vi "Autonomous Independent.vi"   [LabVIEW 2017]
doc: "This VI is called when autonomous begins, and will automatically be terminated when autonomous ends. You can carry out timed or sensor driven robot movement independently without needing to return to the caller."
uses:
  <vilib>/Rock Robotics/WPI/ThirdParty/Phoenix-LabVIEW/Motor Controller/Controls/CTRE_Phoenix_MotorControl_RemoteSourceType.ctl
  <vilib>/Rock Robotics/WPI/ThirdParty/Phoenix-LabVIEW/Motor Controller/Controls/CTRE_Phoenix_MotorControl_ControlMode.ctl
  <vilib>/Rock Robotics/WPI/Utilities/WPI_GetSetVariantRefNum.vi
  <vilib>/Rock Robotics/Network Tables/NT Read String.vi
  Robot Global Data.vi
  <vilib>/Rock Robotics/WPI/RobotDrive/WPI_RobotDriveArcadeDrive_Standard(NoSaturation).vi
  <vilib>/Rock Robotics/WPI/ThirdParty/Phoenix-LabVIEW/Motor Controller/Get/CTRE_Phoenix_MotorController_GetPulseWidthAll.vi
panel:
  # "Be sure to right-click and choose Data Operations>>Make Current Value default if you want to save the array values with the VI"
types:
  T1 = typedef "CTRE_Phoenix_MotorControl_RemoteSourceType.ctl" = enum16{"Off", "Talon SRX Selected Sensor", "Pigeon IMU Yaw", "Pigeon IMU Pitch", "Pigeon IMU Roll", "CANifier Quadrature", "CANifier PWM Input 0", "CANifier PWM Input 1", "CANifier PWM Input 2", "CANifier PWM Input 3", "Gadgeteer Pigeon Yaw", "Gadgeteer Pigeon Pitch", "Gadgeteer Pigeon Roll"}
  T2 = typedef "WPI_MotorControlDeviceRef.ctl" = cluster{"DeviceStatus":errorcluster, "Type":T3, "PWM":cluster{"PWM Channel":T4, "DeadBand":T5}, "CAN":cluster{"Device Number":u8, "SetOutput VI Ref":variant, "GetOutput VI Ref":variant, "Enable VI Ref":variant, "Disable VI Ref":variant, "Data":variant}, "Invert":bool, "DIO PWM":cluster{"PWM \"Enable\" Channel":T4, "DIOChannel":T6, "PWM Rate":dbl}}
  T3 = typedef "WPI_MotorControlType.ctl" = enum16{"PWM", "CAN", "DIO PWM"}
  T4 = typedef "FPGA_DIOPWMChannel.ctl" = enum8{"PWM 0", "PWM 1", "PWM 2", "PWM 3", "PWM 4", "PWM 5", "PWM 6", "PWM 7", "PWM 8", "PWM 9", "PWM MXP 0", "PWM MXP 1", "PWM MXP 2", "PWM MXP 3", "PWM MXP 4", "PWM MXP 5", "PWM MXP 6", "PWM MXP 7", "PWM MXP 8", "PWM MXP 9", "Invalid"}
  T5 = typedef "WPI_PWMDeadband.ctl" = cluster{"Name":string, "maxPositivePwm":i32, "minPositivePwm":i32, "centerPwm":i32, "maxNegativePwm":i32, "minNegativePwm":i32, "angularRange":u16}
  T6 = typedef "FPGA_DIOChannel.ctl" = enum8{"DIO 0", "DIO 1", "DIO 2", "DIO 3", "DIO 4", "DIO 5", "DIO 6", "DIO 7", "DIO 8", "DIO 9", "DIO MXP 0", "DIO MXP 1", "DIO MXP 2", "DIO MXP 3", "DIO MXP 4", "DIO MXP 5", "DIO MXP 6", "DIO MXP 7", "DIO MXP 8", "DIO MXP 9", "DIO MXP 10", "DIO MXP 11", "DIO MXP 12", "DIO MXP 13", "DIO MXP 14", "DIO MXP 15", "SPI Port CS1", "SPI Port CS2", "SPI Port CS3", "SPI Port MISO", "SPI Port MOSI", "Invalid"}
  T7 = typedef "WPI_AnalogChannelDevRef.ctl" = cluster{"DevStatus":errorcluster, "Analog Channel":T8}
  T8 = typedef "FPGA_AIChannel.ctl" = enum8{"AI 0", "AI 1", "AI 2", "AI 3", "AI MXP 0", "AI MXP 1", "AI MXP 2", "AI MXP 3", "Invalid"}
  T9 = typedef "WPI_SwitchDevRef.ctl" = cluster{"DevStatus":errorcluster, "DIO Channel":T6, "CntIndex":T10, "Normally Closed":bool}
  T10 = typedef "FPGA_CounterCtrSystemIndex.ctl" = enum8{"Ctr 0", "Ctr 1", "Ctr 2", "Ctr 3", "Ctr 4", "Ctr 5", "Ctr 6", "Ctr 7", "Invalid"}
  T11 = typedef "WPI_RobotDriveDevRef.ctl" = cluster{"DevStatus":errorcluster, "Motors[]":T2[], "Square Inputs":bool, "Max Output":dbl}
  T12 = typedef "CTRE_Phoenix_MotorControl_ControlMode.ctl" = u16
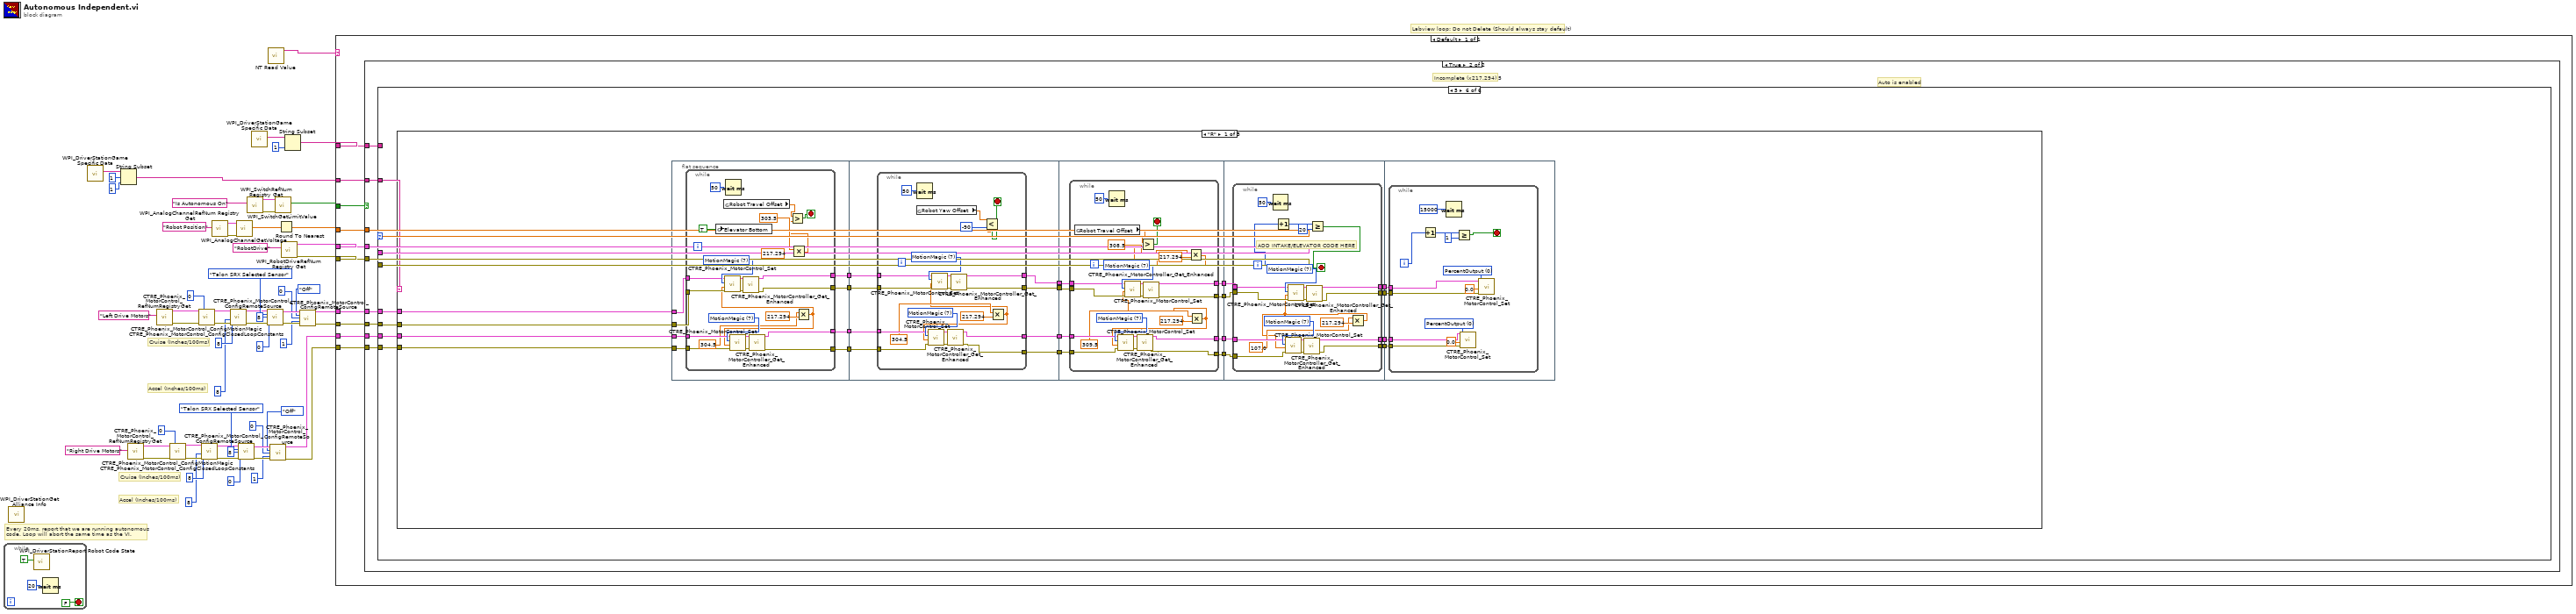
[diagram p0: block diagram]
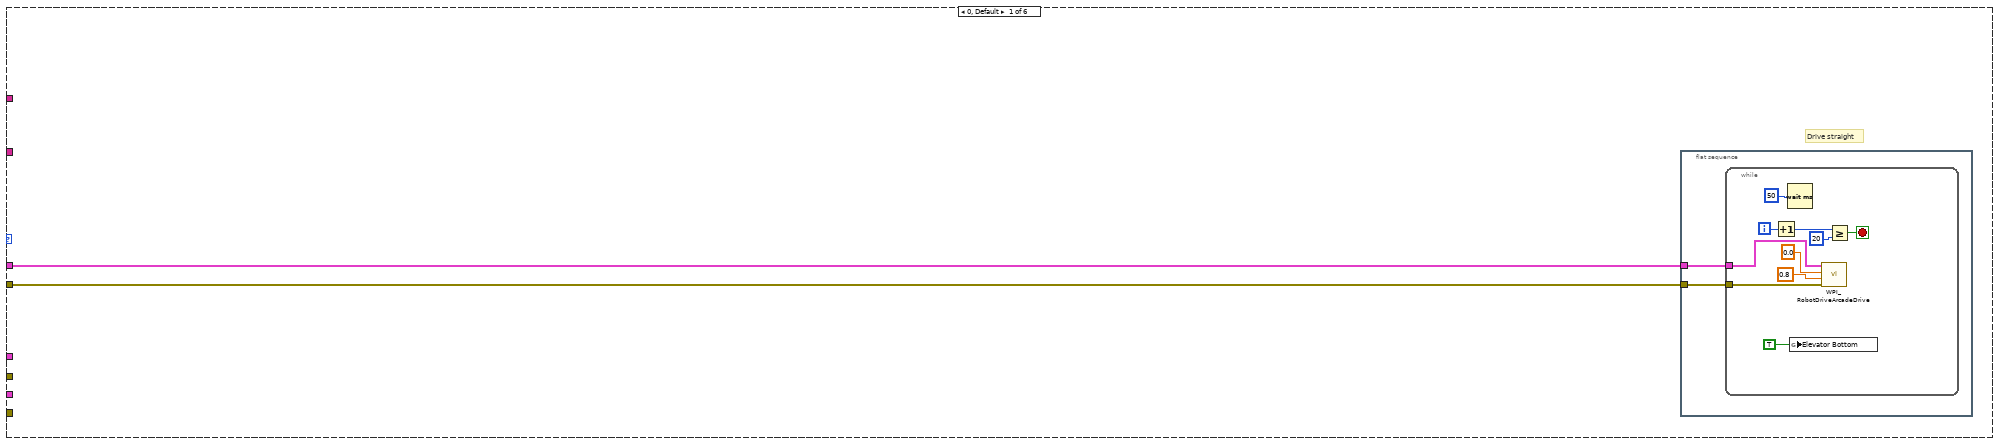
[diagram p3: hidden frame]
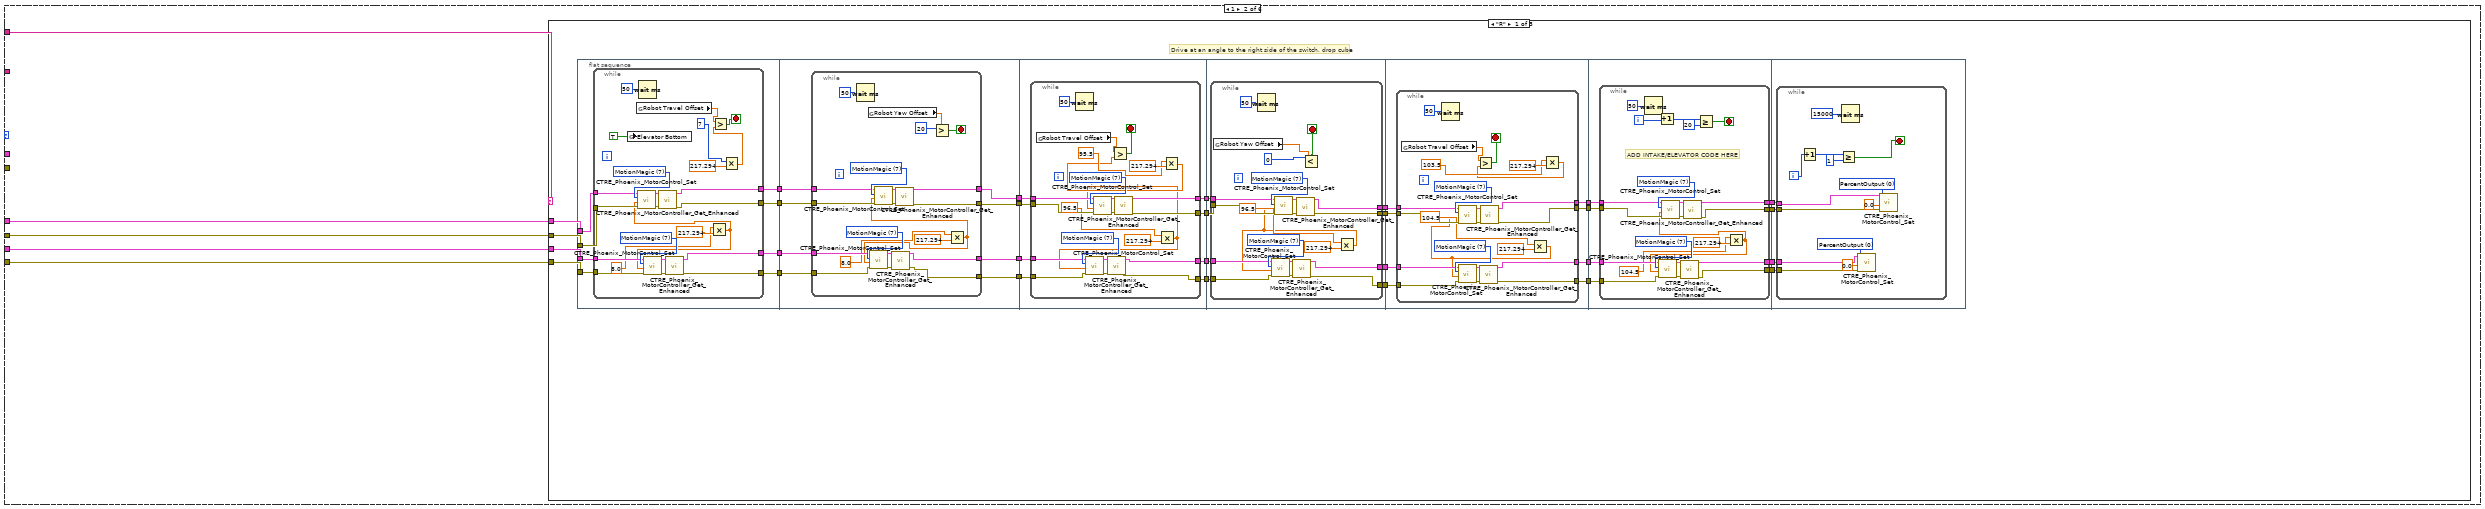
[diagram p4: hidden frame]
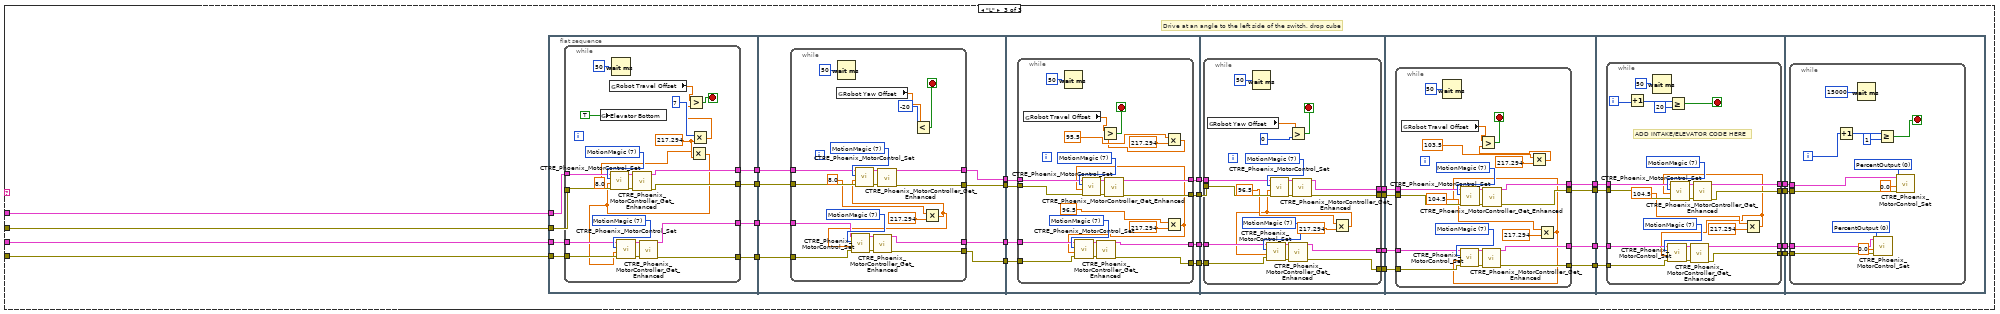
[diagram p6: hidden frame]
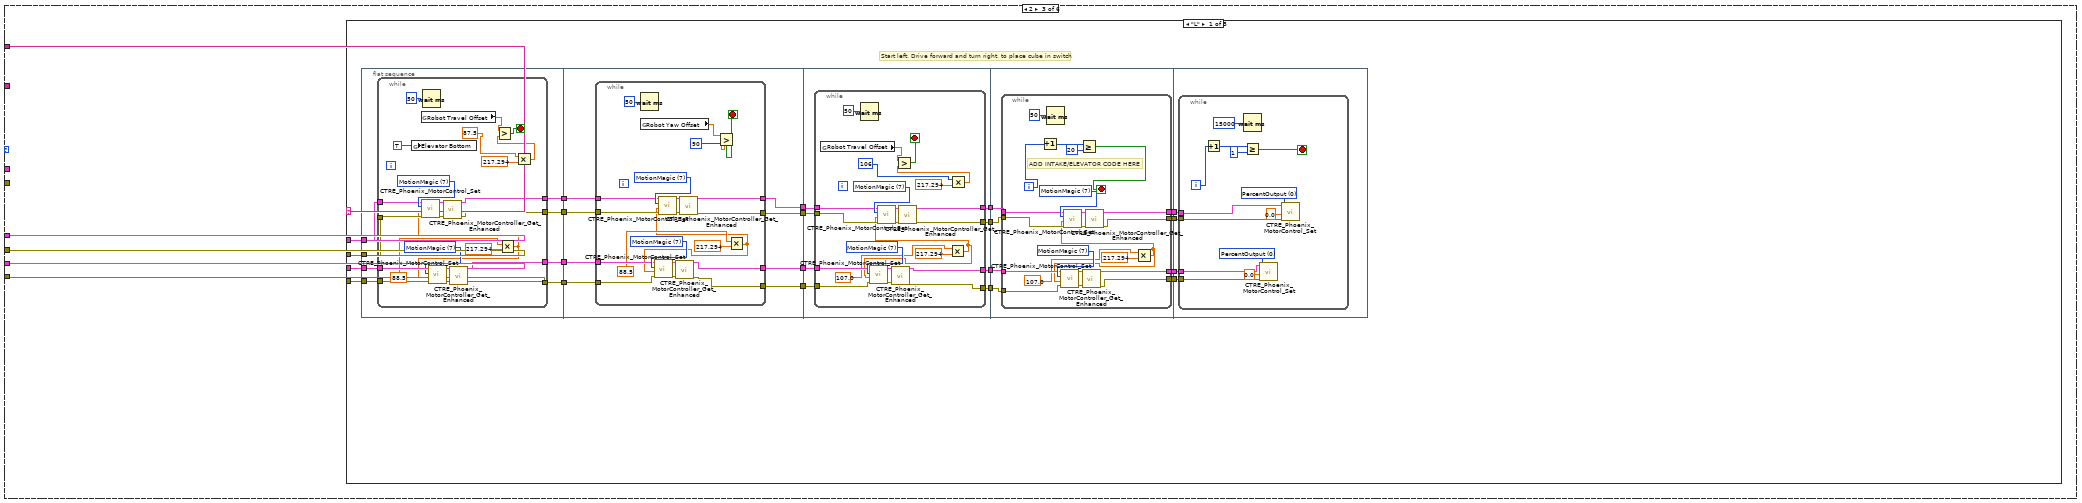
[diagram p7: hidden frame]
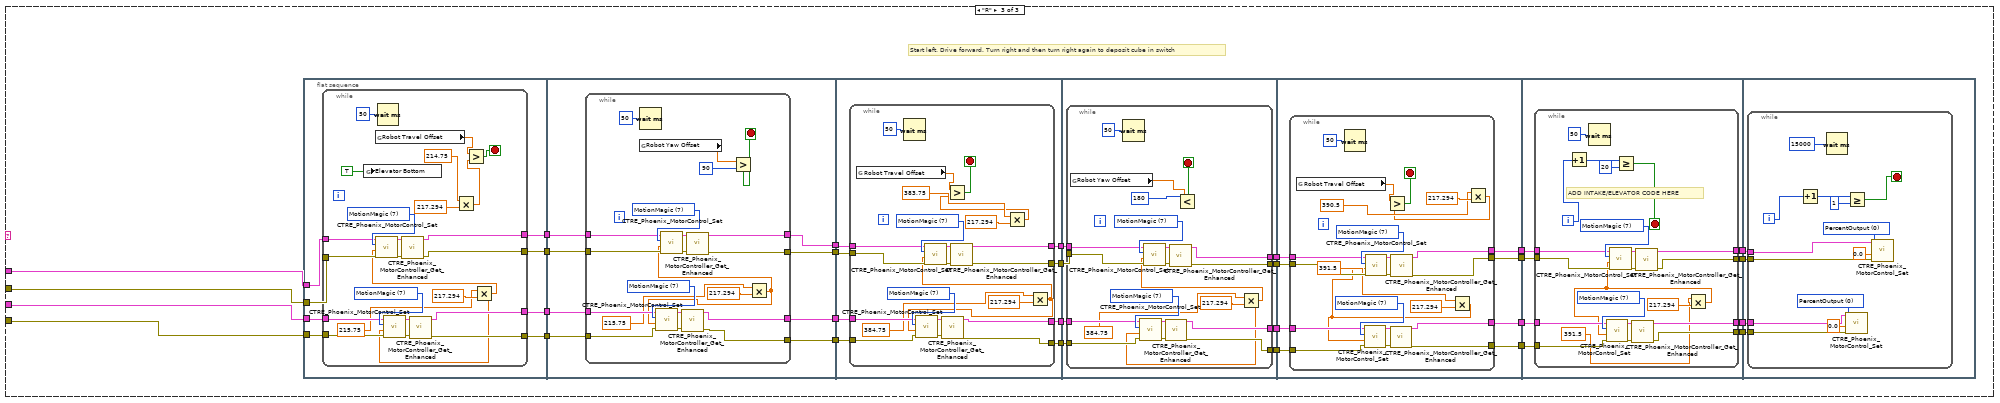
[diagram p9: hidden frame]
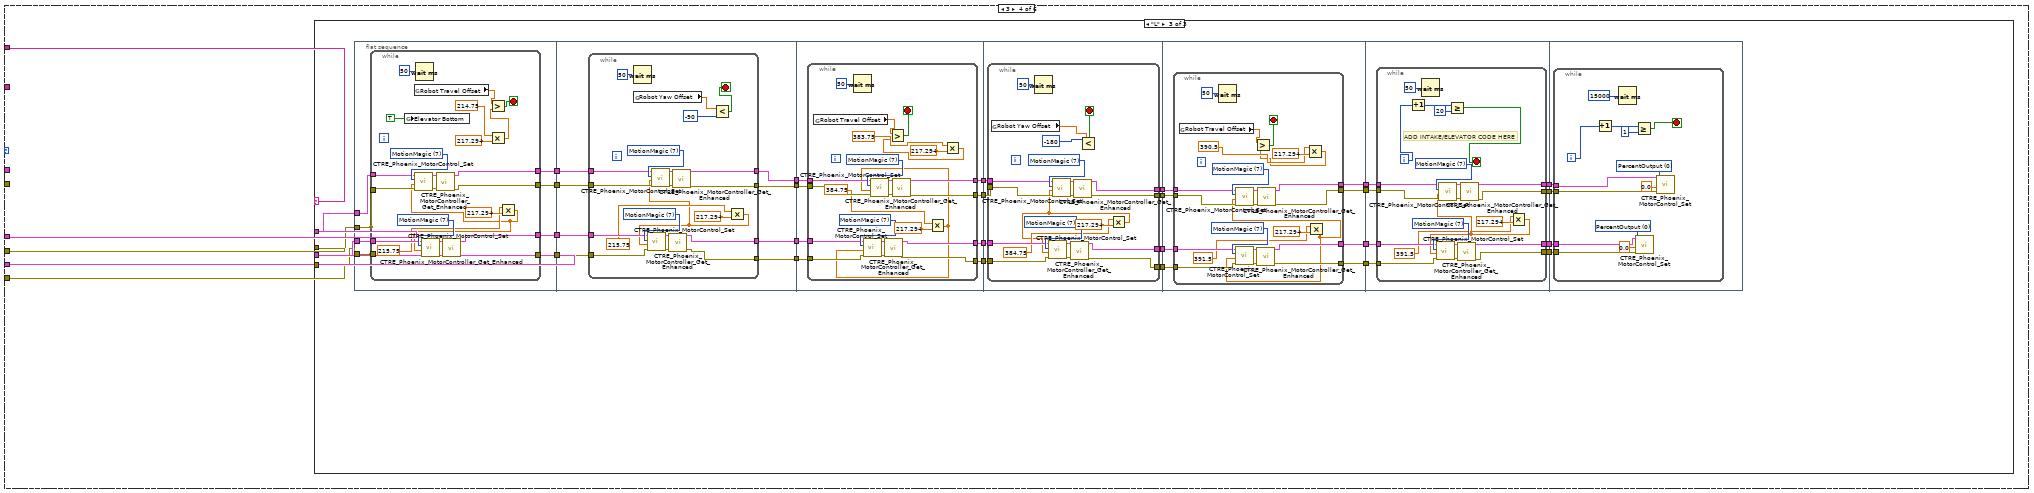
[diagram p10: hidden frame]
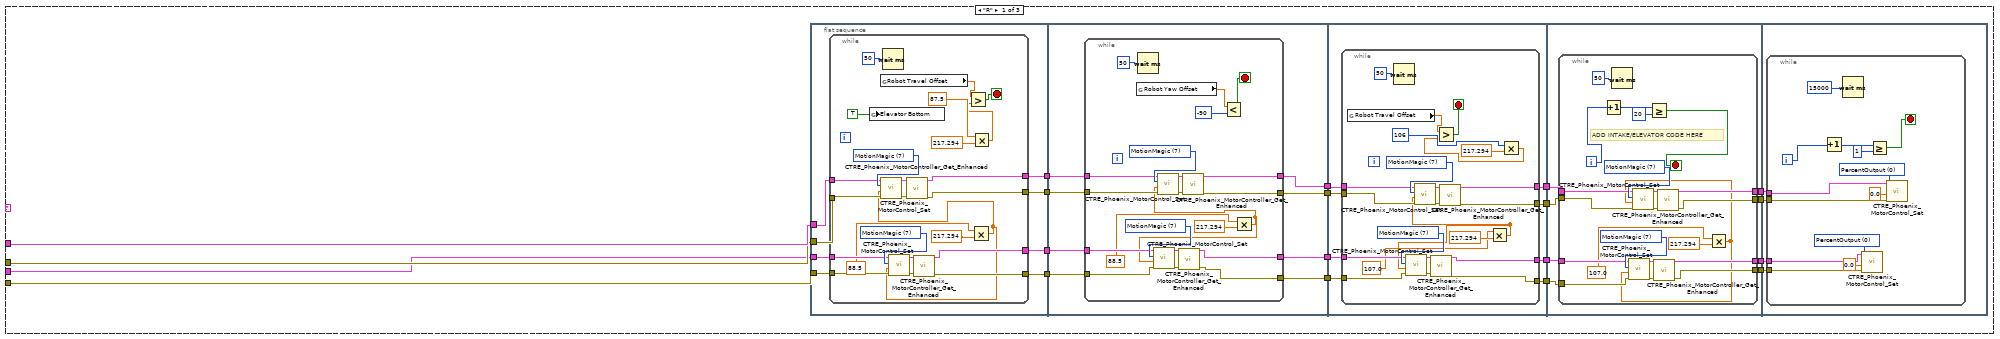
[diagram p11: hidden frame]
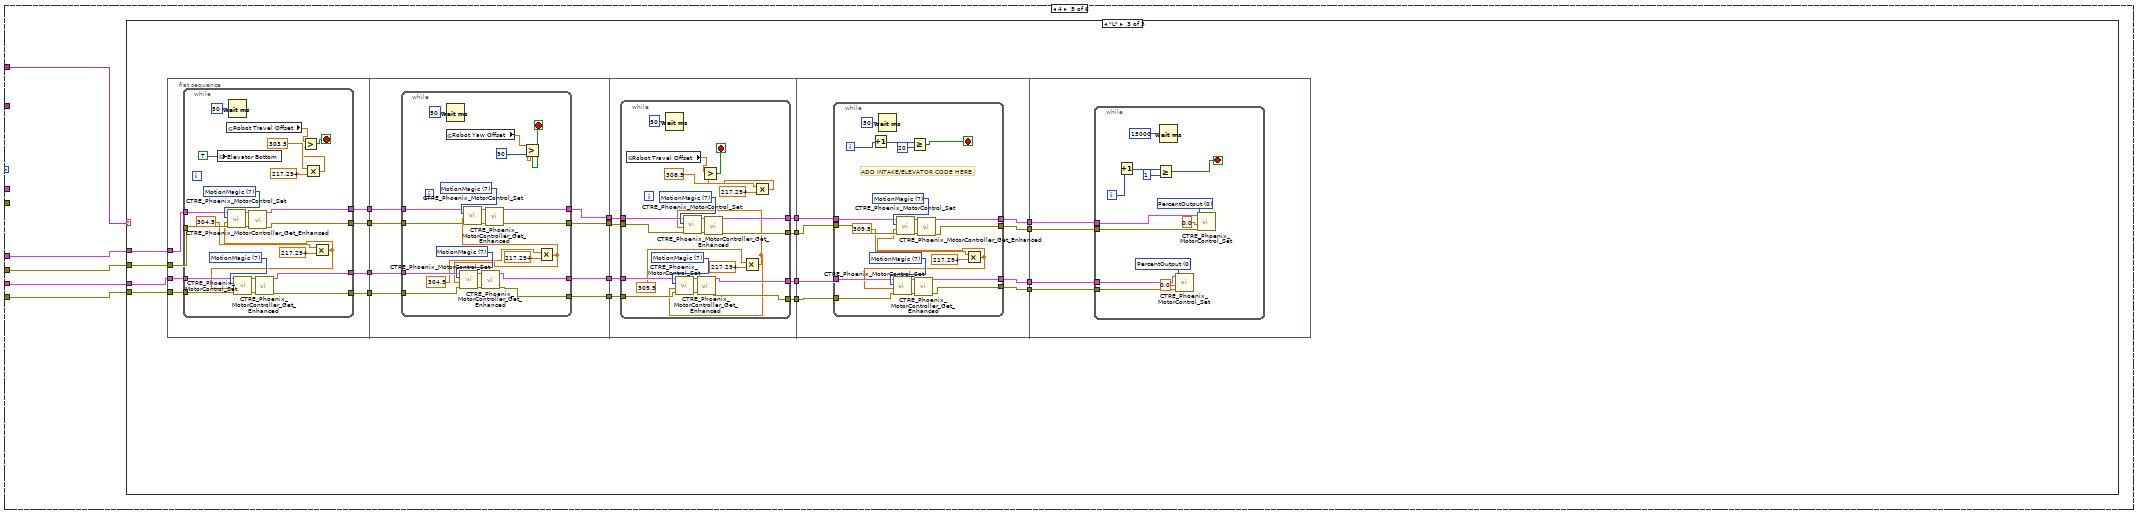
[diagram p13: hidden frame]
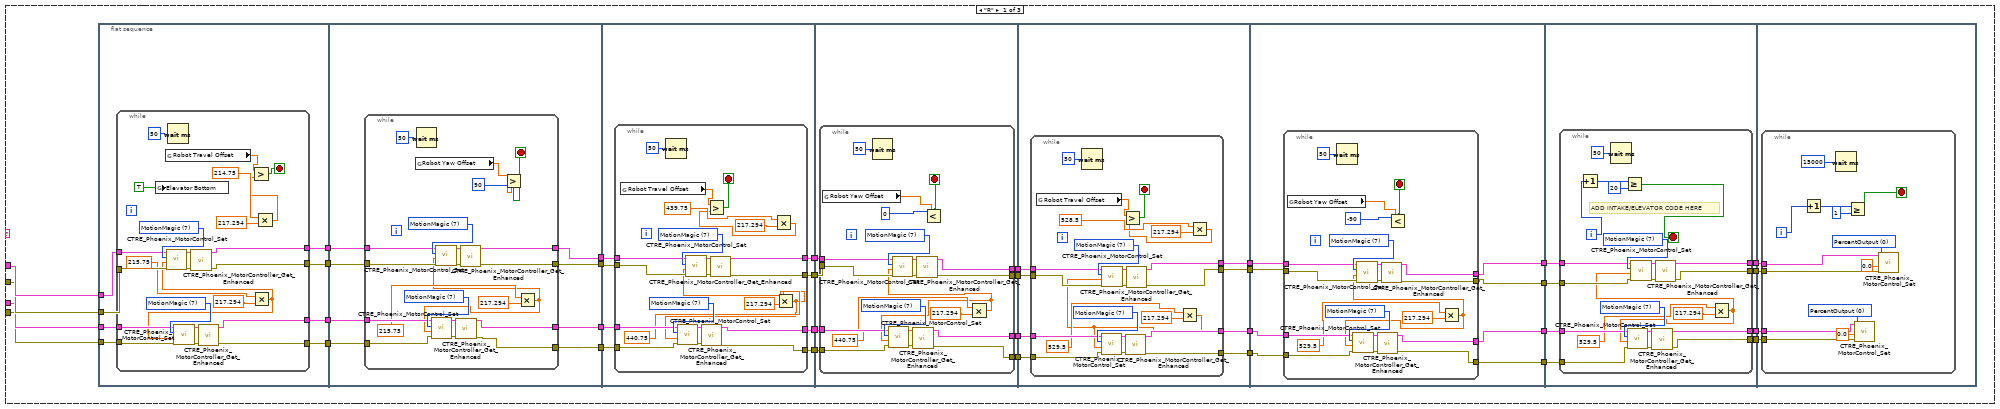
[diagram p14: hidden frame]
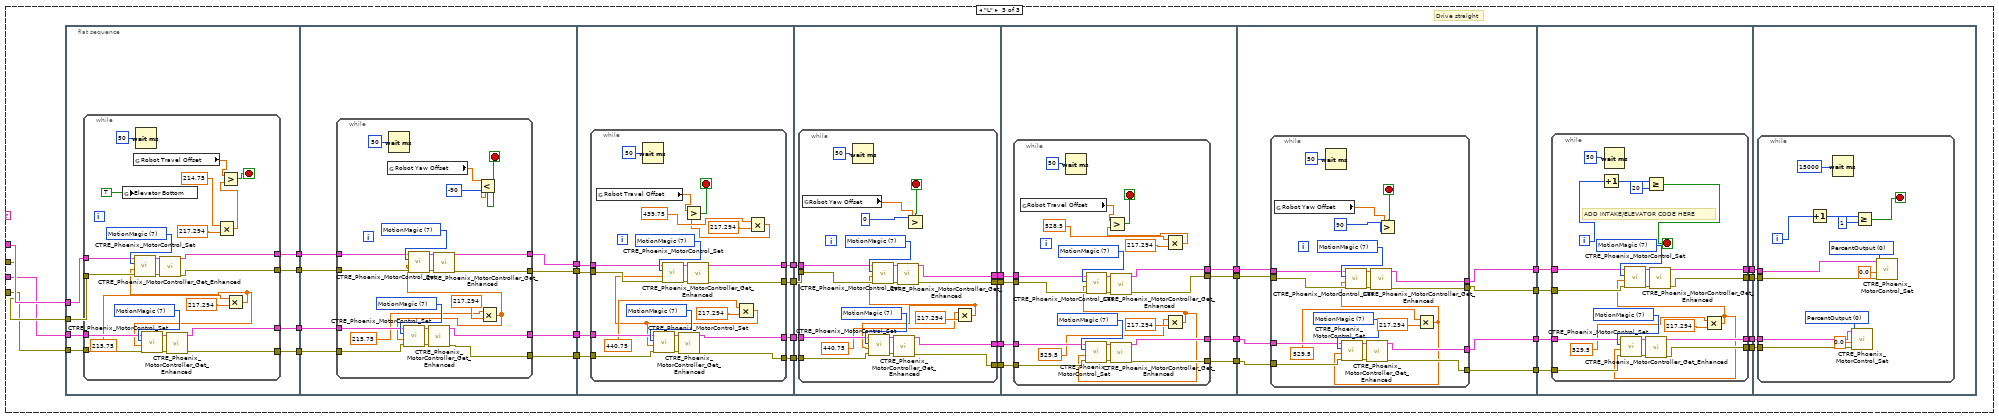
[diagram p17: hidden frame]
diagram:
  # "Cruise (Inches/100ms)"
  # "Accel (Inches/100ms)"
  # "Cruise (Inches/100ms)"
  # "Accel (Inches/100ms)"
  # "Labview loop: Do not Delete (Should always stay default)"
  # "Every 20ms, report that we are running autonomous\ncode. Loop will abort the same time as the VI."
  n1 = while {
    stop <- FALSE stop-if-true
    n2 = call <vilib>:"WPI_DriverStationReport Robot Code State.vi"("Autonomous"=TRUE) -> ()  [unwired: 10 in, 1 out]
    n3 = Wait (ms)(milliseconds to wait=u32 20) -> ()  [unwired: 1 out]
  }
  n4 = call <vilib>:"WPI_DriverStationGet Alliance Info.vi"() -> ()  [unwired: 12 out]
  n5 = call <vilib>:"WPI_DriverStationGame Specific Data.vi"() -> ("Game Specific Data"=w51:string)  [unwired: 11 in]
  n6 = String Subset(string=w51, offset (0)=1, length (rest)=1 ("length (rest)")) -> (substring=w50:string)
  n7 = call <vilib>:"CTRE_Phoenix_MotorControl_RefNumRegistryGet.vi"("refnum name"="Right Drive Motors") -> ("error out"=w19:errorcluster, "PhoenixMotorControlDevRef"=w17:T2)  [unwired: 9 in]
  n8 = call <vilib>:"CTRE_Phoenix_MotorControl_RefNumRegistryGet.vi"("refnum name"="Left Drive Motors") -> ("error out"=w39:errorcluster, "PhoenixMotorControlDevRef"=w37:T2)  [unwired: 9 in]
  n9 = call <vilib>:"CTRE_Phoenix_MotorControl_ConfigClosedLoopConstants.vi"("PhoenixMotorControlDevRef"=w17, "slotIdx"=0, "error in (no error)"=w19) -> ("PhoenixMotorControlDevRef"=w16:T2, "error out"=w18:errorcluster)  [unwired: 11 in]
  n10 = call <vilib>:"CTRE_Phoenix_MotorControl_ConfigClosedLoopConstants.vi"("PhoenixMotorControlDevRef"=w37, "slotIdx"=0, "error in (no error)"=w39) -> ("PhoenixMotorControlDevRef"=w36:T2, "error out"=w38:errorcluster)  [unwired: 11 in]
  n11 = call <vilib>:"CTRE_Phoenix_MotorControl_ConfigMotionMagic.vi"("error in (no error)"=w18, "Acceleration"=8, "Cruise Velocity"=8, "PhoenixMotorControlDevRef"=w16) -> ("error out"=w3:errorcluster, "PhoenixMotorControlDevRef"=w4:T2)  [unwired: 6 in]
  n12 = call <vilib>:"WPI_AnalogChannelRefNum Registry Get.vi"("refnum name"="Robot Position") -> ("error out"=w49:errorcluster, "AIDeviceRef"=w48:T7)  [unwired: 9 in]
  n13 = call <vilib>:"CTRE_Phoenix_MotorControl_ConfigMotionMagic.vi"("error in (no error)"=w38, "Acceleration"=8, "Cruise Velocity"=8, "PhoenixMotorControlDevRef"=w36) -> ("error out"=w23:errorcluster, "PhoenixMotorControlDevRef"=w24:T2)  [unwired: 6 in]
  n14 = call <vilib>:"WPI_AnalogChannelGetVoltage.vi"("error in (no error)"=w49, "AIDeviceRef"=w48) -> ("Voltage"=w47:dbl)  [unwired: 7 in, 2 out]
  n15 = call <vilib>:"CTRE_Phoenix_MotorControl_ConfigRemoteSource.vi"("PhoenixMotorControlDevRef"=w4, "Remote Device Type"=CTRE_Phoenix_MotorControl_RemoteSourceType."Talon SRX Selected Sensor", "Remote Device ID"=u8 8, "Source Index (0/1)"=u32 0, "error in (no error)"=w3) -> ("PhoenixMotorControlDevRef"=w9:T2, "error out"=w8:errorcluster)  [unwired: 9 in]
  n16 = call <vilib>:"WPI_SwitchRefNum Registry Get.vi"("refnum name"="Is Autonomous On") -> ("error out"=w56:errorcluster, "SwitchDevRef"=w55:T9)  [unwired: 9 in]
  n17 = call <vilib>:"WPI_DriverStationGame Specific Data.vi"() -> ("Game Specific Data"=w53:string)  [unwired: 11 in]
  n18 = call <vilib>:"CTRE_Phoenix_MotorControl_ConfigRemoteSource.vi"("PhoenixMotorControlDevRef"=w24, "Remote Device Type"=CTRE_Phoenix_MotorControl_RemoteSourceType."Talon SRX Selected Sensor", "Remote Device ID"=u8 8, "Source Index (0/1)"=u32 0, "error in (no error)"=w23) -> ("PhoenixMotorControlDevRef"=w29:T2, "error out"=w28:errorcluster)  [unwired: 9 in]
  n19 = call-poly <vilib>:"NT Read Value.vi"() -> ("String"=w59:string)  [unwired: 10 in, 1 out]
  n20 = call <vilib>:"CTRE_Phoenix_MotorControl_ConfigRemoteSource.vi"("PhoenixMotorControlDevRef"=w9, "Remote Device Type"=CTRE_Phoenix_MotorControl_RemoteSourceType."Off", "Remote Device ID"=u8 0, "Source Index (0/1)"=u32 1, "error in (no error)"=w8) -> ("PhoenixMotorControlDevRef"=w2:T2, "error out"=w1:errorcluster)  [unwired: 9 in]
  n21 = call <vilib>:"WPI_SwitchGetLimitValue.vi"("error in (no error)"=w56, "SwitchDevRef"=w55) -> ("Switch Pressed"=w45:bool)  [unwired: 7 in, 2 out]
  n22 = Round To Nearest(number=w47) -> (nearest integer value=w46:dbl)
  n23 = call <vilib>:"WPI_RobotDriveRefNum Registry Get.vi"("refnum name"="RobotDrive") -> ("error out"=w41:errorcluster, "RobotDriveDevRef"=w42:T11)  [unwired: 1 in, 8 out]
  n24 = String Subset(string=w53, length (rest)=1 ("length (rest)")) -> (substring=w57:string)  [unwired: 1 in]
  n25 = call <vilib>:"CTRE_Phoenix_MotorControl_ConfigRemoteSource.vi"("PhoenixMotorControlDevRef"=w29, "Remote Device Type"=CTRE_Phoenix_MotorControl_RemoteSourceType."Off", "Remote Device ID"=u8 0, "Source Index (0/1)"=u32 1, "error in (no error)"=w28) -> ("PhoenixMotorControlDevRef"=w22:T2, "error out"=w21:errorcluster)  [unwired: 9 in]
  n26 = case shown="Default" w59 {
    tunnel: w57 -> [w73]
    tunnel: w45 -> [w72]
    tunnel: w50 -> [w71]
    tunnel: w46 -> [w70]
    tunnel: w42 -> [w69]
    tunnel: w41 -> [w68]
    tunnel: w22 -> [w67]
    tunnel: w21 -> [w66]
    tunnel: w2 -> [w65]
    tunnel: w1 -> [w64]
    frame Default {
      n27 = case shown="True" w72 {
        tunnel: w73 -> [_ w79]
        tunnel: w71 -> [_ w74]
        tunnel: w70 -> [_ w82]
        tunnel: w69 -> [_ w81]
        tunnel: w68 -> [_ w80]
        tunnel: w67 -> [_ w78]
        tunnel: w66 -> [_ w77]
        tunnel: w65 -> [_ w76]
        tunnel: w64 -> [_ w75]
        frame False {
          # "Autonomous disabled"
          # "PUT NOTHING IN HERE\n\n(AUSTIN, THIS MEANS YOU!!!)"
        }
        frame True {
          # "Incomplete (x217.294) 5"
          # "Auto is enabled"
          n28 = case shown="5" w82 {
            tunnel: w81 -> [w84 _ _ _ _ _]
            tunnel: w80 -> [w83 _ _ _ _ _]
            tunnel: w79 -> [_ w101 w559 w950 w1341 _]
            tunnel: w78 -> [_ w100 w558 w949 w1340 w1764]
            tunnel: w77 -> [_ w99 w557 w948 w1339 w1763]
            tunnel: w76 -> [_ w98 w556 w947 w1338 w1762]
            tunnel: w75 -> [_ w97 w555 w946 w1337 w1761]
            tunnel: w74 -> [_ _ _ _ _ w1765]
            frame 0, Default {
              # "Drive straight"
              n29 = flat-sequence {
                tunnel: w84 -> [w86]
                tunnel: w83 -> [w85]
                frame #0 {
                  n30 = while {
                    tunnel: w86 -> [w91]
                    tunnel: w85 -> [w90]
                    i -> [w94]
                    stop <- w95 stop-if-true
                    n31 = Increment(x=w94) -> (x+1=w92:i32)
                    n32 = Wait (ms)(milliseconds to wait=u32 50) -> ()  [unwired: 1 out]
                    n33 = global write "Robot Global Data.vi" "Elevator Bottom"(TRUE) -> ()
                    n34 = call-poly <vilib>:"WPI_RobotDriveArcadeDrive.vi"("error in (no error)"=w90, "Y axis value"=0.8, "X axis value"=0.0, "RobotDriveDevRef"=w91) -> ()  [unwired: 5 in, 3 out]
                    n35 = Greater Or Equal?(x=w92, y=20) -> (x >= y?=w95:bool)
                  }
                }
              }
            }
            frame 1 {
              n36 = case shown="\"R\"" w101 {
                tunnel: w100 -> [w111 _ w356]
                tunnel: w99 -> [w110 _ w355]
                tunnel: w98 -> [w109 _ w336]
                tunnel: w97 -> [w108 _ w335]
                frame "R" {
                  # "Drive at an angle to the right side of the switch, drop cube"
                  n37 = flat-sequence {
                    tunnel: w111 -> [w137]
                    tunnel: w110 -> [w136]
                    tunnel: [w135] -> w129
                    tunnel: [w134] -> w128
                    tunnel: w109 -> [w133]
                    tunnel: w108 -> [w132]
                    tunnel: [w131] -> w103
                    tunnel: [w130] -> w102
                    tunnel: w129 -> [w169]
                    tunnel: w128 -> [w168]
                    tunnel: [w167] -> w127
                    tunnel: [w166] -> w126
                    tunnel: [w165] -> w105
                    tunnel: [w164] -> w104
                    tunnel: w103 -> [w163]
                    tunnel: w102 -> [w162]
                    tunnel: w127 -> [w198]
                    tunnel: w126 -> [w197]
                    tunnel: [w196] -> w125
                    tunnel: [w195] -> w124
                    tunnel: [w194] -> w107
                    tunnel: [w193] -> w106
                    tunnel: w105 -> [w192]
                    tunnel: w104 -> [w191]
                    tunnel: w125 -> [w229]
                    tunnel: w124 -> [w228]
                    tunnel: [w227] -> w123
                    tunnel: [w226] -> w122
                    tunnel: [w225] -> w121
                    tunnel: [w224] -> w120
                    tunnel: w107 -> [w223]
                    tunnel: w106 -> [w222]
                    tunnel: w123 -> [w258]
                    tunnel: w122 -> [w257]
                    tunnel: [w256] -> w119
                    tunnel: [w255] -> w118
                    tunnel: w121 -> [w254]
                    tunnel: w120 -> [w253]
                    tunnel: [w252] -> w117
                    tunnel: [w251] -> w116
                    tunnel: w119 -> [w289]
                    tunnel: w118 -> [w288]
                    tunnel: [w287] -> w115
                    tunnel: [w286] -> w114
                    tunnel: w117 -> [w285]
                    tunnel: w116 -> [w284]
                    tunnel: [w283] -> w113
                    tunnel: [w282] -> w112
                    tunnel: w115 -> [w315]
                    tunnel: w114 -> [w314]
                    tunnel: w113 -> [w313]
                    tunnel: w112 -> [w312]
                    frame #0 {
                      n38 = while {
                        tunnel: w137 -> [w156]
                        tunnel: w136 -> [w155]
                        tunnel: [w154] -> w135
                        tunnel: [w153] -> w134
                        tunnel: w133 -> [w147]
                        tunnel: w132 -> [w146]
                        tunnel: [w145] -> w131
                        tunnel: [w144] -> w130
                        stop <- w151 stop-if-true
                        w148 = T12 7 items=["PercentOutput"=0, "Position"=1, "Velocity"=2, "Current"=3, "Follower"=5, "MotionProfile"=6, "MotionMagic"=7, "MotionMagicArc"=8, "MotionProfileArc"=10, "Disabled"=15] ("Control Mode")
                        w157 = T12 7 items=["PercentOutput"=0, "Position"=1, "Velocity"=2, "Current"=3, "Follower"=5, "MotionProfile"=6, "MotionMagic"=7, "MotionMagicArc"=8, "MotionProfileArc"=10, "Disabled"=15] ("Control Mode")
                        n39 = global write "Robot Global Data.vi" "Elevator Bottom"(TRUE) -> ()
                        n40 = global read "Robot Global Data.vi" "Robot Travel Offset"() -> (w152:dbl)
                        n41 = Wait (ms)(milliseconds to wait=u32 50) -> ()  [unwired: 1 out]
                        n42 = Multiply(x=8.0 ("Output"), y=217.294) -> (x*y=w138:dbl)
                        n43 = call <vilib>:"CTRE_Phoenix_MotorControl_Set.vi"("error in (no error)"=w155, "Output"=w138, "Control Mode"=w157, "PhoenixMotorControlDevRef"=w156) -> ("error out"=w159:errorcluster, "PhoenixMotorControlDevRef"=w158:T2)  [unwired: 6 in]
                        n44 = call <vilib>:"CTRE_Phoenix_MotorControl_Set.vi"("error in (no error)"=w146, "Output"=w138, "Control Mode"=w148, "PhoenixMotorControlDevRef"=w147) -> ("error out"=w150:errorcluster, "PhoenixMotorControlDevRef"=w149:T2)  [unwired: 6 in]
                        n45 = call-poly <vilib>:"CTRE_Phoenix_MotorController_Get_Enhanced.vi"("PhoenixMotorControlDevRef"=w158, "error in"=w159) -> ("PhoenixMotorControlDevRef"=w154:T2, "error out"=w153:errorcluster)  [unwired: 8 in, 4 out]
                        n46 = call-poly <vilib>:"CTRE_Phoenix_MotorController_Get_Enhanced.vi"("PhoenixMotorControlDevRef"=w149, "error in"=w150) -> ("PhoenixMotorControlDevRef"=w145:T2, "error out"=w144:errorcluster)  [unwired: 8 in, 4 out]
                        n47 = Multiply(x=7, y=217.294) -> (x*y=w140:dbl)
                        n48 = Greater?(x=w152, y=w140) -> (0:w151:bool)
                      }
                    }
                    frame #1 {
                      n49 = while {
                        tunnel: w169 -> [w186]
                        tunnel: w168 -> [w185]
                        tunnel: [w184] -> w167
                        tunnel: [w183] -> w166
                        tunnel: [w179] -> w165
                        tunnel: [w178] -> w164
                        tunnel: w163 -> [w177]
                        tunnel: w162 -> [w176]
                        stop <- w175 stop-if-true
                        w180 = T12 7 items=["PercentOutput"=0, "Position"=1, "Velocity"=2, "Current"=3, "Follower"=5, "MotionProfile"=6, "MotionMagic"=7, "MotionMagicArc"=8, "MotionProfileArc"=10, "Disabled"=15] ("Control Mode")
                        w187 = T12 7 items=["PercentOutput"=0, "Position"=1, "Velocity"=2, "Current"=3, "Follower"=5, "MotionProfile"=6, "MotionMagic"=7, "MotionMagicArc"=8, "MotionProfileArc"=10, "Disabled"=15] ("Control Mode")
                        n50 = Wait (ms)(milliseconds to wait=u32 50) -> ()  [unwired: 1 out]
                        n51 = global read "Robot Global Data.vi" "Robot Yaw Offset"() -> (w173:dbl)
                        n52 = Greater?(x=w173, y=20) -> (0:w175:bool)
                        n53 = Multiply(x=8.0 ("Output"), y=217.294) -> (x*y=w170:dbl)
                        n54 = call <vilib>:"CTRE_Phoenix_MotorControl_Set.vi"("error in (no error)"=w176, "Output"=w170, "Control Mode"=w180, "PhoenixMotorControlDevRef"=w177) -> ("error out"=w182:errorcluster, "PhoenixMotorControlDevRef"=w181:T2)  [unwired: 6 in]
                        n55 = call <vilib>:"CTRE_Phoenix_MotorControl_Set.vi"("error in (no error)"=w185, "Output"=w170, "Control Mode"=w187, "PhoenixMotorControlDevRef"=w186) -> ("error out"=w189:errorcluster, "PhoenixMotorControlDevRef"=w188:T2)  [unwired: 6 in]
                        n56 = call-poly <vilib>:"CTRE_Phoenix_MotorController_Get_Enhanced.vi"("PhoenixMotorControlDevRef"=w181, "error in"=w182) -> ("PhoenixMotorControlDevRef"=w179:T2, "error out"=w178:errorcluster)  [unwired: 8 in, 4 out]
                        n57 = call-poly <vilib>:"CTRE_Phoenix_MotorController_Get_Enhanced.vi"("PhoenixMotorControlDevRef"=w188, "error in"=w189) -> ("PhoenixMotorControlDevRef"=w184:T2, "error out"=w183:errorcluster)  [unwired: 8 in, 4 out]
                      }
                    }
                    frame #2 {
                      n58 = while {
                        tunnel: w198 -> [w217]
                        tunnel: w197 -> [w216]
                        tunnel: [w213] -> w196
                        tunnel: [w212] -> w195
                        tunnel: [w208] -> w194
                        tunnel: [w207] -> w193
                        tunnel: w192 -> [w206]
                        tunnel: w191 -> [w205]
                        stop <- w214 stop-if-true
                        w209 = T12 7 items=["PercentOutput"=0, "Position"=1, "Velocity"=2, "Current"=3, "Follower"=5, "MotionProfile"=6, "MotionMagic"=7, "MotionMagicArc"=8, "MotionProfileArc"=10, "Disabled"=15] ("Control Mode")
                        w218 = T12 7 items=["PercentOutput"=0, "Position"=1, "Velocity"=2, "Current"=3, "Follower"=5, "MotionProfile"=6, "MotionMagic"=7, "MotionMagicArc"=8, "MotionProfileArc"=10, "Disabled"=15] ("Control Mode")
                        n59 = global read "Robot Global Data.vi" "Robot Travel Offset"() -> (w215:dbl)
                        n60 = Wait (ms)(milliseconds to wait=u32 50) -> ()  [unwired: 1 out]
                        n61 = Multiply(x=96.5 ("Output"), y=217.294) -> (x*y=w199:dbl)
                        n62 = call <vilib>:"CTRE_Phoenix_MotorControl_Set.vi"("error in (no error)"=w205, "Output"=w199, "Control Mode"=w209, "PhoenixMotorControlDevRef"=w206) -> ("error out"=w211:errorcluster, "PhoenixMotorControlDevRef"=w210:T2)  [unwired: 6 in]
                        n63 = call <vilib>:"CTRE_Phoenix_MotorControl_Set.vi"("error in (no error)"=w216, "Output"=w199, "Control Mode"=w218, "PhoenixMotorControlDevRef"=w217) -> ("error out"=w220:errorcluster, "PhoenixMotorControlDevRef"=w219:T2)  [unwired: 6 in]
                        n64 = call-poly <vilib>:"CTRE_Phoenix_MotorController_Get_Enhanced.vi"("PhoenixMotorControlDevRef"=w210, "error in"=w211) -> ("PhoenixMotorControlDevRef"=w208:T2, "error out"=w207:errorcluster)  [unwired: 8 in, 4 out]
                        n65 = call-poly <vilib>:"CTRE_Phoenix_MotorController_Get_Enhanced.vi"("PhoenixMotorControlDevRef"=w219, "error in"=w220) -> ("PhoenixMotorControlDevRef"=w213:T2, "error out"=w212:errorcluster)  [unwired: 8 in, 4 out]
                        n66 = Multiply(x=95.5, y=217.294) -> (x*y=w202:dbl)
                        n67 = Greater?(x=w215, y=w202) -> (0:w214:bool)
                      }
                    }
                    frame #3 {
                      n68 = while {
                        tunnel: w229 -> [w246]
                        tunnel: w228 -> [w245]
                        tunnel: [w244] -> w227
                        tunnel: [w243] -> w226
                        tunnel: [w239] -> w225
                        tunnel: [w238] -> w224
                        tunnel: w223 -> [w237]
                        tunnel: w222 -> [w236]
                        stop <- w233 stop-if-true
                        w240 = T12 7 items=["PercentOutput"=0, "Position"=1, "Velocity"=2, "Current"=3, "Follower"=5, "MotionProfile"=6, "MotionMagic"=7, "MotionMagicArc"=8, "MotionProfileArc"=10, "Disabled"=15] ("Control Mode")
                        w247 = T12 7 items=["PercentOutput"=0, "Position"=1, "Velocity"=2, "Current"=3, "Follower"=5, "MotionProfile"=6, "MotionMagic"=7, "MotionMagicArc"=8, "MotionProfileArc"=10, "Disabled"=15] ("Control Mode")
                        n69 = global read "Robot Global Data.vi" "Robot Yaw Offset"() -> (w234:dbl)
                        n70 = Wait (ms)(milliseconds to wait=u32 50) -> ()  [unwired: 1 out]
                        n71 = Less?(x=w234, y=0) -> (x < y?=w233:bool)
                        n72 = Multiply(x=96.5 ("Output"), y=217.294) -> (x*y=w230:dbl)
                        n73 = call <vilib>:"CTRE_Phoenix_MotorControl_Set.vi"("error in (no error)"=w236, "Output"=w230, "Control Mode"=w240, "PhoenixMotorControlDevRef"=w237) -> ("error out"=w242:errorcluster, "PhoenixMotorControlDevRef"=w241:T2)  [unwired: 6 in]
                        n74 = call <vilib>:"CTRE_Phoenix_MotorControl_Set.vi"("error in (no error)"=w245, "Output"=w230, "Control Mode"=w247, "PhoenixMotorControlDevRef"=w246) -> ("error out"=w249:errorcluster, "PhoenixMotorControlDevRef"=w248:T2)  [unwired: 6 in]
                        n75 = call-poly <vilib>:"CTRE_Phoenix_MotorController_Get_Enhanced.vi"("PhoenixMotorControlDevRef"=w241, "error in"=w242) -> ("PhoenixMotorControlDevRef"=w239:T2, "error out"=w238:errorcluster)  [unwired: 8 in, 4 out]
                        n76 = call-poly <vilib>:"CTRE_Phoenix_MotorController_Get_Enhanced.vi"("PhoenixMotorControlDevRef"=w248, "error in"=w249) -> ("PhoenixMotorControlDevRef"=w244:T2, "error out"=w243:errorcluster)  [unwired: 8 in, 4 out]
                      }
                    }
                    frame #4 {
                      n77 = while {
                        tunnel: w258 -> [w277]
                        tunnel: w257 -> [w276]
                        tunnel: [w273] -> w256
                        tunnel: [w272] -> w255
                        tunnel: w254 -> [w268]
                        tunnel: w253 -> [w267]
                        tunnel: [w266] -> w252
                        tunnel: [w265] -> w251
                        stop <- w274 stop-if-true
                        w269 = T12 7 items=["PercentOutput"=0, "Position"=1, "Velocity"=2, "Current"=3, "Follower"=5, "MotionProfile"=6, "MotionMagic"=7, "MotionMagicArc"=8, "MotionProfileArc"=10, "Disabled"=15] ("Control Mode")
                        w278 = T12 7 items=["PercentOutput"=0, "Position"=1, "Velocity"=2, "Current"=3, "Follower"=5, "MotionProfile"=6, "MotionMagic"=7, "MotionMagicArc"=8, "MotionProfileArc"=10, "Disabled"=15] ("Control Mode")
                        n78 = global read "Robot Global Data.vi" "Robot Travel Offset"() -> (w275:dbl)
                        n79 = Wait (ms)(milliseconds to wait=u32 50) -> ()  [unwired: 1 out]
                        n80 = Multiply(x=104.5 ("Output"), y=217.294) -> (x*y=w259:dbl)
                        n81 = call <vilib>:"CTRE_Phoenix_MotorControl_Set.vi"("error in (no error)"=w267, "Output"=w259, "Control Mode"=w269, "PhoenixMotorControlDevRef"=w268) -> ("error out"=w271:errorcluster, "PhoenixMotorControlDevRef"=w270:T2)  [unwired: 6 in]
                        n82 = call <vilib>:"CTRE_Phoenix_MotorControl_Set.vi"("error in (no error)"=w276, "Output"=w259, "Control Mode"=w278, "PhoenixMotorControlDevRef"=w277) -> ("error out"=w280:errorcluster, "PhoenixMotorControlDevRef"=w279:T2)  [unwired: 6 in]
                        n83 = call-poly <vilib>:"CTRE_Phoenix_MotorController_Get_Enhanced.vi"("PhoenixMotorControlDevRef"=w270, "error in"=w271) -> ("PhoenixMotorControlDevRef"=w266:T2, "error out"=w265:errorcluster)  [unwired: 8 in, 4 out]
                        n84 = call-poly <vilib>:"CTRE_Phoenix_MotorController_Get_Enhanced.vi"("PhoenixMotorControlDevRef"=w279, "error in"=w280) -> ("PhoenixMotorControlDevRef"=w273:T2, "error out"=w272:errorcluster)  [unwired: 8 in, 4 out]
                        n85 = Multiply(x=103.5, y=217.294) -> (x*y=w262:dbl)
                        n86 = Greater?(x=w275, y=w262) -> (0:w274:bool)
                      }
                    }
                    frame #5 {
                      n87 = while {
                        tunnel: w289 -> [w307]
                        tunnel: w288 -> [w306]
                        tunnel: [w305] -> w287
                        tunnel: [w304] -> w286
                        tunnel: w285 -> [w300]
                        tunnel: w284 -> [w299]
                        tunnel: [w298] -> w283
                        tunnel: [w297] -> w282
                        i -> [w293]
                        stop <- w294 stop-if-true
                        w301 = T12 7 items=["PercentOutput"=0, "Position"=1, "Velocity"=2, "Current"=3, "Follower"=5, "MotionProfile"=6, "MotionMagic"=7, "MotionMagicArc"=8, "MotionProfileArc"=10, "Disabled"=15] ("Control Mode")
                        w308 = T12 7 items=["PercentOutput"=0, "Position"=1, "Velocity"=2, "Current"=3, "Follower"=5, "MotionProfile"=6, "MotionMagic"=7, "MotionMagicArc"=8, "MotionProfileArc"=10, "Disabled"=15] ("Control Mode")
                        # "ADD INTAKE/ELEVATOR CODE HERE"
                        n88 = Wait (ms)(milliseconds to wait=u32 50) -> ()  [unwired: 1 out]
                        n89 = Increment(x=w293) -> (x+1=w295:i32)
                        n90 = Greater Or Equal?(x=w295, y=20) -> (x >= y?=w294:bool)
                        n91 = Multiply(x=104.5 ("Output"), y=217.294) -> (x*y=w290:dbl)
                        n92 = call <vilib>:"CTRE_Phoenix_MotorControl_Set.vi"("error in (no error)"=w299, "Output"=w290, "Control Mode"=w301, "PhoenixMotorControlDevRef"=w300) -> ("error out"=w303:errorcluster, "PhoenixMotorControlDevRef"=w302:T2)  [unwired: 6 in]
                        n93 = call <vilib>:"CTRE_Phoenix_MotorControl_Set.vi"("error in (no error)"=w306, "Output"=w290, "Control Mode"=w308, "PhoenixMotorControlDevRef"=w307) -> ("error out"=w310:errorcluster, "PhoenixMotorControlDevRef"=w309:T2)  [unwired: 6 in]
                        n94 = call-poly <vilib>:"CTRE_Phoenix_MotorController_Get_Enhanced.vi"("PhoenixMotorControlDevRef"=w302, "error in"=w303) -> ("PhoenixMotorControlDevRef"=w298:T2, "error out"=w297:errorcluster)  [unwired: 8 in, 4 out]
                        n95 = call-poly <vilib>:"CTRE_Phoenix_MotorController_Get_Enhanced.vi"("PhoenixMotorControlDevRef"=w309, "error in"=w310) -> ("PhoenixMotorControlDevRef"=w305:T2, "error out"=w304:errorcluster)  [unwired: 8 in, 4 out]
                      }
                    }
                    frame #6 {
                      n96 = while {
                        tunnel: w315 -> [w326]
                        tunnel: w314 -> [w325]
                        tunnel: w313 -> [w323]
                        tunnel: w312 -> [w322]
                        i -> [w316]
                        stop <- w317 stop-if-true
                        w324 = T12 0 items=["PercentOutput"=0, "Position"=1, "Velocity"=2, "Current"=3, "Follower"=5, "MotionProfile"=6, "MotionMagic"=7, "MotionMagicArc"=8, "MotionProfileArc"=10, "Disabled"=15] ("Control Mode")
                        w327 = T12 0 items=["PercentOutput"=0, "Position"=1, "Velocity"=2, "Current"=3, "Follower"=5, "MotionProfile"=6, "MotionMagic"=7, "MotionMagicArc"=8, "MotionProfileArc"=10, "Disabled"=15] ("Control Mode")
                        n97 = Increment(x=w316) -> (x+1=w318:i32)
                        n98 = Greater Or Equal?(x=w318, y=1) -> (x >= y?=w317:bool)
                        n99 = Wait (ms)(milliseconds to wait=u32 15000) -> ()  [unwired: 1 out]
                        n100 = call <vilib>:"CTRE_Phoenix_MotorControl_Set.vi"("error in (no error)"=w322, "Output"=0.0, "Control Mode"=w324, "PhoenixMotorControlDevRef"=w323) -> ()  [unwired: 6 in, 2 out]
                        n101 = call <vilib>:"CTRE_Phoenix_MotorControl_Set.vi"("error in (no error)"=w325, "Output"=0.0, "Control Mode"=w327, "PhoenixMotorControlDevRef"=w326) -> ()  [unwired: 6 in, 2 out]
                      }
                    }
                  }
                }
                frame Default {
                }
                frame "L" {
                  # "Drive at an angle to the left side of the switch, drop cube"
                  n102 = flat-sequence {
                    tunnel: w356 -> [w364]
                    tunnel: w355 -> [w363]
                    tunnel: [w362] -> w354
                    tunnel: [w361] -> w353
                    tunnel: w336 -> [w360]
                    tunnel: w335 -> [w359]
                    tunnel: [w358] -> w332
                    tunnel: [w357] -> w331
                    tunnel: w354 -> [w395]
                    tunnel: w353 -> [w394]
                    tunnel: [w393] -> w352
                    tunnel: [w392] -> w351
                    tunnel: w332 -> [w391]
                    tunnel: w331 -> [w390]
                    tunnel: [w389] -> w330
                    tunnel: [w388] -> w329
                    tunnel: w352 -> [w424]
                    tunnel: w351 -> [w423]
                    tunnel: [w422] -> w350
                    tunnel: [w421] -> w349
                    tunnel: [w420] -> w334
                    tunnel: [w419] -> w333
                    tunnel: w330 -> [w418]
                    tunnel: w329 -> [w417]
                    tunnel: w350 -> [w455]
                    tunnel: w349 -> [w454]
                    tunnel: [w453] -> w348
                    tunnel: [w452] -> w347
                    tunnel: [w451] -> w342
                    tunnel: [w450] -> w341
                    tunnel: w334 -> [w449]
                    tunnel: w333 -> [w448]
                    tunnel: w348 -> [w484]
                    tunnel: w347 -> [w483]
                    tunnel: [w482] -> w346
                    tunnel: [w481] -> w345
                    tunnel: w342 -> [w480]
                    tunnel: w341 -> [w479]
                    tunnel: [w478] -> w340
                    tunnel: [w477] -> w339
                    tunnel: w346 -> [w515]
                    tunnel: w345 -> [w514]
                    tunnel: [w513] -> w344
                    tunnel: [w512] -> w343
                    tunnel: w340 -> [w511]
                    tunnel: w339 -> [w510]
                    tunnel: [w509] -> w338
                    tunnel: [w508] -> w337
                    tunnel: w344 -> [w541]
                    tunnel: w343 -> [w540]
                    tunnel: w338 -> [w539]
                    tunnel: w337 -> [w538]
                    frame #0 {
                      n103 = while {
                        tunnel: w364 -> [w382]
                        tunnel: w363 -> [w381]
                        tunnel: [w380] -> w362
                        tunnel: [w379] -> w361
                        tunnel: w360 -> [w373]
                        tunnel: w359 -> [w372]
                        tunnel: [w371] -> w358
                        tunnel: [w370] -> w357
                        stop <- w377 stop-if-true
                        w367 = 217.294 ("y")
                        w374 = T12 7 items=["PercentOutput"=0, "Position"=1, "Velocity"=2, "Current"=3, "Follower"=5, "MotionProfile"=6, "MotionMagic"=7, "MotionMagicArc"=8, "MotionProfileArc"=10, "Disabled"=15] ("Control Mode")
                        w383 = T12 7 items=["PercentOutput"=0, "Position"=1, "Velocity"=2, "Current"=3, "Follower"=5, "MotionProfile"=6, "MotionMagic"=7, "MotionMagicArc"=8, "MotionProfileArc"=10, "Disabled"=15] ("Control Mode")
                        n104 = global write "Robot Global Data.vi" "Elevator Bottom"(TRUE) -> ()
                        n105 = global read "Robot Global Data.vi" "Robot Travel Offset"() -> (w378:dbl)
                        n106 = Wait (ms)(milliseconds to wait=u32 50) -> ()  [unwired: 1 out]
                        n107 = Multiply(x=8.0 ("Output"), y=w367) -> (x*y=w365:dbl)
                        n108 = call <vilib>:"CTRE_Phoenix_MotorControl_Set.vi"("error in (no error)"=w381, "Output"=w365, "Control Mode"=w383, "PhoenixMotorControlDevRef"=w382) -> ("error out"=w385:errorcluster, "PhoenixMotorControlDevRef"=w384:T2)  [unwired: 6 in]
                        n109 = call <vilib>:"CTRE_Phoenix_MotorControl_Set.vi"("error in (no error)"=w372, "Output"=w365, "Control Mode"=w374, "PhoenixMotorControlDevRef"=w373) -> ("error out"=w376:errorcluster, "PhoenixMotorControlDevRef"=w375:T2)  [unwired: 6 in]
                        n110 = call-poly <vilib>:"CTRE_Phoenix_MotorController_Get_Enhanced.vi"("PhoenixMotorControlDevRef"=w384, "error in"=w385) -> ("PhoenixMotorControlDevRef"=w380:T2, "error out"=w379:errorcluster)  [unwired: 8 in, 4 out]
                        n111 = call-poly <vilib>:"CTRE_Phoenix_MotorController_Get_Enhanced.vi"("PhoenixMotorControlDevRef"=w375, "error in"=w376) -> ("PhoenixMotorControlDevRef"=w371:T2, "error out"=w370:errorcluster)  [unwired: 8 in, 4 out]
                        n112 = Multiply(x=7, y=w367) -> (x*y=w368:dbl)
                        n113 = Greater?(x=w378, y=w368) -> (0:w377:bool)
                      }
                    }
                    frame #1 {
                      n114 = while {
                        tunnel: w395 -> [w412]
                        tunnel: w394 -> [w411]
                        tunnel: [w410] -> w393
                        tunnel: [w409] -> w392
                        tunnel: w391 -> [w402]
                        tunnel: w390 -> [w401]
                        tunnel: [w400] -> w389
                        tunnel: [w399] -> w388
                        stop <- w407 stop-if-true
                        w403 = T12 7 items=["PercentOutput"=0, "Position"=1, "Velocity"=2, "Current"=3, "Follower"=5, "MotionProfile"=6, "MotionMagic"=7, "MotionMagicArc"=8, "MotionProfileArc"=10, "Disabled"=15] ("Control Mode")
                        w413 = T12 7 items=["PercentOutput"=0, "Position"=1, "Velocity"=2, "Current"=3, "Follower"=5, "MotionProfile"=6, "MotionMagic"=7, "MotionMagicArc"=8, "MotionProfileArc"=10, "Disabled"=15] ("Control Mode")
                        n115 = global read "Robot Global Data.vi" "Robot Yaw Offset"() -> (w406:dbl)
                        n116 = Wait (ms)(milliseconds to wait=u32 50) -> ()  [unwired: 1 out]
                        n117 = Less?(x=w406, y=-20) -> (x < y?=w407:bool)
                        n118 = Multiply(x=8.0 ("Output"), y=217.294) -> (x*y=w396:dbl)
                        n119 = call <vilib>:"CTRE_Phoenix_MotorControl_Set.vi"("error in (no error)"=w401, "Output"=w396, "Control Mode"=w403, "PhoenixMotorControlDevRef"=w402) -> ("error out"=w405:errorcluster, "PhoenixMotorControlDevRef"=w404:T2)  [unwired: 6 in]
                        n120 = call <vilib>:"CTRE_Phoenix_MotorControl_Set.vi"("error in (no error)"=w411, "Output"=w396, "Control Mode"=w413, "PhoenixMotorControlDevRef"=w412) -> ("error out"=w415:errorcluster, "PhoenixMotorControlDevRef"=w414:T2)  [unwired: 6 in]
                        n121 = call-poly <vilib>:"CTRE_Phoenix_MotorController_Get_Enhanced.vi"("PhoenixMotorControlDevRef"=w404, "error in"=w405) -> ("PhoenixMotorControlDevRef"=w400:T2, "error out"=w399:errorcluster)  [unwired: 8 in, 4 out]
                        n122 = call-poly <vilib>:"CTRE_Phoenix_MotorController_Get_Enhanced.vi"("PhoenixMotorControlDevRef"=w414, "error in"=w415) -> ("PhoenixMotorControlDevRef"=w410:T2, "error out"=w409:errorcluster)  [unwired: 8 in, 4 out]
                      }
                    }
                    frame #2 {
                      n123 = while {
                        tunnel: w424 -> [w443]
                        tunnel: w423 -> [w442]
                        tunnel: [w439] -> w422
                        tunnel: [w438] -> w421
                        tunnel: [w434] -> w420
                        tunnel: [w433] -> w419
                        tunnel: w418 -> [w432]
                        tunnel: w417 -> [w431]
                        stop <- w440 stop-if-true
                        w435 = T12 7 items=["PercentOutput"=0, "Position"=1, "Velocity"=2, "Current"=3, "Follower"=5, "MotionProfile"=6, "MotionMagic"=7, "MotionMagicArc"=8, "MotionProfileArc"=10, "Disabled"=15] ("Control Mode")
                        w444 = T12 7 items=["PercentOutput"=0, "Position"=1, "Velocity"=2, "Current"=3, "Follower"=5, "MotionProfile"=6, "MotionMagic"=7, "MotionMagicArc"=8, "MotionProfileArc"=10, "Disabled"=15] ("Control Mode")
                        n124 = global read "Robot Global Data.vi" "Robot Travel Offset"() -> (w441:dbl)
                        n125 = Wait (ms)(milliseconds to wait=u32 50) -> ()  [unwired: 1 out]
                        n126 = Multiply(x=95.5, y=217.294) -> (x*y=w428:dbl)
                        n127 = Greater?(x=w441, y=w428) -> (0:w440:bool)
                        n128 = Multiply(x=96.5 ("Output"), y=217.294) -> (x*y=w425:dbl)
                        n129 = call <vilib>:"CTRE_Phoenix_MotorControl_Set.vi"("error in (no error)"=w431, "Output"=w425, "Control Mode"=w435, "PhoenixMotorControlDevRef"=w432) -> ("error out"=w437:errorcluster, "PhoenixMotorControlDevRef"=w436:T2)  [unwired: 6 in]
                        n130 = call <vilib>:"CTRE_Phoenix_MotorControl_Set.vi"("error in (no error)"=w442, "Output"=w425, "Control Mode"=w444, "PhoenixMotorControlDevRef"=w443) -> ("error out"=w446:errorcluster, "PhoenixMotorControlDevRef"=w445:T2)  [unwired: 6 in]
                        n131 = call-poly <vilib>:"CTRE_Phoenix_MotorController_Get_Enhanced.vi"("PhoenixMotorControlDevRef"=w436, "error in"=w437) -> ("PhoenixMotorControlDevRef"=w434:T2, "error out"=w433:errorcluster)  [unwired: 8 in, 4 out]
                        n132 = call-poly <vilib>:"CTRE_Phoenix_MotorController_Get_Enhanced.vi"("PhoenixMotorControlDevRef"=w445, "error in"=w446) -> ("PhoenixMotorControlDevRef"=w439:T2, "error out"=w438:errorcluster)  [unwired: 8 in, 4 out]
                      }
                    }
                    frame #3 {
                      n133 = while {
                        tunnel: w455 -> [w472]
                        tunnel: w454 -> [w471]
                        tunnel: [w469] -> w453
                        tunnel: [w468] -> w452
                        tunnel: [w462] -> w451
                        tunnel: [w461] -> w450
                        tunnel: w449 -> [w460]
                        tunnel: w448 -> [w459]
                        stop <- w470 stop-if-true
                        w463 = T12 7 items=["PercentOutput"=0, "Position"=1, "Velocity"=2, "Current"=3, "Follower"=5, "MotionProfile"=6, "MotionMagic"=7, "MotionMagicArc"=8, "MotionProfileArc"=10, "Disabled"=15] ("Control Mode")
                        w473 = T12 7 items=["PercentOutput"=0, "Position"=1, "Velocity"=2, "Current"=3, "Follower"=5, "MotionProfile"=6, "MotionMagic"=7, "MotionMagicArc"=8, "MotionProfileArc"=10, "Disabled"=15] ("Control Mode")
                        n134 = global read "Robot Global Data.vi" "Robot Yaw Offset"() -> (w467:dbl)
                        n135 = Wait (ms)(milliseconds to wait=u32 50) -> ()  [unwired: 1 out]
                        n136 = Greater?(x=w467, y=0) -> (0:w470:bool)
                        n137 = Multiply(x=96.5 ("Output"), y=217.294) -> (x*y=w456:dbl)
                        n138 = call <vilib>:"CTRE_Phoenix_MotorControl_Set.vi"("error in (no error)"=w459, "Output"=w456, "Control Mode"=w463, "PhoenixMotorControlDevRef"=w460) -> ("error out"=w465:errorcluster, "PhoenixMotorControlDevRef"=w464:T2)  [unwired: 6 in]
                        n139 = call <vilib>:"CTRE_Phoenix_MotorControl_Set.vi"("error in (no error)"=w471, "Output"=w456, "Control Mode"=w473, "PhoenixMotorControlDevRef"=w472) -> ("error out"=w475:errorcluster, "PhoenixMotorControlDevRef"=w474:T2)  [unwired: 6 in]
                        n140 = call-poly <vilib>:"CTRE_Phoenix_MotorController_Get_Enhanced.vi"("PhoenixMotorControlDevRef"=w464, "error in"=w465) -> ("PhoenixMotorControlDevRef"=w462:T2, "error out"=w461:errorcluster)  [unwired: 8 in, 4 out]
                        n141 = call-poly <vilib>:"CTRE_Phoenix_MotorController_Get_Enhanced.vi"("PhoenixMotorControlDevRef"=w474, "error in"=w475) -> ("PhoenixMotorControlDevRef"=w469:T2, "error out"=w468:errorcluster)  [unwired: 8 in, 4 out]
                      }
                    }
                    frame #4 {
                      n142 = while {
                        tunnel: w484 -> [w503]
                        tunnel: w483 -> [w502]
                        tunnel: [w499] -> w482
                        tunnel: [w498] -> w481
                        tunnel: w480 -> [w494]
                        tunnel: w479 -> [w493]
                        tunnel: [w492] -> w478
                        tunnel: [w491] -> w477
                        stop <- w500 stop-if-true
                        w495 = T12 7 items=["PercentOutput"=0, "Position"=1, "Velocity"=2, "Current"=3, "Follower"=5, "MotionProfile"=6, "MotionMagic"=7, "MotionMagicArc"=8, "MotionProfileArc"=10, "Disabled"=15] ("Control Mode")
                        w504 = T12 7 items=["PercentOutput"=0, "Position"=1, "Velocity"=2, "Current"=3, "Follower"=5, "MotionProfile"=6, "MotionMagic"=7, "MotionMagicArc"=8, "MotionProfileArc"=10, "Disabled"=15] ("Control Mode")
                        n143 = global read "Robot Global Data.vi" "Robot Travel Offset"() -> (w501:dbl)
                        n144 = Wait (ms)(milliseconds to wait=u32 50) -> ()  [unwired: 1 out]
                        n145 = Multiply(x=103.5, y=217.294) -> (x*y=w488:dbl)
                        n146 = Greater?(x=w501, y=w488) -> (0:w500:bool)
                        n147 = Multiply(x=104.5 ("Output"), y=217.294) -> (x*y=w485:dbl)
                        n148 = call <vilib>:"CTRE_Phoenix_MotorControl_Set.vi"("error in (no error)"=w493, "Output"=w485, "Control Mode"=w495, "PhoenixMotorControlDevRef"=w494) -> ("error out"=w497:errorcluster, "PhoenixMotorControlDevRef"=w496:T2)  [unwired: 6 in]
                        n149 = call <vilib>:"CTRE_Phoenix_MotorControl_Set.vi"("error in (no error)"=w502, "Output"=w485, "Control Mode"=w504, "PhoenixMotorControlDevRef"=w503) -> ("error out"=w506:errorcluster, "PhoenixMotorControlDevRef"=w505:T2)  [unwired: 6 in]
                        n150 = call-poly <vilib>:"CTRE_Phoenix_MotorController_Get_Enhanced.vi"("PhoenixMotorControlDevRef"=w496, "error in"=w497) -> ("PhoenixMotorControlDevRef"=w492:T2, "error out"=w491:errorcluster)  [unwired: 8 in, 4 out]
                        n151 = call-poly <vilib>:"CTRE_Phoenix_MotorController_Get_Enhanced.vi"("PhoenixMotorControlDevRef"=w505, "error in"=w506) -> ("PhoenixMotorControlDevRef"=w499:T2, "error out"=w498:errorcluster)  [unwired: 8 in, 4 out]
                      }
                    }
                    frame #5 {
                      n152 = while {
                        tunnel: w515 -> [w533]
                        tunnel: w514 -> [w532]
                        tunnel: [w531] -> w513
                        tunnel: [w530] -> w512
                        tunnel: w511 -> [w526]
                        tunnel: w510 -> [w525]
                        tunnel: [w524] -> w509
                        tunnel: [w523] -> w508
                        i -> [w519]
                        stop <- w520 stop-if-true
                        w527 = T12 7 items=["PercentOutput"=0, "Position"=1, "Velocity"=2, "Current"=3, "Follower"=5, "MotionProfile"=6, "MotionMagic"=7, "MotionMagicArc"=8, "MotionProfileArc"=10, "Disabled"=15] ("Control Mode")
                        w534 = T12 7 items=["PercentOutput"=0, "Position"=1, "Velocity"=2, "Current"=3, "Follower"=5, "MotionProfile"=6, "MotionMagic"=7, "MotionMagicArc"=8, "MotionProfileArc"=10, "Disabled"=15] ("Control Mode")
                        # "ADD INTAKE/ELEVATOR CODE HERE"
                        n153 = Increment(x=w519) -> (x+1=w521:i32)
                        n154 = Wait (ms)(milliseconds to wait=u32 50) -> ()  [unwired: 1 out]
                        n155 = Greater Or Equal?(x=w521, y=20) -> (x >= y?=w520:bool)
                        n156 = Multiply(x=104.5 ("Output"), y=217.294) -> (x*y=w516:dbl)
                        n157 = call <vilib>:"CTRE_Phoenix_MotorControl_Set.vi"("error in (no error)"=w525, "Output"=w516, "Control Mode"=w527, "PhoenixMotorControlDevRef"=w526) -> ("error out"=w529:errorcluster, "PhoenixMotorControlDevRef"=w528:T2)  [unwired: 6 in]
                        n158 = call <vilib>:"CTRE_Phoenix_MotorControl_Set.vi"("error in (no error)"=w532, "Output"=w516, "Control Mode"=w534, "PhoenixMotorControlDevRef"=w533) -> ("error out"=w536:errorcluster, "PhoenixMotorControlDevRef"=w535:T2)  [unwired: 6 in]
                        n159 = call-poly <vilib>:"CTRE_Phoenix_MotorController_Get_Enhanced.vi"("PhoenixMotorControlDevRef"=w528, "error in"=w529) -> ("PhoenixMotorControlDevRef"=w524:T2, "error out"=w523:errorcluster)  [unwired: 8 in, 4 out]
                        n160 = call-poly <vilib>:"CTRE_Phoenix_MotorController_Get_Enhanced.vi"("PhoenixMotorControlDevRef"=w535, "error in"=w536) -> ("PhoenixMotorControlDevRef"=w531:T2, "error out"=w530:errorcluster)  [unwired: 8 in, 4 out]
                      }
                    }
                    frame #6 {
                      n161 = while {
                        tunnel: w541 -> [w552]
                        tunnel: w540 -> [w551]
                        tunnel: w539 -> [w549]
                        tunnel: w538 -> [w548]
                        i -> [w544]
                        stop <- w545 stop-if-true
                        w550 = T12 0 items=["PercentOutput"=0, "Position"=1, "Velocity"=2, "Current"=3, "Follower"=5, "MotionProfile"=6, "MotionMagic"=7, "MotionMagicArc"=8, "MotionProfileArc"=10, "Disabled"=15] ("Control Mode")
                        w553 = T12 0 items=["PercentOutput"=0, "Position"=1, "Velocity"=2, "Current"=3, "Follower"=5, "MotionProfile"=6, "MotionMagic"=7, "MotionMagicArc"=8, "MotionProfileArc"=10, "Disabled"=15] ("Control Mode")
                        n162 = Increment(x=w544) -> (x+1=w546:i32)
                        n163 = Wait (ms)(milliseconds to wait=u32 15000) -> ()  [unwired: 1 out]
                        n164 = call <vilib>:"CTRE_Phoenix_MotorControl_Set.vi"("error in (no error)"=w548, "Output"=0.0, "Control Mode"=w550, "PhoenixMotorControlDevRef"=w549) -> ()  [unwired: 6 in, 2 out]
                        n165 = Greater Or Equal?(x=w546, y=1) -> (x >= y?=w545:bool)
                        n166 = call <vilib>:"CTRE_Phoenix_MotorControl_Set.vi"("error in (no error)"=w551, "Output"=0.0, "Control Mode"=w553, "PhoenixMotorControlDevRef"=w552) -> ()  [unwired: 6 in, 2 out]
                      }
                    }
                  }
                }
              }
            }
            frame 2 {
              n167 = case shown="\"L\"" w559 {
                tunnel: w558 -> [w567 _ w722]
                tunnel: w557 -> [w566 _ w721]
                tunnel: w556 -> [w565 _ w720]
                tunnel: w555 -> [w564 _ w719]
                frame "L" {
                  # "Start left. Drive forward and turn right, to place cube in switch"
                  n168 = flat-sequence {
                    tunnel: w567 -> [w587]
                    tunnel: w566 -> [w586]
                    tunnel: [w585] -> w579
                    tunnel: [w584] -> w578
                    tunnel: w565 -> [w583]
                    tunnel: w564 -> [w582]
                    tunnel: [w581] -> w577
                    tunnel: [w580] -> w576
                    tunnel: w579 -> [w619]
                    tunnel: w578 -> [w618]
                    tunnel: [w617] -> w575
                    tunnel: [w616] -> w574
                    tunnel: [w615] -> w573
                    tunnel: [w614] -> w572
                    tunnel: w577 -> [w613]
                    tunnel: w576 -> [w612]
                    tunnel: w575 -> [w648]
                    tunnel: w574 -> [w647]
                    tunnel: w573 -> [w646]
                    tunnel: w572 -> [w645]
                    tunnel: [w644] -> w563
                    tunnel: [w643] -> w562
                    tunnel: [w642] -> w561
                    tunnel: [w641] -> w560
                    tunnel: [w679] -> w571
                    tunnel: [w678] -> w570
                    tunnel: [w677] -> w569
                    tunnel: [w676] -> w568
                    tunnel: w563 -> [w675]
                    tunnel: w562 -> [w674]
                    tunnel: w561 -> [w673]
                    tunnel: w560 -> [w672]
                    tunnel: w571 -> [w705]
                    tunnel: w570 -> [w704]
                    tunnel: w569 -> [w703]
                    tunnel: w568 -> [w702]
                    frame #0 {
                      n169 = while {
                        tunnel: w587 -> [w606]
                        tunnel: w586 -> [w605]
                        tunnel: [w604] -> w585
                        tunnel: [w603] -> w584
                        tunnel: w583 -> [w597]
                        tunnel: w582 -> [w596]
                        tunnel: [w595] -> w581
                        tunnel: [w594] -> w580
                        stop <- w601 stop-if-true
                        w598 = T12 7 items=["PercentOutput"=0, "Position"=1, "Velocity"=2, "Current"=3, "Follower"=5, "MotionProfile"=6, "MotionMagic"=7, "MotionMagicArc"=8, "MotionProfileArc"=10, "Disabled"=15] ("Control Mode")
                        w607 = T12 7 items=["PercentOutput"=0, "Position"=1, "Velocity"=2, "Current"=3, "Follower"=5, "MotionProfile"=6, "MotionMagic"=7, "MotionMagicArc"=8, "MotionProfileArc"=10, "Disabled"=15] ("Control Mode")
                        n170 = global write "Robot Global Data.vi" "Elevator Bottom"(TRUE) -> ()
                        n171 = global read "Robot Global Data.vi" "Robot Travel Offset"() -> (w602:dbl)
                        n172 = Wait (ms)(milliseconds to wait=u32 50) -> ()  [unwired: 1 out]
                        n173 = Multiply(x=88.5 ("Output"), y=217.294) -> (x*y=w588:dbl)
                        n174 = call <vilib>:"CTRE_Phoenix_MotorControl_Set.vi"("error in (no error)"=w605, "Output"=w588, "Control Mode"=w607, "PhoenixMotorControlDevRef"=w606) -> ("error out"=w609:errorcluster, "PhoenixMotorControlDevRef"=w608:T2)  [unwired: 6 in]
                        n175 = call <vilib>:"CTRE_Phoenix_MotorControl_Set.vi"("error in (no error)"=w596, "Output"=w588, "Control Mode"=w598, "PhoenixMotorControlDevRef"=w597) -> ("error out"=w600:errorcluster, "PhoenixMotorControlDevRef"=w599:T2)  [unwired: 6 in]
                        n176 = call-poly <vilib>:"CTRE_Phoenix_MotorController_Get_Enhanced.vi"("PhoenixMotorControlDevRef"=w608, "error in"=w609) -> ("PhoenixMotorControlDevRef"=w604:T2, "error out"=w603:errorcluster)  [unwired: 8 in, 4 out]
                        n177 = call-poly <vilib>:"CTRE_Phoenix_MotorController_Get_Enhanced.vi"("PhoenixMotorControlDevRef"=w599, "error in"=w600) -> ("PhoenixMotorControlDevRef"=w595:T2, "error out"=w594:errorcluster)  [unwired: 8 in, 4 out]
                        n178 = Multiply(x=87.5, y=217.294) -> (x*y=w591:dbl)
                        n179 = Greater?(x=w602, y=w591) -> (0:w601:bool)
                      }
                    }
                    frame #1 {
                      n180 = while {
                        tunnel: w619 -> [w636]
                        tunnel: w618 -> [w635]
                        tunnel: [w634] -> w617
                        tunnel: [w633] -> w616
                        tunnel: [w629] -> w615
                        tunnel: [w628] -> w614
                        tunnel: w613 -> [w627]
                        tunnel: w612 -> [w626]
                        stop <- w625 stop-if-true
                        w630 = T12 7 items=["PercentOutput"=0, "Position"=1, "Velocity"=2, "Current"=3, "Follower"=5, "MotionProfile"=6, "MotionMagic"=7, "MotionMagicArc"=8, "MotionProfileArc"=10, "Disabled"=15] ("Control Mode")
                        w637 = T12 7 items=["PercentOutput"=0, "Position"=1, "Velocity"=2, "Current"=3, "Follower"=5, "MotionProfile"=6, "MotionMagic"=7, "MotionMagicArc"=8, "MotionProfileArc"=10, "Disabled"=15] ("Control Mode")
                        n181 = global read "Robot Global Data.vi" "Robot Yaw Offset"() -> (w623:dbl)
                        n182 = Wait (ms)(milliseconds to wait=u32 50) -> ()  [unwired: 1 out]
                        n183 = Greater?(x=w623, y=90) -> (0:w625:bool)
                        n184 = Multiply(x=88.5 ("Output"), y=217.294) -> (x*y=w620:dbl)
                        n185 = call <vilib>:"CTRE_Phoenix_MotorControl_Set.vi"("error in (no error)"=w626, "Output"=w620, "Control Mode"=w630, "PhoenixMotorControlDevRef"=w627) -> ("error out"=w632:errorcluster, "PhoenixMotorControlDevRef"=w631:T2)  [unwired: 6 in]
                        n186 = call <vilib>:"CTRE_Phoenix_MotorControl_Set.vi"("error in (no error)"=w635, "Output"=w620, "Control Mode"=w637, "PhoenixMotorControlDevRef"=w636) -> ("error out"=w639:errorcluster, "PhoenixMotorControlDevRef"=w638:T2)  [unwired: 6 in]
                        n187 = call-poly <vilib>:"CTRE_Phoenix_MotorController_Get_Enhanced.vi"("PhoenixMotorControlDevRef"=w631, "error in"=w632) -> ("PhoenixMotorControlDevRef"=w629:T2, "error out"=w628:errorcluster)  [unwired: 8 in, 4 out]
                        n188 = call-poly <vilib>:"CTRE_Phoenix_MotorController_Get_Enhanced.vi"("PhoenixMotorControlDevRef"=w638, "error in"=w639) -> ("PhoenixMotorControlDevRef"=w634:T2, "error out"=w633:errorcluster)  [unwired: 8 in, 4 out]
                      }
                    }
                    frame #2 {
                      n189 = while {
                        tunnel: w648 -> [w667]
                        tunnel: w647 -> [w666]
                        tunnel: [w663] -> w644
                        tunnel: [w662] -> w642
                        tunnel: [w658] -> w643
                        tunnel: [w657] -> w641
                        tunnel: w646 -> [w656]
                        tunnel: w645 -> [w655]
                        stop <- w664 stop-if-true
                        w659 = T12 7 items=["PercentOutput"=0, "Position"=1, "Velocity"=2, "Current"=3, "Follower"=5, "MotionProfile"=6, "MotionMagic"=7, "MotionMagicArc"=8, "MotionProfileArc"=10, "Disabled"=15] ("Control Mode")
                        w668 = T12 7 items=["PercentOutput"=0, "Position"=1, "Velocity"=2, "Current"=3, "Follower"=5, "MotionProfile"=6, "MotionMagic"=7, "MotionMagicArc"=8, "MotionProfileArc"=10, "Disabled"=15] ("Control Mode")
                        n190 = global read "Robot Global Data.vi" "Robot Travel Offset"() -> (w665:dbl)
                        n191 = Wait (ms)(milliseconds to wait=u32 50) -> ()  [unwired: 1 out]
                        n192 = Multiply(x=107.0 ("Output"), y=217.294) -> (x*y=w649:dbl)
                        n193 = call <vilib>:"CTRE_Phoenix_MotorControl_Set.vi"("error in (no error)"=w655, "Output"=w649, "Control Mode"=w659, "PhoenixMotorControlDevRef"=w656) -> ("error out"=w661:errorcluster, "PhoenixMotorControlDevRef"=w660:T2)  [unwired: 6 in]
                        n194 = call <vilib>:"CTRE_Phoenix_MotorControl_Set.vi"("error in (no error)"=w666, "Output"=w649, "Control Mode"=w668, "PhoenixMotorControlDevRef"=w667) -> ("error out"=w670:errorcluster, "PhoenixMotorControlDevRef"=w669:T2)  [unwired: 6 in]
                        n195 = call-poly <vilib>:"CTRE_Phoenix_MotorController_Get_Enhanced.vi"("PhoenixMotorControlDevRef"=w660, "error in"=w661) -> ("PhoenixMotorControlDevRef"=w658:T2, "error out"=w657:errorcluster)  [unwired: 8 in, 4 out]
                        n196 = call-poly <vilib>:"CTRE_Phoenix_MotorController_Get_Enhanced.vi"("PhoenixMotorControlDevRef"=w669, "error in"=w670) -> ("PhoenixMotorControlDevRef"=w663:T2, "error out"=w662:errorcluster)  [unwired: 8 in, 4 out]
                        n197 = Multiply(x=106, y=217.294) -> (x*y=w652:dbl)
                        n198 = Greater?(x=w665, y=w652) -> (0:w664:bool)
                      }
                    }
                    frame #3 {
                      n199 = while {
                        tunnel: w675 -> [w697]
                        tunnel: w673 -> [w696]
                        tunnel: [w695] -> w679
                        tunnel: [w694] -> w678
                        tunnel: w674 -> [w690]
                        tunnel: w672 -> [w689]
                        tunnel: [w688] -> w677
                        tunnel: [w687] -> w676
                        i -> [w683]
                        stop <- w684 stop-if-true
                        w691 = T12 7 items=["PercentOutput"=0, "Position"=1, "Velocity"=2, "Current"=3, "Follower"=5, "MotionProfile"=6, "MotionMagic"=7, "MotionMagicArc"=8, "MotionProfileArc"=10, "Disabled"=15] ("Control Mode")
                        w698 = T12 7 items=["PercentOutput"=0, "Position"=1, "Velocity"=2, "Current"=3, "Follower"=5, "MotionProfile"=6, "MotionMagic"=7, "MotionMagicArc"=8, "MotionProfileArc"=10, "Disabled"=15] ("Control Mode")
                        # "ADD INTAKE/ELEVATOR CODE HERE"
                        n200 = Increment(x=w683) -> (x+1=w685:i32)
                        n201 = Wait (ms)(milliseconds to wait=u32 50) -> ()  [unwired: 1 out]
                        n202 = Greater Or Equal?(x=w685, y=20) -> (x >= y?=w684:bool)
                        n203 = Multiply(x=107.0 ("Output"), y=217.294) -> (x*y=w680:dbl)
                        n204 = call <vilib>:"CTRE_Phoenix_MotorControl_Set.vi"("error in (no error)"=w689, "Output"=w680, "Control Mode"=w691, "PhoenixMotorControlDevRef"=w690) -> ("error out"=w693:errorcluster, "PhoenixMotorControlDevRef"=w692:T2)  [unwired: 6 in]
                        n205 = call <vilib>:"CTRE_Phoenix_MotorControl_Set.vi"("error in (no error)"=w696, "Output"=w680, "Control Mode"=w698, "PhoenixMotorControlDevRef"=w697) -> ("error out"=w700:errorcluster, "PhoenixMotorControlDevRef"=w699:T2)  [unwired: 6 in]
                        n206 = call-poly <vilib>:"CTRE_Phoenix_MotorController_Get_Enhanced.vi"("PhoenixMotorControlDevRef"=w692, "error in"=w693) -> ("PhoenixMotorControlDevRef"=w688:T2, "error out"=w687:errorcluster)  [unwired: 8 in, 4 out]
                        n207 = call-poly <vilib>:"CTRE_Phoenix_MotorController_Get_Enhanced.vi"("PhoenixMotorControlDevRef"=w699, "error in"=w700) -> ("PhoenixMotorControlDevRef"=w695:T2, "error out"=w694:errorcluster)  [unwired: 8 in, 4 out]
                      }
                    }
                    frame #4 {
                      n208 = while {
                        tunnel: w705 -> [w716]
                        tunnel: w704 -> [w715]
                        tunnel: w703 -> [w713]
                        tunnel: w702 -> [w712]
                        i -> [w708]
                        stop <- w709 stop-if-true
                        w714 = T12 0 items=["PercentOutput"=0, "Position"=1, "Velocity"=2, "Current"=3, "Follower"=5, "MotionProfile"=6, "MotionMagic"=7, "MotionMagicArc"=8, "MotionProfileArc"=10, "Disabled"=15] ("Control Mode")
                        w717 = T12 0 items=["PercentOutput"=0, "Position"=1, "Velocity"=2, "Current"=3, "Follower"=5, "MotionProfile"=6, "MotionMagic"=7, "MotionMagicArc"=8, "MotionProfileArc"=10, "Disabled"=15] ("Control Mode")
                        n209 = Increment(x=w708) -> (x+1=w710:i32)
                        n210 = Wait (ms)(milliseconds to wait=u32 15000) -> ()  [unwired: 1 out]
                        n211 = Greater Or Equal?(x=w710, y=1) -> (x >= y?=w709:bool)
                        n212 = call <vilib>:"CTRE_Phoenix_MotorControl_Set.vi"("error in (no error)"=w712, "Output"=0.0, "Control Mode"=w714, "PhoenixMotorControlDevRef"=w713) -> ()  [unwired: 6 in, 2 out]
                        n213 = call <vilib>:"CTRE_Phoenix_MotorControl_Set.vi"("error in (no error)"=w715, "Output"=0.0, "Control Mode"=w717, "PhoenixMotorControlDevRef"=w716) -> ()  [unwired: 6 in, 2 out]
                      }
                    }
                  }
                }
                frame Default {
                }
                frame "R" {
                  # "Start left. Drive forward. Turn right and then turn right again to deposit cube in switch"
                  n214 = flat-sequence {
                    tunnel: w722 -> [w754]
                    tunnel: w721 -> [w753]
                    tunnel: [w752] -> w746
                    tunnel: [w751] -> w745
                    tunnel: w720 -> [w750]
                    tunnel: w719 -> [w749]
                    tunnel: [w748] -> w744
                    tunnel: [w747] -> w743
                    tunnel: w746 -> [w786]
                    tunnel: w745 -> [w785]
                    tunnel: [w784] -> w742
                    tunnel: [w783] -> w741
                    tunnel: [w782] -> w740
                    tunnel: [w781] -> w739
                    tunnel: w744 -> [w780]
                    tunnel: w743 -> [w779]
                    tunnel: w742 -> [w815]
                    tunnel: w741 -> [w814]
                    tunnel: [w813] -> w738
                    tunnel: [w812] -> w737
                    tunnel: [w811] -> w736
                    tunnel: [w810] -> w735
                    tunnel: w740 -> [w809]
                    tunnel: w739 -> [w808]
                    tunnel: w738 -> [w846]
                    tunnel: w737 -> [w845]
                    tunnel: [w844] -> w734
                    tunnel: [w843] -> w733
                    tunnel: [w842] -> w732
                    tunnel: [w841] -> w731
                    tunnel: w736 -> [w840]
                    tunnel: w735 -> [w839]
                    tunnel: w734 -> [w875]
                    tunnel: w733 -> [w874]
                    tunnel: [w873] -> w730
                    tunnel: [w872] -> w729
                    tunnel: w732 -> [w871]
                    tunnel: w731 -> [w870]
                    tunnel: [w869] -> w728
                    tunnel: [w868] -> w727
                    tunnel: w730 -> [w906]
                    tunnel: w729 -> [w905]
                    tunnel: [w904] -> w726
                    tunnel: [w903] -> w725
                    tunnel: w728 -> [w902]
                    tunnel: w727 -> [w901]
                    tunnel: [w900] -> w724
                    tunnel: [w899] -> w723
                    tunnel: w726 -> [w932]
                    tunnel: w725 -> [w931]
                    tunnel: w724 -> [w930]
                    tunnel: w723 -> [w929]
                    frame #0 {
                      n215 = while {
                        tunnel: w754 -> [w773]
                        tunnel: w753 -> [w772]
                        tunnel: [w771] -> w752
                        tunnel: [w770] -> w751
                        tunnel: w750 -> [w764]
                        tunnel: w749 -> [w763]
                        tunnel: [w762] -> w748
                        tunnel: [w761] -> w747
                        stop <- w768 stop-if-true
                        w765 = T12 7 items=["PercentOutput"=0, "Position"=1, "Velocity"=2, "Current"=3, "Follower"=5, "MotionProfile"=6, "MotionMagic"=7, "MotionMagicArc"=8, "MotionProfileArc"=10, "Disabled"=15] ("Control Mode")
                        w774 = T12 7 items=["PercentOutput"=0, "Position"=1, "Velocity"=2, "Current"=3, "Follower"=5, "MotionProfile"=6, "MotionMagic"=7, "MotionMagicArc"=8, "MotionProfileArc"=10, "Disabled"=15] ("Control Mode")
                        n216 = global write "Robot Global Data.vi" "Elevator Bottom"(TRUE) -> ()
                        n217 = global read "Robot Global Data.vi" "Robot Travel Offset"() -> (w769:dbl)
                        n218 = Wait (ms)(milliseconds to wait=u32 50) -> ()  [unwired: 1 out]
                        n219 = Multiply(x=214.75, y=217.294) -> (x*y=w758:dbl)
                        n220 = Greater?(x=w769, y=w758) -> (0:w768:bool)
                        n221 = Multiply(x=215.75 ("Output"), y=217.294) -> (x*y=w755:dbl)
                        n222 = call <vilib>:"CTRE_Phoenix_MotorControl_Set.vi"("error in (no error)"=w772, "Output"=w755, "Control Mode"=w774, "PhoenixMotorControlDevRef"=w773) -> ("error out"=w776:errorcluster, "PhoenixMotorControlDevRef"=w775:T2)  [unwired: 6 in]
                        n223 = call <vilib>:"CTRE_Phoenix_MotorControl_Set.vi"("error in (no error)"=w763, "Output"=w755, "Control Mode"=w765, "PhoenixMotorControlDevRef"=w764) -> ("error out"=w767:errorcluster, "PhoenixMotorControlDevRef"=w766:T2)  [unwired: 6 in]
                        n224 = call-poly <vilib>:"CTRE_Phoenix_MotorController_Get_Enhanced.vi"("PhoenixMotorControlDevRef"=w775, "error in"=w776) -> ("PhoenixMotorControlDevRef"=w771:T2, "error out"=w770:errorcluster)  [unwired: 8 in, 4 out]
                        n225 = call-poly <vilib>:"CTRE_Phoenix_MotorController_Get_Enhanced.vi"("PhoenixMotorControlDevRef"=w766, "error in"=w767) -> ("PhoenixMotorControlDevRef"=w762:T2, "error out"=w761:errorcluster)  [unwired: 8 in, 4 out]
                      }
                    }
                    frame #1 {
                      n226 = while {
                        tunnel: w786 -> [w803]
                        tunnel: w785 -> [w802]
                        tunnel: [w801] -> w784
                        tunnel: [w800] -> w783
                        tunnel: [w796] -> w782
                        tunnel: [w795] -> w781
                        tunnel: w780 -> [w794]
                        tunnel: w779 -> [w793]
                        stop <- w792 stop-if-true
                        w797 = T12 7 items=["PercentOutput"=0, "Position"=1, "Velocity"=2, "Current"=3, "Follower"=5, "MotionProfile"=6, "MotionMagic"=7, "MotionMagicArc"=8, "MotionProfileArc"=10, "Disabled"=15] ("Control Mode")
                        w804 = T12 7 items=["PercentOutput"=0, "Position"=1, "Velocity"=2, "Current"=3, "Follower"=5, "MotionProfile"=6, "MotionMagic"=7, "MotionMagicArc"=8, "MotionProfileArc"=10, "Disabled"=15] ("Control Mode")
                        n227 = global read "Robot Global Data.vi" "Robot Yaw Offset"() -> (w791:dbl)
                        n228 = Wait (ms)(milliseconds to wait=u32 50) -> ()  [unwired: 1 out]
                        n229 = Greater?(x=w791, y=90) -> (0:w792:bool)
                        n230 = Multiply(x=215.75 ("Output"), y=217.294) -> (x*y=w788:dbl)
                        n231 = call <vilib>:"CTRE_Phoenix_MotorControl_Set.vi"("error in (no error)"=w793, "Output"=w788, "Control Mode"=w797, "PhoenixMotorControlDevRef"=w794) -> ("error out"=w799:errorcluster, "PhoenixMotorControlDevRef"=w798:T2)  [unwired: 6 in]
                        n232 = call <vilib>:"CTRE_Phoenix_MotorControl_Set.vi"("error in (no error)"=w802, "Output"=w788, "Control Mode"=w804, "PhoenixMotorControlDevRef"=w803) -> ("error out"=w806:errorcluster, "PhoenixMotorControlDevRef"=w805:T2)  [unwired: 6 in]
                        n233 = call-poly <vilib>:"CTRE_Phoenix_MotorController_Get_Enhanced.vi"("PhoenixMotorControlDevRef"=w798, "error in"=w799) -> ("PhoenixMotorControlDevRef"=w796:T2, "error out"=w795:errorcluster)  [unwired: 8 in, 4 out]
                        n234 = call-poly <vilib>:"CTRE_Phoenix_MotorController_Get_Enhanced.vi"("PhoenixMotorControlDevRef"=w805, "error in"=w806) -> ("PhoenixMotorControlDevRef"=w801:T2, "error out"=w800:errorcluster)  [unwired: 8 in, 4 out]
                      }
                    }
                    frame #2 {
                      n235 = while {
                        tunnel: w815 -> [w834]
                        tunnel: w814 -> [w833]
                        tunnel: [w830] -> w813
                        tunnel: [w829] -> w812
                        tunnel: [w825] -> w811
                        tunnel: [w824] -> w810
                        tunnel: w809 -> [w823]
                        tunnel: w808 -> [w822]
                        stop <- w831 stop-if-true
                        w826 = T12 7 items=["PercentOutput"=0, "Position"=1, "Velocity"=2, "Current"=3, "Follower"=5, "MotionProfile"=6, "MotionMagic"=7, "MotionMagicArc"=8, "MotionProfileArc"=10, "Disabled"=15] ("Control Mode")
                        w835 = T12 7 items=["PercentOutput"=0, "Position"=1, "Velocity"=2, "Current"=3, "Follower"=5, "MotionProfile"=6, "MotionMagic"=7, "MotionMagicArc"=8, "MotionProfileArc"=10, "Disabled"=15] ("Control Mode")
                        n236 = global read "Robot Global Data.vi" "Robot Travel Offset"() -> (w832:dbl)
                        n237 = Wait (ms)(milliseconds to wait=u32 50) -> ()  [unwired: 1 out]
                        n238 = Multiply(x=383.75, y=217.294) -> (x*y=w818:dbl)
                        n239 = Greater?(x=w832, y=w818) -> (0:w831:bool)
                        n240 = Multiply(x=384.75 ("Output"), y=217.294) -> (x*y=w816:dbl)
                        n241 = call <vilib>:"CTRE_Phoenix_MotorControl_Set.vi"("error in (no error)"=w822, "Output"=w816, "Control Mode"=w826, "PhoenixMotorControlDevRef"=w823) -> ("error out"=w828:errorcluster, "PhoenixMotorControlDevRef"=w827:T2)  [unwired: 6 in]
                        n242 = call <vilib>:"CTRE_Phoenix_MotorControl_Set.vi"("error in (no error)"=w833, "Output"=w816, "Control Mode"=w835, "PhoenixMotorControlDevRef"=w834) -> ("error out"=w837:errorcluster, "PhoenixMotorControlDevRef"=w836:T2)  [unwired: 6 in]
                        n243 = call-poly <vilib>:"CTRE_Phoenix_MotorController_Get_Enhanced.vi"("PhoenixMotorControlDevRef"=w827, "error in"=w828) -> ("PhoenixMotorControlDevRef"=w825:T2, "error out"=w824:errorcluster)  [unwired: 8 in, 4 out]
                        n244 = call-poly <vilib>:"CTRE_Phoenix_MotorController_Get_Enhanced.vi"("PhoenixMotorControlDevRef"=w836, "error in"=w837) -> ("PhoenixMotorControlDevRef"=w830:T2, "error out"=w829:errorcluster)  [unwired: 8 in, 4 out]
                      }
                    }
                    frame #3 {
                      n245 = while {
                        tunnel: w846 -> [w863]
                        tunnel: w845 -> [w862]
                        tunnel: [w861] -> w844
                        tunnel: [w860] -> w843
                        tunnel: [w856] -> w842
                        tunnel: [w855] -> w841
                        tunnel: w840 -> [w854]
                        tunnel: w839 -> [w853]
                        stop <- w850 stop-if-true
                        w857 = T12 7 items=["PercentOutput"=0, "Position"=1, "Velocity"=2, "Current"=3, "Follower"=5, "MotionProfile"=6, "MotionMagic"=7, "MotionMagicArc"=8, "MotionProfileArc"=10, "Disabled"=15] ("Control Mode")
                        w864 = T12 7 items=["PercentOutput"=0, "Position"=1, "Velocity"=2, "Current"=3, "Follower"=5, "MotionProfile"=6, "MotionMagic"=7, "MotionMagicArc"=8, "MotionProfileArc"=10, "Disabled"=15] ("Control Mode")
                        n246 = global read "Robot Global Data.vi" "Robot Yaw Offset"() -> (w851:dbl)
                        n247 = Wait (ms)(milliseconds to wait=u32 50) -> ()  [unwired: 1 out]
                        n248 = Less?(x=w851, y=180) -> (x < y?=w850:bool)
                        n249 = Multiply(x=384.75 ("Output"), y=217.294) -> (x*y=w847:dbl)
                        n250 = call <vilib>:"CTRE_Phoenix_MotorControl_Set.vi"("error in (no error)"=w853, "Output"=w847, "Control Mode"=w857, "PhoenixMotorControlDevRef"=w854) -> ("error out"=w859:errorcluster, "PhoenixMotorControlDevRef"=w858:T2)  [unwired: 6 in]
                        n251 = call <vilib>:"CTRE_Phoenix_MotorControl_Set.vi"("error in (no error)"=w862, "Output"=w847, "Control Mode"=w864, "PhoenixMotorControlDevRef"=w863) -> ("error out"=w866:errorcluster, "PhoenixMotorControlDevRef"=w865:T2)  [unwired: 6 in]
                        n252 = call-poly <vilib>:"CTRE_Phoenix_MotorController_Get_Enhanced.vi"("PhoenixMotorControlDevRef"=w858, "error in"=w859) -> ("PhoenixMotorControlDevRef"=w856:T2, "error out"=w855:errorcluster)  [unwired: 8 in, 4 out]
                        n253 = call-poly <vilib>:"CTRE_Phoenix_MotorController_Get_Enhanced.vi"("PhoenixMotorControlDevRef"=w865, "error in"=w866) -> ("PhoenixMotorControlDevRef"=w861:T2, "error out"=w860:errorcluster)  [unwired: 8 in, 4 out]
                      }
                    }
                    frame #4 {
                      n254 = while {
                        tunnel: w875 -> [w894]
                        tunnel: w874 -> [w893]
                        tunnel: [w890] -> w873
                        tunnel: [w889] -> w872
                        tunnel: w871 -> [w885]
                        tunnel: w870 -> [w884]
                        tunnel: [w883] -> w869
                        tunnel: [w882] -> w868
                        stop <- w891 stop-if-true
                        w886 = T12 7 items=["PercentOutput"=0, "Position"=1, "Velocity"=2, "Current"=3, "Follower"=5, "MotionProfile"=6, "MotionMagic"=7, "MotionMagicArc"=8, "MotionProfileArc"=10, "Disabled"=15] ("Control Mode")
                        w895 = T12 7 items=["PercentOutput"=0, "Position"=1, "Velocity"=2, "Current"=3, "Follower"=5, "MotionProfile"=6, "MotionMagic"=7, "MotionMagicArc"=8, "MotionProfileArc"=10, "Disabled"=15] ("Control Mode")
                        n255 = global read "Robot Global Data.vi" "Robot Travel Offset"() -> (w892:dbl)
                        n256 = Wait (ms)(milliseconds to wait=u32 50) -> ()  [unwired: 1 out]
                        n257 = Multiply(x=391.5 ("Output"), y=217.294) -> (x*y=w878:dbl)
                        n258 = call <vilib>:"CTRE_Phoenix_MotorControl_Set.vi"("error in (no error)"=w884, "Output"=w878, "Control Mode"=w886, "PhoenixMotorControlDevRef"=w885) -> ("error out"=w888:errorcluster, "PhoenixMotorControlDevRef"=w887:T2)  [unwired: 6 in]
                        n259 = call <vilib>:"CTRE_Phoenix_MotorControl_Set.vi"("error in (no error)"=w893, "Output"=w878, "Control Mode"=w895, "PhoenixMotorControlDevRef"=w894) -> ("error out"=w897:errorcluster, "PhoenixMotorControlDevRef"=w896:T2)  [unwired: 6 in]
                        n260 = call-poly <vilib>:"CTRE_Phoenix_MotorController_Get_Enhanced.vi"("PhoenixMotorControlDevRef"=w887, "error in"=w888) -> ("PhoenixMotorControlDevRef"=w883:T2, "error out"=w882:errorcluster)  [unwired: 8 in, 4 out]
                        n261 = call-poly <vilib>:"CTRE_Phoenix_MotorController_Get_Enhanced.vi"("PhoenixMotorControlDevRef"=w896, "error in"=w897) -> ("PhoenixMotorControlDevRef"=w890:T2, "error out"=w889:errorcluster)  [unwired: 8 in, 4 out]
                        n262 = Multiply(x=390.5, y=217.294) -> (x*y=w876:dbl)
                        n263 = Greater?(x=w892, y=w876) -> (0:w891:bool)
                      }
                    }
                    frame #5 {
                      n264 = while {
                        tunnel: w906 -> [w924]
                        tunnel: w905 -> [w923]
                        tunnel: [w922] -> w904
                        tunnel: [w921] -> w903
                        tunnel: w902 -> [w917]
                        tunnel: w901 -> [w916]
                        tunnel: [w915] -> w900
                        tunnel: [w914] -> w899
                        i -> [w910]
                        stop <- w911 stop-if-true
                        w918 = T12 7 items=["PercentOutput"=0, "Position"=1, "Velocity"=2, "Current"=3, "Follower"=5, "MotionProfile"=6, "MotionMagic"=7, "MotionMagicArc"=8, "MotionProfileArc"=10, "Disabled"=15] ("Control Mode")
                        w925 = T12 7 items=["PercentOutput"=0, "Position"=1, "Velocity"=2, "Current"=3, "Follower"=5, "MotionProfile"=6, "MotionMagic"=7, "MotionMagicArc"=8, "MotionProfileArc"=10, "Disabled"=15] ("Control Mode")
                        # "ADD INTAKE/ELEVATOR CODE HERE"
                        n265 = Increment(x=w910) -> (x+1=w912:i32)
                        n266 = Wait (ms)(milliseconds to wait=u32 50) -> ()  [unwired: 1 out]
                        n267 = Greater Or Equal?(x=w912, y=20) -> (x >= y?=w911:bool)
                        n268 = Multiply(x=391.5 ("Output"), y=217.294) -> (x*y=w907:dbl)
                        n269 = call <vilib>:"CTRE_Phoenix_MotorControl_Set.vi"("error in (no error)"=w916, "Output"=w907, "Control Mode"=w918, "PhoenixMotorControlDevRef"=w917) -> ("error out"=w920:errorcluster, "PhoenixMotorControlDevRef"=w919:T2)  [unwired: 6 in]
                        n270 = call <vilib>:"CTRE_Phoenix_MotorControl_Set.vi"("error in (no error)"=w923, "Output"=w907, "Control Mode"=w925, "PhoenixMotorControlDevRef"=w924) -> ("error out"=w927:errorcluster, "PhoenixMotorControlDevRef"=w926:T2)  [unwired: 6 in]
                        n271 = call-poly <vilib>:"CTRE_Phoenix_MotorController_Get_Enhanced.vi"("PhoenixMotorControlDevRef"=w919, "error in"=w920) -> ("PhoenixMotorControlDevRef"=w915:T2, "error out"=w914:errorcluster)  [unwired: 8 in, 4 out]
                        n272 = call-poly <vilib>:"CTRE_Phoenix_MotorController_Get_Enhanced.vi"("PhoenixMotorControlDevRef"=w926, "error in"=w927) -> ("PhoenixMotorControlDevRef"=w922:T2, "error out"=w921:errorcluster)  [unwired: 8 in, 4 out]
                      }
                    }
                    frame #6 {
                      n273 = while {
                        tunnel: w932 -> [w943]
                        tunnel: w931 -> [w942]
                        tunnel: w930 -> [w940]
                        tunnel: w929 -> [w939]
                        i -> [w935]
                        stop <- w936 stop-if-true
                        w941 = T12 0 items=["PercentOutput"=0, "Position"=1, "Velocity"=2, "Current"=3, "Follower"=5, "MotionProfile"=6, "MotionMagic"=7, "MotionMagicArc"=8, "MotionProfileArc"=10, "Disabled"=15] ("Control Mode")
                        w944 = T12 0 items=["PercentOutput"=0, "Position"=1, "Velocity"=2, "Current"=3, "Follower"=5, "MotionProfile"=6, "MotionMagic"=7, "MotionMagicArc"=8, "MotionProfileArc"=10, "Disabled"=15] ("Control Mode")
                        n274 = Increment(x=w935) -> (x+1=w937:i32)
                        n275 = Wait (ms)(milliseconds to wait=u32 15000) -> ()  [unwired: 1 out]
                        n276 = call <vilib>:"CTRE_Phoenix_MotorControl_Set.vi"("error in (no error)"=w939, "Output"=0.0, "Control Mode"=w941, "PhoenixMotorControlDevRef"=w940) -> ()  [unwired: 6 in, 2 out]
                        n277 = Greater Or Equal?(x=w937, y=1) -> (x >= y?=w936:bool)
                        n278 = call <vilib>:"CTRE_Phoenix_MotorControl_Set.vi"("error in (no error)"=w942, "Output"=0.0, "Control Mode"=w944, "PhoenixMotorControlDevRef"=w943) -> ()  [unwired: 6 in, 2 out]
                      }
                    }
                  }
                }
              }
            }
            frame 3 {
              n279 = case shown="\"L\"" w950 {
                tunnel: w949 -> [w954 _ w1113]
                tunnel: w948 -> [w953 _ w1112]
                tunnel: w947 -> [w952 _ w1111]
                tunnel: w946 -> [w951 _ w1110]
                frame "R" {
                  n280 = flat-sequence {
                    tunnel: w954 -> [w978]
                    tunnel: w953 -> [w977]
                    tunnel: [w976] -> w970
                    tunnel: [w975] -> w969
                    tunnel: w952 -> [w974]
                    tunnel: w951 -> [w973]
                    tunnel: [w972] -> w968
                    tunnel: [w971] -> w967
                    tunnel: w970 -> [w1010]
                    tunnel: w969 -> [w1009]
                    tunnel: [w1008] -> w966
                    tunnel: [w1007] -> w965
                    tunnel: [w1006] -> w964
                    tunnel: [w1005] -> w963
                    tunnel: w968 -> [w1004]
                    tunnel: w967 -> [w1003]
                    tunnel: w966 -> [w1039]
                    tunnel: w965 -> [w1038]
                    tunnel: w964 -> [w1037]
                    tunnel: w963 -> [w1036]
                    tunnel: [w1035] -> w962
                    tunnel: [w1034] -> w961
                    tunnel: [w1033] -> w960
                    tunnel: [w1032] -> w959
                    tunnel: [w1070] -> w958
                    tunnel: [w1069] -> w957
                    tunnel: [w1068] -> w956
                    tunnel: [w1067] -> w955
                    tunnel: w962 -> [w1066]
                    tunnel: w961 -> [w1065]
                    tunnel: w960 -> [w1064]
                    tunnel: w959 -> [w1063]
                    tunnel: w958 -> [w1096]
                    tunnel: w957 -> [w1095]
                    tunnel: w956 -> [w1094]
                    tunnel: w955 -> [w1093]
                    frame #0 {
                      n281 = while {
                        tunnel: w978 -> [w997]
                        tunnel: w977 -> [w996]
                        tunnel: [w995] -> w976
                        tunnel: [w994] -> w975
                        tunnel: w974 -> [w988]
                        tunnel: w973 -> [w987]
                        tunnel: [w986] -> w972
                        tunnel: [w985] -> w971
                        stop <- w992 stop-if-true
                        w989 = T12 7 items=["PercentOutput"=0, "Position"=1, "Velocity"=2, "Current"=3, "Follower"=5, "MotionProfile"=6, "MotionMagic"=7, "MotionMagicArc"=8, "MotionProfileArc"=10, "Disabled"=15] ("Control Mode")
                        w998 = T12 7 items=["PercentOutput"=0, "Position"=1, "Velocity"=2, "Current"=3, "Follower"=5, "MotionProfile"=6, "MotionMagic"=7, "MotionMagicArc"=8, "MotionProfileArc"=10, "Disabled"=15] ("Control Mode")
                        n282 = global write "Robot Global Data.vi" "Elevator Bottom"(TRUE) -> ()
                        n283 = global read "Robot Global Data.vi" "Robot Travel Offset"() -> (w993:dbl)
                        n284 = Wait (ms)(milliseconds to wait=u32 50) -> ()  [unwired: 1 out]
                        n285 = Multiply(x=88.5 ("Output"), y=217.294) -> (x*y=w981:dbl)
                        n286 = call <vilib>:"CTRE_Phoenix_MotorControl_Set.vi"("error in (no error)"=w996, "Output"=w981, "Control Mode"=w998, "PhoenixMotorControlDevRef"=w997) -> ("error out"=w1000:errorcluster, "PhoenixMotorControlDevRef"=w999:T2)  [unwired: 6 in]
                        n287 = call <vilib>:"CTRE_Phoenix_MotorControl_Set.vi"("error in (no error)"=w987, "Output"=w981, "Control Mode"=w989, "PhoenixMotorControlDevRef"=w988) -> ("error out"=w991:errorcluster, "PhoenixMotorControlDevRef"=w990:T2)  [unwired: 6 in]
                        n288 = call-poly <vilib>:"CTRE_Phoenix_MotorController_Get_Enhanced.vi"("PhoenixMotorControlDevRef"=w999, "error in"=w1000) -> ("PhoenixMotorControlDevRef"=w995:T2, "error out"=w994:errorcluster)  [unwired: 8 in, 4 out]
                        n289 = call-poly <vilib>:"CTRE_Phoenix_MotorController_Get_Enhanced.vi"("PhoenixMotorControlDevRef"=w990, "error in"=w991) -> ("PhoenixMotorControlDevRef"=w986:T2, "error out"=w985:errorcluster)  [unwired: 8 in, 4 out]
                        n290 = Multiply(x=87.5, y=217.294) -> (x*y=w979:dbl)
                        n291 = Greater?(x=w993, y=w979) -> (0:w992:bool)
                      }
                    }
                    frame #1 {
                      n292 = while {
                        tunnel: w1010 -> [w1027]
                        tunnel: w1009 -> [w1026]
                        tunnel: [w1025] -> w1008
                        tunnel: [w1024] -> w1007
                        tunnel: [w1020] -> w1006
                        tunnel: [w1019] -> w1005
                        tunnel: w1004 -> [w1018]
                        tunnel: w1003 -> [w1017]
                        stop <- w1014 stop-if-true
                        w1021 = T12 7 items=["PercentOutput"=0, "Position"=1, "Velocity"=2, "Current"=3, "Follower"=5, "MotionProfile"=6, "MotionMagic"=7, "MotionMagicArc"=8, "MotionProfileArc"=10, "Disabled"=15] ("Control Mode")
                        w1028 = T12 7 items=["PercentOutput"=0, "Position"=1, "Velocity"=2, "Current"=3, "Follower"=5, "MotionProfile"=6, "MotionMagic"=7, "MotionMagicArc"=8, "MotionProfileArc"=10, "Disabled"=15] ("Control Mode")
                        n293 = global read "Robot Global Data.vi" "Robot Yaw Offset"() -> (w1015:dbl)
                        n294 = Wait (ms)(milliseconds to wait=u32 50) -> ()  [unwired: 1 out]
                        n295 = Less?(x=w1015, y=-90) -> (x < y?=w1014:bool)
                        n296 = Multiply(x=88.5 ("Output"), y=217.294) -> (x*y=w1011:dbl)
                        n297 = call <vilib>:"CTRE_Phoenix_MotorControl_Set.vi"("error in (no error)"=w1017, "Output"=w1011, "Control Mode"=w1021, "PhoenixMotorControlDevRef"=w1018) -> ("error out"=w1023:errorcluster, "PhoenixMotorControlDevRef"=w1022:T2)  [unwired: 6 in]
                        n298 = call <vilib>:"CTRE_Phoenix_MotorControl_Set.vi"("error in (no error)"=w1026, "Output"=w1011, "Control Mode"=w1028, "PhoenixMotorControlDevRef"=w1027) -> ("error out"=w1030:errorcluster, "PhoenixMotorControlDevRef"=w1029:T2)  [unwired: 6 in]
                        n299 = call-poly <vilib>:"CTRE_Phoenix_MotorController_Get_Enhanced.vi"("PhoenixMotorControlDevRef"=w1022, "error in"=w1023) -> ("PhoenixMotorControlDevRef"=w1020:T2, "error out"=w1019:errorcluster)  [unwired: 8 in, 4 out]
                        n300 = call-poly <vilib>:"CTRE_Phoenix_MotorController_Get_Enhanced.vi"("PhoenixMotorControlDevRef"=w1029, "error in"=w1030) -> ("PhoenixMotorControlDevRef"=w1025:T2, "error out"=w1024:errorcluster)  [unwired: 8 in, 4 out]
                      }
                    }
                    frame #2 {
                      n301 = while {
                        tunnel: w1039 -> [w1058]
                        tunnel: w1038 -> [w1057]
                        tunnel: [w1054] -> w1035
                        tunnel: [w1053] -> w1033
                        tunnel: [w1049] -> w1034
                        tunnel: [w1048] -> w1032
                        tunnel: w1037 -> [w1047]
                        tunnel: w1036 -> [w1046]
                        stop <- w1055 stop-if-true
                        w1050 = T12 7 items=["PercentOutput"=0, "Position"=1, "Velocity"=2, "Current"=3, "Follower"=5, "MotionProfile"=6, "MotionMagic"=7, "MotionMagicArc"=8, "MotionProfileArc"=10, "Disabled"=15] ("Control Mode")
                        w1059 = T12 7 items=["PercentOutput"=0, "Position"=1, "Velocity"=2, "Current"=3, "Follower"=5, "MotionProfile"=6, "MotionMagic"=7, "MotionMagicArc"=8, "MotionProfileArc"=10, "Disabled"=15] ("Control Mode")
                        n302 = global read "Robot Global Data.vi" "Robot Travel Offset"() -> (w1056:dbl)
                        n303 = Wait (ms)(milliseconds to wait=u32 50) -> ()  [unwired: 1 out]
                        n304 = Multiply(x=107.0 ("Output"), y=217.294) -> (x*y=w1040:dbl)
                        n305 = call <vilib>:"CTRE_Phoenix_MotorControl_Set.vi"("error in (no error)"=w1046, "Output"=w1040, "Control Mode"=w1050, "PhoenixMotorControlDevRef"=w1047) -> ("error out"=w1052:errorcluster, "PhoenixMotorControlDevRef"=w1051:T2)  [unwired: 6 in]
                        n306 = call <vilib>:"CTRE_Phoenix_MotorControl_Set.vi"("error in (no error)"=w1057, "Output"=w1040, "Control Mode"=w1059, "PhoenixMotorControlDevRef"=w1058) -> ("error out"=w1061:errorcluster, "PhoenixMotorControlDevRef"=w1060:T2)  [unwired: 6 in]
                        n307 = call-poly <vilib>:"CTRE_Phoenix_MotorController_Get_Enhanced.vi"("PhoenixMotorControlDevRef"=w1051, "error in"=w1052) -> ("PhoenixMotorControlDevRef"=w1049:T2, "error out"=w1048:errorcluster)  [unwired: 8 in, 4 out]
                        n308 = call-poly <vilib>:"CTRE_Phoenix_MotorController_Get_Enhanced.vi"("PhoenixMotorControlDevRef"=w1060, "error in"=w1061) -> ("PhoenixMotorControlDevRef"=w1054:T2, "error out"=w1053:errorcluster)  [unwired: 8 in, 4 out]
                        n309 = Multiply(x=106, y=217.294) -> (x*y=w1042:dbl)
                        n310 = Greater?(x=w1056, y=w1042) -> (0:w1055:bool)
                      }
                    }
                    frame #3 {
                      n311 = while {
                        tunnel: w1066 -> [w1088]
                        tunnel: w1064 -> [w1087]
                        tunnel: [w1086] -> w1070
                        tunnel: [w1085] -> w1069
                        tunnel: w1065 -> [w1081]
                        tunnel: w1063 -> [w1080]
                        tunnel: [w1079] -> w1068
                        tunnel: [w1078] -> w1067
                        i -> [w1075]
                        stop <- w1074 stop-if-true
                        w1082 = T12 7 items=["PercentOutput"=0, "Position"=1, "Velocity"=2, "Current"=3, "Follower"=5, "MotionProfile"=6, "MotionMagic"=7, "MotionMagicArc"=8, "MotionProfileArc"=10, "Disabled"=15] ("Control Mode")
                        w1089 = T12 7 items=["PercentOutput"=0, "Position"=1, "Velocity"=2, "Current"=3, "Follower"=5, "MotionProfile"=6, "MotionMagic"=7, "MotionMagicArc"=8, "MotionProfileArc"=10, "Disabled"=15] ("Control Mode")
                        # "ADD INTAKE/ELEVATOR CODE HERE"
                        n312 = Increment(x=w1075) -> (x+1=w1076:i32)
                        n313 = Wait (ms)(milliseconds to wait=u32 50) -> ()  [unwired: 1 out]
                        n314 = Greater Or Equal?(x=w1076, y=20) -> (x >= y?=w1074:bool)
                        n315 = Multiply(x=107.0 ("Output"), y=217.294) -> (x*y=w1071:dbl)
                        n316 = call <vilib>:"CTRE_Phoenix_MotorControl_Set.vi"("error in (no error)"=w1080, "Output"=w1071, "Control Mode"=w1082, "PhoenixMotorControlDevRef"=w1081) -> ("error out"=w1084:errorcluster, "PhoenixMotorControlDevRef"=w1083:T2)  [unwired: 6 in]
                        n317 = call <vilib>:"CTRE_Phoenix_MotorControl_Set.vi"("error in (no error)"=w1087, "Output"=w1071, "Control Mode"=w1089, "PhoenixMotorControlDevRef"=w1088) -> ("error out"=w1091:errorcluster, "PhoenixMotorControlDevRef"=w1090:T2)  [unwired: 6 in]
                        n318 = call-poly <vilib>:"CTRE_Phoenix_MotorController_Get_Enhanced.vi"("PhoenixMotorControlDevRef"=w1083, "error in"=w1084) -> ("PhoenixMotorControlDevRef"=w1079:T2, "error out"=w1078:errorcluster)  [unwired: 8 in, 4 out]
                        n319 = call-poly <vilib>:"CTRE_Phoenix_MotorController_Get_Enhanced.vi"("PhoenixMotorControlDevRef"=w1090, "error in"=w1091) -> ("PhoenixMotorControlDevRef"=w1086:T2, "error out"=w1085:errorcluster)  [unwired: 8 in, 4 out]
                      }
                    }
                    frame #4 {
                      n320 = while {
                        tunnel: w1096 -> [w1107]
                        tunnel: w1095 -> [w1106]
                        tunnel: w1094 -> [w1104]
                        tunnel: w1093 -> [w1103]
                        i -> [w1099]
                        stop <- w1100 stop-if-true
                        w1105 = T12 0 items=["PercentOutput"=0, "Position"=1, "Velocity"=2, "Current"=3, "Follower"=5, "MotionProfile"=6, "MotionMagic"=7, "MotionMagicArc"=8, "MotionProfileArc"=10, "Disabled"=15] ("Control Mode")
                        w1108 = T12 0 items=["PercentOutput"=0, "Position"=1, "Velocity"=2, "Current"=3, "Follower"=5, "MotionProfile"=6, "MotionMagic"=7, "MotionMagicArc"=8, "MotionProfileArc"=10, "Disabled"=15] ("Control Mode")
                        n321 = Increment(x=w1099) -> (x+1=w1101:i32)
                        n322 = Wait (ms)(milliseconds to wait=u32 15000) -> ()  [unwired: 1 out]
                        n323 = call <vilib>:"CTRE_Phoenix_MotorControl_Set.vi"("error in (no error)"=w1103, "Output"=0.0, "Control Mode"=w1105, "PhoenixMotorControlDevRef"=w1104) -> ()  [unwired: 6 in, 2 out]
                        n324 = Greater Or Equal?(x=w1101, y=1) -> (x >= y?=w1100:bool)
                        n325 = call <vilib>:"CTRE_Phoenix_MotorControl_Set.vi"("error in (no error)"=w1106, "Output"=0.0, "Control Mode"=w1108, "PhoenixMotorControlDevRef"=w1107) -> ()  [unwired: 6 in, 2 out]
                      }
                    }
                  }
                }
                frame Default {
                }
                frame "L" {
                  n326 = flat-sequence {
                    tunnel: w1113 -> [w1145]
                    tunnel: [w1139] -> _
                    tunnel: [w1144] -> w1137
                    tunnel: [w1143] -> w1136
                    tunnel: w1111 -> [w1142]
                    tunnel: [w1138] -> _
                    tunnel: [w1141] -> w1135
                    tunnel: [w1140] -> w1134
                    tunnel: w1112 -> [w1139]
                    tunnel: w1110 -> [w1138]
                    tunnel: w1137 -> [w1177]
                    tunnel: w1136 -> [w1176]
                    tunnel: [w1175] -> w1133
                    tunnel: [w1174] -> w1132
                    tunnel: [w1173] -> w1131
                    tunnel: [w1172] -> w1130
                    tunnel: w1135 -> [w1171]
                    tunnel: w1134 -> [w1170]
                    tunnel: w1133 -> [w1206]
                    tunnel: w1132 -> [w1205]
                    tunnel: [w1204] -> w1129
                    tunnel: [w1203] -> w1128
                    tunnel: [w1202] -> w1127
                    tunnel: [w1201] -> w1126
                    tunnel: w1131 -> [w1200]
                    tunnel: w1130 -> [w1199]
                    tunnel: w1129 -> [w1237]
                    tunnel: w1128 -> [w1236]
                    tunnel: [w1235] -> w1125
                    tunnel: [w1234] -> w1124
                    tunnel: [w1233] -> w1123
                    tunnel: [w1232] -> w1122
                    tunnel: w1127 -> [w1231]
                    tunnel: w1126 -> [w1230]
                    tunnel: w1125 -> [w1266]
                    tunnel: w1124 -> [w1265]
                    tunnel: [w1264] -> w1121
                    tunnel: [w1263] -> w1120
                    tunnel: w1123 -> [w1262]
                    tunnel: w1122 -> [w1261]
                    tunnel: [w1260] -> w1119
                    tunnel: [w1259] -> w1118
                    tunnel: w1121 -> [w1297]
                    tunnel: w1120 -> [w1296]
                    tunnel: [w1295] -> w1117
                    tunnel: [w1294] -> w1116
                    tunnel: w1119 -> [w1293]
                    tunnel: w1118 -> [w1292]
                    tunnel: [w1291] -> w1115
                    tunnel: [w1290] -> w1114
                    tunnel: w1117 -> [w1323]
                    tunnel: w1116 -> [w1322]
                    tunnel: w1115 -> [w1321]
                    tunnel: w1114 -> [w1320]
                    frame #0 {
                      n327 = while {
                        tunnel: w1145 -> [w1164]
                        tunnel: w1139 -> [w1163]
                        tunnel: [w1162] -> w1144
                        tunnel: [w1161] -> w1143
                        tunnel: w1142 -> [w1155]
                        tunnel: w1138 -> [w1154]
                        tunnel: [w1153] -> w1141
                        tunnel: [w1152] -> w1140
                        stop <- w1159 stop-if-true
                        w1156 = T12 7 items=["PercentOutput"=0, "Position"=1, "Velocity"=2, "Current"=3, "Follower"=5, "MotionProfile"=6, "MotionMagic"=7, "MotionMagicArc"=8, "MotionProfileArc"=10, "Disabled"=15] ("Control Mode")
                        w1165 = T12 7 items=["PercentOutput"=0, "Position"=1, "Velocity"=2, "Current"=3, "Follower"=5, "MotionProfile"=6, "MotionMagic"=7, "MotionMagicArc"=8, "MotionProfileArc"=10, "Disabled"=15] ("Control Mode")
                        n328 = global write "Robot Global Data.vi" "Elevator Bottom"(TRUE) -> ()
                        n329 = global read "Robot Global Data.vi" "Robot Travel Offset"() -> (w1160:dbl)
                        n330 = Wait (ms)(milliseconds to wait=u32 50) -> ()  [unwired: 1 out]
                        n331 = Multiply(x=214.75, y=217.294) -> (x*y=w1146:dbl)
                        n332 = Greater?(x=w1160, y=w1146) -> (0:w1159:bool)
                        n333 = Multiply(x=215.75 ("Output"), y=217.294) -> (x*y=w1148:dbl)
                        n334 = call <vilib>:"CTRE_Phoenix_MotorControl_Set.vi"("error in (no error)"=w1163, "Output"=w1148, "Control Mode"=w1165, "PhoenixMotorControlDevRef"=w1164) -> ("error out"=w1167:errorcluster, "PhoenixMotorControlDevRef"=w1166:T2)  [unwired: 6 in]
                        n335 = call <vilib>:"CTRE_Phoenix_MotorControl_Set.vi"("error in (no error)"=w1154, "Output"=w1148, "Control Mode"=w1156, "PhoenixMotorControlDevRef"=w1155) -> ("error out"=w1158:errorcluster, "PhoenixMotorControlDevRef"=w1157:T2)  [unwired: 6 in]
                        n336 = call-poly <vilib>:"CTRE_Phoenix_MotorController_Get_Enhanced.vi"("PhoenixMotorControlDevRef"=w1166, "error in"=w1167) -> ("PhoenixMotorControlDevRef"=w1162:T2, "error out"=w1161:errorcluster)  [unwired: 8 in, 4 out]
                        n337 = call-poly <vilib>:"CTRE_Phoenix_MotorController_Get_Enhanced.vi"("PhoenixMotorControlDevRef"=w1157, "error in"=w1158) -> ("PhoenixMotorControlDevRef"=w1153:T2, "error out"=w1152:errorcluster)  [unwired: 8 in, 4 out]
                      }
                    }
                    frame #1 {
                      n338 = while {
                        tunnel: w1177 -> [w1194]
                        tunnel: w1176 -> [w1193]
                        tunnel: [w1192] -> w1175
                        tunnel: [w1191] -> w1174
                        tunnel: [w1187] -> w1173
                        tunnel: [w1186] -> w1172
                        tunnel: w1171 -> [w1185]
                        tunnel: w1170 -> [w1184]
                        stop <- w1182 stop-if-true
                        w1188 = T12 7 items=["PercentOutput"=0, "Position"=1, "Velocity"=2, "Current"=3, "Follower"=5, "MotionProfile"=6, "MotionMagic"=7, "MotionMagicArc"=8, "MotionProfileArc"=10, "Disabled"=15] ("Control Mode")
                        w1195 = T12 7 items=["PercentOutput"=0, "Position"=1, "Velocity"=2, "Current"=3, "Follower"=5, "MotionProfile"=6, "MotionMagic"=7, "MotionMagicArc"=8, "MotionProfileArc"=10, "Disabled"=15] ("Control Mode")
                        n339 = global read "Robot Global Data.vi" "Robot Yaw Offset"() -> (w1183:dbl)
                        n340 = Wait (ms)(milliseconds to wait=u32 50) -> ()  [unwired: 1 out]
                        n341 = Less?(x=w1183, y=-90) -> (x < y?=w1182:bool)
                        n342 = Multiply(x=215.75 ("Output"), y=217.294) -> (x*y=w1178:dbl)
                        n343 = call <vilib>:"CTRE_Phoenix_MotorControl_Set.vi"("error in (no error)"=w1184, "Output"=w1178, "Control Mode"=w1188, "PhoenixMotorControlDevRef"=w1185) -> ("error out"=w1190:errorcluster, "PhoenixMotorControlDevRef"=w1189:T2)  [unwired: 6 in]
                        n344 = call <vilib>:"CTRE_Phoenix_MotorControl_Set.vi"("error in (no error)"=w1193, "Output"=w1178, "Control Mode"=w1195, "PhoenixMotorControlDevRef"=w1194) -> ("error out"=w1197:errorcluster, "PhoenixMotorControlDevRef"=w1196:T2)  [unwired: 6 in]
                        n345 = call-poly <vilib>:"CTRE_Phoenix_MotorController_Get_Enhanced.vi"("PhoenixMotorControlDevRef"=w1189, "error in"=w1190) -> ("PhoenixMotorControlDevRef"=w1187:T2, "error out"=w1186:errorcluster)  [unwired: 8 in, 4 out]
                        n346 = call-poly <vilib>:"CTRE_Phoenix_MotorController_Get_Enhanced.vi"("PhoenixMotorControlDevRef"=w1196, "error in"=w1197) -> ("PhoenixMotorControlDevRef"=w1192:T2, "error out"=w1191:errorcluster)  [unwired: 8 in, 4 out]
                      }
                    }
                    frame #2 {
                      n347 = while {
                        tunnel: w1206 -> [w1225]
                        tunnel: w1205 -> [w1224]
                        tunnel: [w1221] -> w1204
                        tunnel: [w1220] -> w1203
                        tunnel: [w1216] -> w1202
                        tunnel: [w1215] -> w1201
                        tunnel: w1200 -> [w1214]
                        tunnel: w1199 -> [w1213]
                        stop <- w1222 stop-if-true
                        w1217 = T12 7 items=["PercentOutput"=0, "Position"=1, "Velocity"=2, "Current"=3, "Follower"=5, "MotionProfile"=6, "MotionMagic"=7, "MotionMagicArc"=8, "MotionProfileArc"=10, "Disabled"=15] ("Control Mode")
                        w1226 = T12 7 items=["PercentOutput"=0, "Position"=1, "Velocity"=2, "Current"=3, "Follower"=5, "MotionProfile"=6, "MotionMagic"=7, "MotionMagicArc"=8, "MotionProfileArc"=10, "Disabled"=15] ("Control Mode")
                        n348 = global read "Robot Global Data.vi" "Robot Travel Offset"() -> (w1223:dbl)
                        n349 = Wait (ms)(milliseconds to wait=u32 50) -> ()  [unwired: 1 out]
                        n350 = Multiply(x=384.75 ("Output"), y=217.294) -> (x*y=w1209:dbl)
                        n351 = call <vilib>:"CTRE_Phoenix_MotorControl_Set.vi"("error in (no error)"=w1213, "Output"=w1209, "Control Mode"=w1217, "PhoenixMotorControlDevRef"=w1214) -> ("error out"=w1219:errorcluster, "PhoenixMotorControlDevRef"=w1218:T2)  [unwired: 6 in]
                        n352 = call <vilib>:"CTRE_Phoenix_MotorControl_Set.vi"("error in (no error)"=w1224, "Output"=w1209, "Control Mode"=w1226, "PhoenixMotorControlDevRef"=w1225) -> ("error out"=w1228:errorcluster, "PhoenixMotorControlDevRef"=w1227:T2)  [unwired: 6 in]
                        n353 = call-poly <vilib>:"CTRE_Phoenix_MotorController_Get_Enhanced.vi"("PhoenixMotorControlDevRef"=w1218, "error in"=w1219) -> ("PhoenixMotorControlDevRef"=w1216:T2, "error out"=w1215:errorcluster)  [unwired: 8 in, 4 out]
                        n354 = call-poly <vilib>:"CTRE_Phoenix_MotorController_Get_Enhanced.vi"("PhoenixMotorControlDevRef"=w1227, "error in"=w1228) -> ("PhoenixMotorControlDevRef"=w1221:T2, "error out"=w1220:errorcluster)  [unwired: 8 in, 4 out]
                        n355 = Multiply(x=383.75, y=217.294) -> (x*y=w1207:dbl)
                        n356 = Greater?(x=w1223, y=w1207) -> (0:w1222:bool)
                      }
                    }
                    frame #3 {
                      n357 = while {
                        tunnel: w1237 -> [w1254]
                        tunnel: w1236 -> [w1253]
                        tunnel: [w1252] -> w1235
                        tunnel: [w1251] -> w1234
                        tunnel: [w1247] -> w1233
                        tunnel: [w1246] -> w1232
                        tunnel: w1231 -> [w1245]
                        tunnel: w1230 -> [w1244]
                        stop <- w1241 stop-if-true
                        w1248 = T12 7 items=["PercentOutput"=0, "Position"=1, "Velocity"=2, "Current"=3, "Follower"=5, "MotionProfile"=6, "MotionMagic"=7, "MotionMagicArc"=8, "MotionProfileArc"=10, "Disabled"=15] ("Control Mode")
                        w1255 = T12 7 items=["PercentOutput"=0, "Position"=1, "Velocity"=2, "Current"=3, "Follower"=5, "MotionProfile"=6, "MotionMagic"=7, "MotionMagicArc"=8, "MotionProfileArc"=10, "Disabled"=15] ("Control Mode")
                        n358 = global read "Robot Global Data.vi" "Robot Yaw Offset"() -> (w1242:dbl)
                        n359 = Wait (ms)(milliseconds to wait=u32 50) -> ()  [unwired: 1 out]
                        n360 = Less?(x=w1242, y=-180) -> (x < y?=w1241:bool)
                        n361 = Multiply(x=384.75 ("Output"), y=217.294) -> (x*y=w1238:dbl)
                        n362 = call <vilib>:"CTRE_Phoenix_MotorControl_Set.vi"("error in (no error)"=w1244, "Output"=w1238, "Control Mode"=w1248, "PhoenixMotorControlDevRef"=w1245) -> ("error out"=w1250:errorcluster, "PhoenixMotorControlDevRef"=w1249:T2)  [unwired: 6 in]
                        n363 = call <vilib>:"CTRE_Phoenix_MotorControl_Set.vi"("error in (no error)"=w1253, "Output"=w1238, "Control Mode"=w1255, "PhoenixMotorControlDevRef"=w1254) -> ("error out"=w1257:errorcluster, "PhoenixMotorControlDevRef"=w1256:T2)  [unwired: 6 in]
                        n364 = call-poly <vilib>:"CTRE_Phoenix_MotorController_Get_Enhanced.vi"("PhoenixMotorControlDevRef"=w1249, "error in"=w1250) -> ("PhoenixMotorControlDevRef"=w1247:T2, "error out"=w1246:errorcluster)  [unwired: 8 in, 4 out]
                        n365 = call-poly <vilib>:"CTRE_Phoenix_MotorController_Get_Enhanced.vi"("PhoenixMotorControlDevRef"=w1256, "error in"=w1257) -> ("PhoenixMotorControlDevRef"=w1252:T2, "error out"=w1251:errorcluster)  [unwired: 8 in, 4 out]
                      }
                    }
                    frame #4 {
                      n366 = while {
                        tunnel: w1266 -> [w1285]
                        tunnel: w1265 -> [w1284]
                        tunnel: [w1281] -> w1264
                        tunnel: [w1280] -> w1263
                        tunnel: w1262 -> [w1276]
                        tunnel: w1261 -> [w1275]
                        tunnel: [w1274] -> w1260
                        tunnel: [w1273] -> w1259
                        stop <- w1282 stop-if-true
                        w1277 = T12 7 items=["PercentOutput"=0, "Position"=1, "Velocity"=2, "Current"=3, "Follower"=5, "MotionProfile"=6, "MotionMagic"=7, "MotionMagicArc"=8, "MotionProfileArc"=10, "Disabled"=15] ("Control Mode")
                        w1286 = T12 7 items=["PercentOutput"=0, "Position"=1, "Velocity"=2, "Current"=3, "Follower"=5, "MotionProfile"=6, "MotionMagic"=7, "MotionMagicArc"=8, "MotionProfileArc"=10, "Disabled"=15] ("Control Mode")
                        n367 = global read "Robot Global Data.vi" "Robot Travel Offset"() -> (w1283:dbl)
                        n368 = Wait (ms)(milliseconds to wait=u32 50) -> ()  [unwired: 1 out]
                        n369 = Multiply(x=390.5, y=217.294) -> (x*y=w1268:dbl)
                        n370 = Greater?(x=w1283, y=w1268) -> (0:w1282:bool)
                        n371 = Multiply(x=391.5 ("Output"), y=217.294) -> (x*y=w1267:dbl)
                        n372 = call <vilib>:"CTRE_Phoenix_MotorControl_Set.vi"("error in (no error)"=w1275, "Output"=w1267, "Control Mode"=w1277, "PhoenixMotorControlDevRef"=w1276) -> ("error out"=w1279:errorcluster, "PhoenixMotorControlDevRef"=w1278:T2)  [unwired: 6 in]
                        n373 = call <vilib>:"CTRE_Phoenix_MotorControl_Set.vi"("error in (no error)"=w1284, "Output"=w1267, "Control Mode"=w1286, "PhoenixMotorControlDevRef"=w1285) -> ("error out"=w1288:errorcluster, "PhoenixMotorControlDevRef"=w1287:T2)  [unwired: 6 in]
                        n374 = call-poly <vilib>:"CTRE_Phoenix_MotorController_Get_Enhanced.vi"("PhoenixMotorControlDevRef"=w1278, "error in"=w1279) -> ("PhoenixMotorControlDevRef"=w1274:T2, "error out"=w1273:errorcluster)  [unwired: 8 in, 4 out]
                        n375 = call-poly <vilib>:"CTRE_Phoenix_MotorController_Get_Enhanced.vi"("PhoenixMotorControlDevRef"=w1287, "error in"=w1288) -> ("PhoenixMotorControlDevRef"=w1281:T2, "error out"=w1280:errorcluster)  [unwired: 8 in, 4 out]
                      }
                    }
                    frame #5 {
                      n376 = while {
                        tunnel: w1297 -> [w1315]
                        tunnel: w1296 -> [w1314]
                        tunnel: [w1313] -> w1295
                        tunnel: [w1312] -> w1294
                        tunnel: w1293 -> [w1308]
                        tunnel: w1292 -> [w1307]
                        tunnel: [w1306] -> w1291
                        tunnel: [w1305] -> w1290
                        i -> [w1302]
                        stop <- w1301 stop-if-true
                        w1309 = T12 7 items=["PercentOutput"=0, "Position"=1, "Velocity"=2, "Current"=3, "Follower"=5, "MotionProfile"=6, "MotionMagic"=7, "MotionMagicArc"=8, "MotionProfileArc"=10, "Disabled"=15] ("Control Mode")
                        w1316 = T12 7 items=["PercentOutput"=0, "Position"=1, "Velocity"=2, "Current"=3, "Follower"=5, "MotionProfile"=6, "MotionMagic"=7, "MotionMagicArc"=8, "MotionProfileArc"=10, "Disabled"=15] ("Control Mode")
                        # "ADD INTAKE/ELEVATOR CODE HERE"
                        n377 = Increment(x=w1302) -> (x+1=w1303:i32)
                        n378 = Wait (ms)(milliseconds to wait=u32 50) -> ()  [unwired: 1 out]
                        n379 = Greater Or Equal?(x=w1303, y=20) -> (x >= y?=w1301:bool)
                        n380 = Multiply(x=391.5 ("Output"), y=217.294) -> (x*y=w1298:dbl)
                        n381 = call <vilib>:"CTRE_Phoenix_MotorControl_Set.vi"("error in (no error)"=w1307, "Output"=w1298, "Control Mode"=w1309, "PhoenixMotorControlDevRef"=w1308) -> ("error out"=w1311:errorcluster, "PhoenixMotorControlDevRef"=w1310:T2)  [unwired: 6 in]
                        n382 = call <vilib>:"CTRE_Phoenix_MotorControl_Set.vi"("error in (no error)"=w1314, "Output"=w1298, "Control Mode"=w1316, "PhoenixMotorControlDevRef"=w1315) -> ("error out"=w1318:errorcluster, "PhoenixMotorControlDevRef"=w1317:T2)  [unwired: 6 in]
                        n383 = call-poly <vilib>:"CTRE_Phoenix_MotorController_Get_Enhanced.vi"("PhoenixMotorControlDevRef"=w1310, "error in"=w1311) -> ("PhoenixMotorControlDevRef"=w1306:T2, "error out"=w1305:errorcluster)  [unwired: 8 in, 4 out]
                        n384 = call-poly <vilib>:"CTRE_Phoenix_MotorController_Get_Enhanced.vi"("PhoenixMotorControlDevRef"=w1317, "error in"=w1318) -> ("PhoenixMotorControlDevRef"=w1313:T2, "error out"=w1312:errorcluster)  [unwired: 8 in, 4 out]
                      }
                    }
                    frame #6 {
                      n385 = while {
                        tunnel: w1323 -> [w1334]
                        tunnel: w1322 -> [w1333]
                        tunnel: w1321 -> [w1331]
                        tunnel: w1320 -> [w1330]
                        i -> [w1326]
                        stop <- w1327 stop-if-true
                        w1332 = T12 0 items=["PercentOutput"=0, "Position"=1, "Velocity"=2, "Current"=3, "Follower"=5, "MotionProfile"=6, "MotionMagic"=7, "MotionMagicArc"=8, "MotionProfileArc"=10, "Disabled"=15] ("Control Mode")
                        w1335 = T12 0 items=["PercentOutput"=0, "Position"=1, "Velocity"=2, "Current"=3, "Follower"=5, "MotionProfile"=6, "MotionMagic"=7, "MotionMagicArc"=8, "MotionProfileArc"=10, "Disabled"=15] ("Control Mode")
                        n386 = Increment(x=w1326) -> (x+1=w1328:i32)
                        n387 = Wait (ms)(milliseconds to wait=u32 15000) -> ()  [unwired: 1 out]
                        n388 = Greater Or Equal?(x=w1328, y=1) -> (x >= y?=w1327:bool)
                        n389 = call <vilib>:"CTRE_Phoenix_MotorControl_Set.vi"("error in (no error)"=w1330, "Output"=0.0, "Control Mode"=w1332, "PhoenixMotorControlDevRef"=w1331) -> ()  [unwired: 6 in, 2 out]
                        n390 = call <vilib>:"CTRE_Phoenix_MotorControl_Set.vi"("error in (no error)"=w1333, "Output"=0.0, "Control Mode"=w1335, "PhoenixMotorControlDevRef"=w1334) -> ()  [unwired: 6 in, 2 out]
                      }
                    }
                  }
                }
              }
            }
            frame 4 {
              n391 = case shown="\"L\"" w1341 {
                tunnel: w1340 -> [w1353 _ w1605]
                tunnel: w1339 -> [w1352 _ w1604]
                tunnel: w1338 -> [w1351 _ w1603]
                tunnel: w1337 -> [w1350 _ w1602]
                frame "R" {
                  n392 = flat-sequence {
                    tunnel: w1353 -> [w1381]
                    tunnel: w1352 -> [w1380]
                    tunnel: [w1379] -> w1373
                    tunnel: [w1378] -> w1372
                    tunnel: w1351 -> [w1377]
                    tunnel: w1350 -> [w1376]
                    tunnel: [w1375] -> w1371
                    tunnel: [w1374] -> w1370
                    tunnel: w1373 -> [w1413]
                    tunnel: w1372 -> [w1412]
                    tunnel: [w1411] -> w1369
                    tunnel: [w1410] -> w1368
                    tunnel: [w1409] -> w1367
                    tunnel: [w1408] -> w1366
                    tunnel: w1371 -> [w1407]
                    tunnel: w1370 -> [w1406]
                    tunnel: w1369 -> [w1442]
                    tunnel: w1368 -> [w1441]
                    tunnel: [w1440] -> w1365
                    tunnel: [w1439] -> w1364
                    tunnel: [w1438] -> w1363
                    tunnel: [w1437] -> w1362
                    tunnel: w1367 -> [w1436]
                    tunnel: w1366 -> [w1435]
                    tunnel: w1365 -> [w1473]
                    tunnel: w1364 -> [w1472]
                    tunnel: [w1471] -> w1361
                    tunnel: [w1470] -> w1360
                    tunnel: [w1469] -> w1359
                    tunnel: [w1468] -> w1358
                    tunnel: w1363 -> [w1467]
                    tunnel: w1362 -> [w1466]
                    tunnel: w1361 -> [w1502]
                    tunnel: w1360 -> [w1501]
                    tunnel: [w1500] -> w1349
                    tunnel: [w1499] -> w1348
                    tunnel: w1359 -> [w1498]
                    tunnel: w1358 -> [w1497]
                    tunnel: [w1496] -> w1347
                    tunnel: [w1495] -> w1346
                    tunnel: w1349 -> [w1533]
                    tunnel: w1348 -> [w1532]
                    tunnel: w1347 -> [w1531]
                    tunnel: w1346 -> [w1530]
                    tunnel: [w1529] -> w1345
                    tunnel: [w1528] -> w1344
                    tunnel: [w1527] -> w1343
                    tunnel: [w1526] -> w1342
                    tunnel: [w1562] -> w1357
                    tunnel: [w1561] -> w1356
                    tunnel: [w1560] -> w1355
                    tunnel: [w1559] -> w1354
                    tunnel: w1345 -> [w1558]
                    tunnel: w1344 -> [w1557]
                    tunnel: w1343 -> [w1556]
                    tunnel: w1342 -> [w1555]
                    tunnel: w1357 -> [w1588]
                    tunnel: w1356 -> [w1587]
                    tunnel: w1355 -> [w1586]
                    tunnel: w1354 -> [w1585]
                    frame #0 {
                      n393 = while {
                        tunnel: w1381 -> [w1400]
                        tunnel: w1380 -> [w1399]
                        tunnel: [w1398] -> w1379
                        tunnel: [w1397] -> w1378
                        tunnel: w1377 -> [w1391]
                        tunnel: w1376 -> [w1390]
                        tunnel: [w1389] -> w1375
                        tunnel: [w1388] -> w1374
                        stop <- w1395 stop-if-true
                        w1392 = T12 7 items=["PercentOutput"=0, "Position"=1, "Velocity"=2, "Current"=3, "Follower"=5, "MotionProfile"=6, "MotionMagic"=7, "MotionMagicArc"=8, "MotionProfileArc"=10, "Disabled"=15] ("Control Mode")
                        w1401 = T12 7 items=["PercentOutput"=0, "Position"=1, "Velocity"=2, "Current"=3, "Follower"=5, "MotionProfile"=6, "MotionMagic"=7, "MotionMagicArc"=8, "MotionProfileArc"=10, "Disabled"=15] ("Control Mode")
                        n394 = global write "Robot Global Data.vi" "Elevator Bottom"(TRUE) -> ()
                        n395 = global read "Robot Global Data.vi" "Robot Travel Offset"() -> (w1396:dbl)
                        n396 = Wait (ms)(milliseconds to wait=u32 50) -> ()  [unwired: 1 out]
                        n397 = Multiply(x=215.75 ("Output"), y=217.294) -> (x*y=w1384:dbl)
                        n398 = call <vilib>:"CTRE_Phoenix_MotorControl_Set.vi"("error in (no error)"=w1399, "Output"=w1384, "Control Mode"=w1401, "PhoenixMotorControlDevRef"=w1400) -> ("error out"=w1403:errorcluster, "PhoenixMotorControlDevRef"=w1402:T2)  [unwired: 6 in]
                        n399 = call <vilib>:"CTRE_Phoenix_MotorControl_Set.vi"("error in (no error)"=w1390, "Output"=w1384, "Control Mode"=w1392, "PhoenixMotorControlDevRef"=w1391) -> ("error out"=w1394:errorcluster, "PhoenixMotorControlDevRef"=w1393:T2)  [unwired: 6 in]
                        n400 = call-poly <vilib>:"CTRE_Phoenix_MotorController_Get_Enhanced.vi"("PhoenixMotorControlDevRef"=w1402, "error in"=w1403) -> ("PhoenixMotorControlDevRef"=w1398:T2, "error out"=w1397:errorcluster)  [unwired: 8 in, 4 out]
                        n401 = call-poly <vilib>:"CTRE_Phoenix_MotorController_Get_Enhanced.vi"("PhoenixMotorControlDevRef"=w1393, "error in"=w1394) -> ("PhoenixMotorControlDevRef"=w1389:T2, "error out"=w1388:errorcluster)  [unwired: 8 in, 4 out]
                        n402 = Multiply(x=214.75, y=217.294) -> (x*y=w1382:dbl)
                        n403 = Greater?(x=w1396, y=w1382) -> (0:w1395:bool)
                      }
                    }
                    frame #1 {
                      n404 = while {
                        tunnel: w1413 -> [w1430]
                        tunnel: w1412 -> [w1429]
                        tunnel: [w1428] -> w1411
                        tunnel: [w1427] -> w1410
                        tunnel: [w1423] -> w1409
                        tunnel: [w1422] -> w1408
                        tunnel: w1407 -> [w1421]
                        tunnel: w1406 -> [w1420]
                        stop <- w1419 stop-if-true
                        w1424 = T12 7 items=["PercentOutput"=0, "Position"=1, "Velocity"=2, "Current"=3, "Follower"=5, "MotionProfile"=6, "MotionMagic"=7, "MotionMagicArc"=8, "MotionProfileArc"=10, "Disabled"=15] ("Control Mode")
                        w1431 = T12 7 items=["PercentOutput"=0, "Position"=1, "Velocity"=2, "Current"=3, "Follower"=5, "MotionProfile"=6, "MotionMagic"=7, "MotionMagicArc"=8, "MotionProfileArc"=10, "Disabled"=15] ("Control Mode")
                        n405 = global read "Robot Global Data.vi" "Robot Yaw Offset"() -> (w1417:dbl)
                        n406 = Wait (ms)(milliseconds to wait=u32 50) -> ()  [unwired: 1 out]
                        n407 = Greater?(x=w1417, y=90) -> (0:w1419:bool)
                        n408 = Multiply(x=215.75 ("Output"), y=217.294) -> (x*y=w1414:dbl)
                        n409 = call <vilib>:"CTRE_Phoenix_MotorControl_Set.vi"("error in (no error)"=w1420, "Output"=w1414, "Control Mode"=w1424, "PhoenixMotorControlDevRef"=w1421) -> ("error out"=w1426:errorcluster, "PhoenixMotorControlDevRef"=w1425:T2)  [unwired: 6 in]
                        n410 = call <vilib>:"CTRE_Phoenix_MotorControl_Set.vi"("error in (no error)"=w1429, "Output"=w1414, "Control Mode"=w1431, "PhoenixMotorControlDevRef"=w1430) -> ("error out"=w1433:errorcluster, "PhoenixMotorControlDevRef"=w1432:T2)  [unwired: 6 in]
                        n411 = call-poly <vilib>:"CTRE_Phoenix_MotorController_Get_Enhanced.vi"("PhoenixMotorControlDevRef"=w1425, "error in"=w1426) -> ("PhoenixMotorControlDevRef"=w1423:T2, "error out"=w1422:errorcluster)  [unwired: 8 in, 4 out]
                        n412 = call-poly <vilib>:"CTRE_Phoenix_MotorController_Get_Enhanced.vi"("PhoenixMotorControlDevRef"=w1432, "error in"=w1433) -> ("PhoenixMotorControlDevRef"=w1428:T2, "error out"=w1427:errorcluster)  [unwired: 8 in, 4 out]
                      }
                    }
                    frame #2 {
                      n413 = while {
                        tunnel: w1442 -> [w1461]
                        tunnel: w1441 -> [w1460]
                        tunnel: [w1457] -> w1440
                        tunnel: [w1456] -> w1439
                        tunnel: [w1452] -> w1438
                        tunnel: [w1451] -> w1437
                        tunnel: w1436 -> [w1450]
                        tunnel: w1435 -> [w1449]
                        stop <- w1458 stop-if-true
                        w1453 = T12 7 items=["PercentOutput"=0, "Position"=1, "Velocity"=2, "Current"=3, "Follower"=5, "MotionProfile"=6, "MotionMagic"=7, "MotionMagicArc"=8, "MotionProfileArc"=10, "Disabled"=15] ("Control Mode")
                        w1462 = T12 7 items=["PercentOutput"=0, "Position"=1, "Velocity"=2, "Current"=3, "Follower"=5, "MotionProfile"=6, "MotionMagic"=7, "MotionMagicArc"=8, "MotionProfileArc"=10, "Disabled"=15] ("Control Mode")
                        n414 = global read "Robot Global Data.vi" "Robot Travel Offset"() -> (w1459:dbl)
                        n415 = Wait (ms)(milliseconds to wait=u32 50) -> ()  [unwired: 1 out]
                        n416 = Multiply(x=439.75, y=217.294) -> (x*y=w1445:dbl)
                        n417 = Greater?(x=w1459, y=w1445) -> (0:w1458:bool)
                        n418 = Multiply(x=440.75 ("Output"), y=217.294) -> (x*y=w1443:dbl)
                        n419 = call <vilib>:"CTRE_Phoenix_MotorControl_Set.vi"("error in (no error)"=w1449, "Output"=w1443, "Control Mode"=w1453, "PhoenixMotorControlDevRef"=w1450) -> ("error out"=w1455:errorcluster, "PhoenixMotorControlDevRef"=w1454:T2)  [unwired: 6 in]
                        n420 = call <vilib>:"CTRE_Phoenix_MotorControl_Set.vi"("error in (no error)"=w1460, "Output"=w1443, "Control Mode"=w1462, "PhoenixMotorControlDevRef"=w1461) -> ("error out"=w1464:errorcluster, "PhoenixMotorControlDevRef"=w1463:T2)  [unwired: 6 in]
                        n421 = call-poly <vilib>:"CTRE_Phoenix_MotorController_Get_Enhanced.vi"("PhoenixMotorControlDevRef"=w1454, "error in"=w1455) -> ("PhoenixMotorControlDevRef"=w1452:T2, "error out"=w1451:errorcluster)  [unwired: 8 in, 4 out]
                        n422 = call-poly <vilib>:"CTRE_Phoenix_MotorController_Get_Enhanced.vi"("PhoenixMotorControlDevRef"=w1463, "error in"=w1464) -> ("PhoenixMotorControlDevRef"=w1457:T2, "error out"=w1456:errorcluster)  [unwired: 8 in, 4 out]
                      }
                    }
                    frame #3 {
                      n423 = while {
                        tunnel: w1473 -> [w1490]
                        tunnel: w1472 -> [w1489]
                        tunnel: [w1488] -> w1471
                        tunnel: [w1487] -> w1470
                        tunnel: [w1483] -> w1469
                        tunnel: [w1482] -> w1468
                        tunnel: w1467 -> [w1481]
                        tunnel: w1466 -> [w1480]
                        stop <- w1477 stop-if-true
                        w1484 = T12 7 items=["PercentOutput"=0, "Position"=1, "Velocity"=2, "Current"=3, "Follower"=5, "MotionProfile"=6, "MotionMagic"=7, "MotionMagicArc"=8, "MotionProfileArc"=10, "Disabled"=15] ("Control Mode")
                        w1491 = T12 7 items=["PercentOutput"=0, "Position"=1, "Velocity"=2, "Current"=3, "Follower"=5, "MotionProfile"=6, "MotionMagic"=7, "MotionMagicArc"=8, "MotionProfileArc"=10, "Disabled"=15] ("Control Mode")
                        n424 = global read "Robot Global Data.vi" "Robot Yaw Offset"() -> (w1478:dbl)
                        n425 = Wait (ms)(milliseconds to wait=u32 50) -> ()  [unwired: 1 out]
                        n426 = Less?(x=w1478, y=0) -> (x < y?=w1477:bool)
                        n427 = Multiply(x=440.75 ("Output"), y=217.294) -> (x*y=w1474:dbl)
                        n428 = call <vilib>:"CTRE_Phoenix_MotorControl_Set.vi"("error in (no error)"=w1480, "Output"=w1474, "Control Mode"=w1484, "PhoenixMotorControlDevRef"=w1481) -> ("error out"=w1486:errorcluster, "PhoenixMotorControlDevRef"=w1485:T2)  [unwired: 6 in]
                        n429 = call <vilib>:"CTRE_Phoenix_MotorControl_Set.vi"("error in (no error)"=w1489, "Output"=w1474, "Control Mode"=w1491, "PhoenixMotorControlDevRef"=w1490) -> ("error out"=w1493:errorcluster, "PhoenixMotorControlDevRef"=w1492:T2)  [unwired: 6 in]
                        n430 = call-poly <vilib>:"CTRE_Phoenix_MotorController_Get_Enhanced.vi"("PhoenixMotorControlDevRef"=w1485, "error in"=w1486) -> ("PhoenixMotorControlDevRef"=w1483:T2, "error out"=w1482:errorcluster)  [unwired: 8 in, 4 out]
                        n431 = call-poly <vilib>:"CTRE_Phoenix_MotorController_Get_Enhanced.vi"("PhoenixMotorControlDevRef"=w1492, "error in"=w1493) -> ("PhoenixMotorControlDevRef"=w1488:T2, "error out"=w1487:errorcluster)  [unwired: 8 in, 4 out]
                      }
                    }
                    frame #4 {
                      n432 = while {
                        tunnel: w1502 -> [w1521]
                        tunnel: w1501 -> [w1520]
                        tunnel: [w1517] -> w1500
                        tunnel: [w1516] -> w1499
                        tunnel: w1498 -> [w1512]
                        tunnel: w1497 -> [w1511]
                        tunnel: [w1510] -> w1496
                        tunnel: [w1509] -> w1495
                        stop <- w1518 stop-if-true
                        w1513 = T12 7 items=["PercentOutput"=0, "Position"=1, "Velocity"=2, "Current"=3, "Follower"=5, "MotionProfile"=6, "MotionMagic"=7, "MotionMagicArc"=8, "MotionProfileArc"=10, "Disabled"=15] ("Control Mode")
                        w1522 = T12 7 items=["PercentOutput"=0, "Position"=1, "Velocity"=2, "Current"=3, "Follower"=5, "MotionProfile"=6, "MotionMagic"=7, "MotionMagicArc"=8, "MotionProfileArc"=10, "Disabled"=15] ("Control Mode")
                        n433 = global read "Robot Global Data.vi" "Robot Travel Offset"() -> (w1519:dbl)
                        n434 = Wait (ms)(milliseconds to wait=u32 50) -> ()  [unwired: 1 out]
                        n435 = Multiply(x=529.5 ("Output"), y=217.294) -> (x*y=w1506:dbl)
                        n436 = call <vilib>:"CTRE_Phoenix_MotorControl_Set.vi"("error in (no error)"=w1511, "Output"=w1506, "Control Mode"=w1513, "PhoenixMotorControlDevRef"=w1512) -> ("error out"=w1515:errorcluster, "PhoenixMotorControlDevRef"=w1514:T2)  [unwired: 6 in]
                        n437 = call <vilib>:"CTRE_Phoenix_MotorControl_Set.vi"("error in (no error)"=w1520, "Output"=w1506, "Control Mode"=w1522, "PhoenixMotorControlDevRef"=w1521) -> ("error out"=w1524:errorcluster, "PhoenixMotorControlDevRef"=w1523:T2)  [unwired: 6 in]
                        n438 = call-poly <vilib>:"CTRE_Phoenix_MotorController_Get_Enhanced.vi"("PhoenixMotorControlDevRef"=w1514, "error in"=w1515) -> ("PhoenixMotorControlDevRef"=w1510:T2, "error out"=w1509:errorcluster)  [unwired: 8 in, 4 out]
                        n439 = call-poly <vilib>:"CTRE_Phoenix_MotorController_Get_Enhanced.vi"("PhoenixMotorControlDevRef"=w1523, "error in"=w1524) -> ("PhoenixMotorControlDevRef"=w1517:T2, "error out"=w1516:errorcluster)  [unwired: 8 in, 4 out]
                        n440 = Multiply(x=528.5, y=217.294) -> (x*y=w1503:dbl)
                        n441 = Greater?(x=w1519, y=w1503) -> (0:w1518:bool)
                      }
                    }
                    frame #5 {
                      n442 = while {
                        tunnel: w1533 -> [w1550]
                        tunnel: w1532 -> [w1549]
                        tunnel: [w1548] -> w1529
                        tunnel: [w1547] -> w1528
                        tunnel: [w1543] -> w1527
                        tunnel: [w1542] -> w1526
                        tunnel: w1531 -> [w1541]
                        tunnel: w1530 -> [w1540]
                        stop <- w1537 stop-if-true
                        w1544 = T12 7 items=["PercentOutput"=0, "Position"=1, "Velocity"=2, "Current"=3, "Follower"=5, "MotionProfile"=6, "MotionMagic"=7, "MotionMagicArc"=8, "MotionProfileArc"=10, "Disabled"=15] ("Control Mode")
                        w1551 = T12 7 items=["PercentOutput"=0, "Position"=1, "Velocity"=2, "Current"=3, "Follower"=5, "MotionProfile"=6, "MotionMagic"=7, "MotionMagicArc"=8, "MotionProfileArc"=10, "Disabled"=15] ("Control Mode")
                        n443 = global read "Robot Global Data.vi" "Robot Yaw Offset"() -> (w1538:dbl)
                        n444 = Wait (ms)(milliseconds to wait=u32 50) -> ()  [unwired: 1 out]
                        n445 = Less?(x=w1538, y=-90) -> (x < y?=w1537:bool)
                        n446 = Multiply(x=529.5 ("Output"), y=217.294) -> (x*y=w1534:dbl)
                        n447 = call <vilib>:"CTRE_Phoenix_MotorControl_Set.vi"("error in (no error)"=w1540, "Output"=w1534, "Control Mode"=w1544, "PhoenixMotorControlDevRef"=w1541) -> ("error out"=w1546:errorcluster, "PhoenixMotorControlDevRef"=w1545:T2)  [unwired: 6 in]
                        n448 = call <vilib>:"CTRE_Phoenix_MotorControl_Set.vi"("error in (no error)"=w1549, "Output"=w1534, "Control Mode"=w1551, "PhoenixMotorControlDevRef"=w1550) -> ("error out"=w1553:errorcluster, "PhoenixMotorControlDevRef"=w1552:T2)  [unwired: 6 in]
                        n449 = call-poly <vilib>:"CTRE_Phoenix_MotorController_Get_Enhanced.vi"("PhoenixMotorControlDevRef"=w1545, "error in"=w1546) -> ("PhoenixMotorControlDevRef"=w1543:T2, "error out"=w1542:errorcluster)  [unwired: 8 in, 4 out]
                        n450 = call-poly <vilib>:"CTRE_Phoenix_MotorController_Get_Enhanced.vi"("PhoenixMotorControlDevRef"=w1552, "error in"=w1553) -> ("PhoenixMotorControlDevRef"=w1548:T2, "error out"=w1547:errorcluster)  [unwired: 8 in, 4 out]
                      }
                    }
                    frame #6 {
                      n451 = while {
                        tunnel: [w1580] -> w1562
                        tunnel: [w1579] -> w1561
                        tunnel: [w1575] -> w1560
                        tunnel: [w1574] -> w1559
                        tunnel: w1558 -> [w1573]
                        tunnel: w1557 -> [w1572]
                        tunnel: w1556 -> [w1571]
                        tunnel: w1555 -> [w1570]
                        i -> [w1566]
                        stop <- w1567 stop-if-true
                        w1576 = T12 7 items=["PercentOutput"=0, "Position"=1, "Velocity"=2, "Current"=3, "Follower"=5, "MotionProfile"=6, "MotionMagic"=7, "MotionMagicArc"=8, "MotionProfileArc"=10, "Disabled"=15] ("Control Mode")
                        w1581 = T12 7 items=["PercentOutput"=0, "Position"=1, "Velocity"=2, "Current"=3, "Follower"=5, "MotionProfile"=6, "MotionMagic"=7, "MotionMagicArc"=8, "MotionProfileArc"=10, "Disabled"=15] ("Control Mode")
                        # "ADD INTAKE/ELEVATOR CODE HERE"
                        n452 = Increment(x=w1566) -> (x+1=w1568:i32)
                        n453 = Wait (ms)(milliseconds to wait=u32 50) -> ()  [unwired: 1 out]
                        n454 = Greater Or Equal?(x=w1568, y=20) -> (x >= y?=w1567:bool)
                        n455 = Multiply(x=529.5 ("Output"), y=217.294) -> (x*y=w1563:dbl)
                        n456 = call <vilib>:"CTRE_Phoenix_MotorControl_Set.vi"("error in (no error)"=w1570, "Output"=w1563, "Control Mode"=w1576, "PhoenixMotorControlDevRef"=w1571) -> ("error out"=w1578:errorcluster, "PhoenixMotorControlDevRef"=w1577:T2)  [unwired: 6 in]
                        n457 = call <vilib>:"CTRE_Phoenix_MotorControl_Set.vi"("error in (no error)"=w1572, "Output"=w1563, "Control Mode"=w1581, "PhoenixMotorControlDevRef"=w1573) -> ("error out"=w1583:errorcluster, "PhoenixMotorControlDevRef"=w1582:T2)  [unwired: 6 in]
                        n458 = call-poly <vilib>:"CTRE_Phoenix_MotorController_Get_Enhanced.vi"("PhoenixMotorControlDevRef"=w1577, "error in"=w1578) -> ("PhoenixMotorControlDevRef"=w1575:T2, "error out"=w1574:errorcluster)  [unwired: 8 in, 4 out]
                        n459 = call-poly <vilib>:"CTRE_Phoenix_MotorController_Get_Enhanced.vi"("PhoenixMotorControlDevRef"=w1582, "error in"=w1583) -> ("PhoenixMotorControlDevRef"=w1580:T2, "error out"=w1579:errorcluster)  [unwired: 8 in, 4 out]
                      }
                    }
                    frame #7 {
                      n460 = while {
                        tunnel: w1588 -> [w1599]
                        tunnel: w1587 -> [w1598]
                        tunnel: w1586 -> [w1596]
                        tunnel: w1585 -> [w1595]
                        i -> [w1589]
                        stop <- w1590 stop-if-true
                        w1597 = T12 0 items=["PercentOutput"=0, "Position"=1, "Velocity"=2, "Current"=3, "Follower"=5, "MotionProfile"=6, "MotionMagic"=7, "MotionMagicArc"=8, "MotionProfileArc"=10, "Disabled"=15] ("Control Mode")
                        w1600 = T12 0 items=["PercentOutput"=0, "Position"=1, "Velocity"=2, "Current"=3, "Follower"=5, "MotionProfile"=6, "MotionMagic"=7, "MotionMagicArc"=8, "MotionProfileArc"=10, "Disabled"=15] ("Control Mode")
                        n461 = Increment(x=w1589) -> (x+1=w1591:i32)
                        n462 = Wait (ms)(milliseconds to wait=u32 15000) -> ()  [unwired: 1 out]
                        n463 = Greater Or Equal?(x=w1591, y=1) -> (x >= y?=w1590:bool)
                        n464 = call <vilib>:"CTRE_Phoenix_MotorControl_Set.vi"("error in (no error)"=w1595, "Output"=0.0, "Control Mode"=w1597, "PhoenixMotorControlDevRef"=w1596) -> ()  [unwired: 6 in, 2 out]
                        n465 = call <vilib>:"CTRE_Phoenix_MotorControl_Set.vi"("error in (no error)"=w1598, "Output"=0.0, "Control Mode"=w1600, "PhoenixMotorControlDevRef"=w1599) -> ()  [unwired: 6 in, 2 out]
                      }
                    }
                  }
                }
                frame Default {
                }
                frame "L" {
                  n466 = flat-sequence {
                    tunnel: w1605 -> [w1629]
                    tunnel: w1604 -> [w1628]
                    tunnel: [w1627] -> w1621
                    tunnel: [w1626] -> w1620
                    tunnel: w1603 -> [w1625]
                    tunnel: w1602 -> [w1624]
                    tunnel: [w1623] -> w1619
                    tunnel: [w1622] -> w1618
                    tunnel: w1621 -> [w1661]
                    tunnel: w1620 -> [w1660]
                    tunnel: [w1659] -> w1617
                    tunnel: [w1658] -> w1616
                    tunnel: [w1657] -> w1615
                    tunnel: [w1656] -> w1614
                    tunnel: w1619 -> [w1655]
                    tunnel: w1618 -> [w1654]
                    tunnel: w1617 -> [w1690]
                    tunnel: w1616 -> [w1689]
                    tunnel: w1615 -> [w1688]
                    tunnel: w1614 -> [w1687]
                    tunnel: [w1686] -> w1613
                    tunnel: [w1685] -> w1612
                    tunnel: [w1684] -> w1611
                    tunnel: [w1683] -> w1610
                    tunnel: [w1721] -> w1609
                    tunnel: [w1720] -> w1608
                    tunnel: [w1719] -> w1607
                    tunnel: [w1718] -> w1606
                    tunnel: w1613 -> [w1717]
                    tunnel: w1612 -> [w1716]
                    tunnel: w1611 -> [w1715]
                    tunnel: w1610 -> [w1714]
                    tunnel: w1609 -> [w1747]
                    tunnel: w1608 -> [w1746]
                    tunnel: w1607 -> [w1745]
                    tunnel: w1606 -> [w1744]
                    frame #0 {
                      n467 = while {
                        tunnel: w1629 -> [w1648]
                        tunnel: w1628 -> [w1647]
                        tunnel: [w1646] -> w1627
                        tunnel: [w1645] -> w1626
                        tunnel: w1625 -> [w1639]
                        tunnel: w1624 -> [w1638]
                        tunnel: [w1637] -> w1623
                        tunnel: [w1636] -> w1622
                        stop <- w1643 stop-if-true
                        w1640 = T12 7 items=["PercentOutput"=0, "Position"=1, "Velocity"=2, "Current"=3, "Follower"=5, "MotionProfile"=6, "MotionMagic"=7, "MotionMagicArc"=8, "MotionProfileArc"=10, "Disabled"=15] ("Control Mode")
                        w1649 = T12 7 items=["PercentOutput"=0, "Position"=1, "Velocity"=2, "Current"=3, "Follower"=5, "MotionProfile"=6, "MotionMagic"=7, "MotionMagicArc"=8, "MotionProfileArc"=10, "Disabled"=15] ("Control Mode")
                        n468 = global write "Robot Global Data.vi" "Elevator Bottom"(TRUE) -> ()
                        n469 = global read "Robot Global Data.vi" "Robot Travel Offset"() -> (w1644:dbl)
                        n470 = Wait (ms)(milliseconds to wait=u32 50) -> ()  [unwired: 1 out]
                        n471 = Multiply(x=303.5, y=217.294) -> (x*y=w1630:dbl)
                        n472 = Greater?(x=w1644, y=w1630) -> (0:w1643:bool)
                        n473 = Multiply(x=304.5 ("Output"), y=217.294) -> (x*y=w1633:dbl)
                        n474 = call <vilib>:"CTRE_Phoenix_MotorControl_Set.vi"("error in (no error)"=w1647, "Output"=w1633, "Control Mode"=w1649, "PhoenixMotorControlDevRef"=w1648) -> ("error out"=w1651:errorcluster, "PhoenixMotorControlDevRef"=w1650:T2)  [unwired: 6 in]
                        n475 = call <vilib>:"CTRE_Phoenix_MotorControl_Set.vi"("error in (no error)"=w1638, "Output"=w1633, "Control Mode"=w1640, "PhoenixMotorControlDevRef"=w1639) -> ("error out"=w1642:errorcluster, "PhoenixMotorControlDevRef"=w1641:T2)  [unwired: 6 in]
                        n476 = call-poly <vilib>:"CTRE_Phoenix_MotorController_Get_Enhanced.vi"("PhoenixMotorControlDevRef"=w1650, "error in"=w1651) -> ("PhoenixMotorControlDevRef"=w1646:T2, "error out"=w1645:errorcluster)  [unwired: 8 in, 4 out]
                        n477 = call-poly <vilib>:"CTRE_Phoenix_MotorController_Get_Enhanced.vi"("PhoenixMotorControlDevRef"=w1641, "error in"=w1642) -> ("PhoenixMotorControlDevRef"=w1637:T2, "error out"=w1636:errorcluster)  [unwired: 8 in, 4 out]
                      }
                    }
                    frame #1 {
                      n478 = while {
                        tunnel: w1661 -> [w1678]
                        tunnel: w1660 -> [w1677]
                        tunnel: [w1676] -> w1659
                        tunnel: [w1675] -> w1658
                        tunnel: [w1671] -> w1657
                        tunnel: [w1670] -> w1656
                        tunnel: w1655 -> [w1669]
                        tunnel: w1654 -> [w1668]
                        stop <- w1667 stop-if-true
                        w1672 = T12 7 items=["PercentOutput"=0, "Position"=1, "Velocity"=2, "Current"=3, "Follower"=5, "MotionProfile"=6, "MotionMagic"=7, "MotionMagicArc"=8, "MotionProfileArc"=10, "Disabled"=15] ("Control Mode")
                        w1679 = T12 7 items=["PercentOutput"=0, "Position"=1, "Velocity"=2, "Current"=3, "Follower"=5, "MotionProfile"=6, "MotionMagic"=7, "MotionMagicArc"=8, "MotionProfileArc"=10, "Disabled"=15] ("Control Mode")
                        n479 = global read "Robot Global Data.vi" "Robot Yaw Offset"() -> (w1665:dbl)
                        n480 = Wait (ms)(milliseconds to wait=u32 50) -> ()  [unwired: 1 out]
                        n481 = Greater?(x=w1665, y=90) -> (0:w1667:bool)
                        n482 = Multiply(x=304.5 ("Output"), y=217.294) -> (x*y=w1662:dbl)
                        n483 = call <vilib>:"CTRE_Phoenix_MotorControl_Set.vi"("error in (no error)"=w1668, "Output"=w1662, "Control Mode"=w1672, "PhoenixMotorControlDevRef"=w1669) -> ("error out"=w1674:errorcluster, "PhoenixMotorControlDevRef"=w1673:T2)  [unwired: 6 in]
                        n484 = call <vilib>:"CTRE_Phoenix_MotorControl_Set.vi"("error in (no error)"=w1677, "Output"=w1662, "Control Mode"=w1679, "PhoenixMotorControlDevRef"=w1678) -> ("error out"=w1681:errorcluster, "PhoenixMotorControlDevRef"=w1680:T2)  [unwired: 6 in]
                        n485 = call-poly <vilib>:"CTRE_Phoenix_MotorController_Get_Enhanced.vi"("PhoenixMotorControlDevRef"=w1673, "error in"=w1674) -> ("PhoenixMotorControlDevRef"=w1671:T2, "error out"=w1670:errorcluster)  [unwired: 8 in, 4 out]
                        n486 = call-poly <vilib>:"CTRE_Phoenix_MotorController_Get_Enhanced.vi"("PhoenixMotorControlDevRef"=w1680, "error in"=w1681) -> ("PhoenixMotorControlDevRef"=w1676:T2, "error out"=w1675:errorcluster)  [unwired: 8 in, 4 out]
                      }
                    }
                    frame #2 {
                      n487 = while {
                        tunnel: w1690 -> [w1709]
                        tunnel: w1689 -> [w1708]
                        tunnel: [w1705] -> w1686
                        tunnel: [w1704] -> w1684
                        tunnel: [w1700] -> w1685
                        tunnel: [w1699] -> w1683
                        tunnel: w1688 -> [w1698]
                        tunnel: w1687 -> [w1697]
                        stop <- w1706 stop-if-true
                        w1701 = T12 7 items=["PercentOutput"=0, "Position"=1, "Velocity"=2, "Current"=3, "Follower"=5, "MotionProfile"=6, "MotionMagic"=7, "MotionMagicArc"=8, "MotionProfileArc"=10, "Disabled"=15] ("Control Mode")
                        w1710 = T12 7 items=["PercentOutput"=0, "Position"=1, "Velocity"=2, "Current"=3, "Follower"=5, "MotionProfile"=6, "MotionMagic"=7, "MotionMagicArc"=8, "MotionProfileArc"=10, "Disabled"=15] ("Control Mode")
                        n488 = global read "Robot Global Data.vi" "Robot Travel Offset"() -> (w1707:dbl)
                        n489 = Wait (ms)(milliseconds to wait=u32 50) -> ()  [unwired: 1 out]
                        n490 = Multiply(x=309.5 ("Output"), y=217.294) -> (x*y=w1694:dbl)
                        n491 = call <vilib>:"CTRE_Phoenix_MotorControl_Set.vi"("error in (no error)"=w1697, "Output"=w1694, "Control Mode"=w1701, "PhoenixMotorControlDevRef"=w1698) -> ("error out"=w1703:errorcluster, "PhoenixMotorControlDevRef"=w1702:T2)  [unwired: 6 in]
                        n492 = call <vilib>:"CTRE_Phoenix_MotorControl_Set.vi"("error in (no error)"=w1708, "Output"=w1694, "Control Mode"=w1710, "PhoenixMotorControlDevRef"=w1709) -> ("error out"=w1712:errorcluster, "PhoenixMotorControlDevRef"=w1711:T2)  [unwired: 6 in]
                        n493 = call-poly <vilib>:"CTRE_Phoenix_MotorController_Get_Enhanced.vi"("PhoenixMotorControlDevRef"=w1702, "error in"=w1703) -> ("PhoenixMotorControlDevRef"=w1700:T2, "error out"=w1699:errorcluster)  [unwired: 8 in, 4 out]
                        n494 = call-poly <vilib>:"CTRE_Phoenix_MotorController_Get_Enhanced.vi"("PhoenixMotorControlDevRef"=w1711, "error in"=w1712) -> ("PhoenixMotorControlDevRef"=w1705:T2, "error out"=w1704:errorcluster)  [unwired: 8 in, 4 out]
                        n495 = Multiply(x=308.5, y=217.294) -> (x*y=w1691:dbl)
                        n496 = Greater?(x=w1707, y=w1691) -> (0:w1706:bool)
                      }
                    }
                    frame #3 {
                      n497 = while {
                        tunnel: w1717 -> [w1739]
                        tunnel: w1715 -> [w1738]
                        tunnel: [w1737] -> w1721
                        tunnel: [w1736] -> w1720
                        tunnel: w1716 -> [w1732]
                        tunnel: w1714 -> [w1731]
                        tunnel: [w1730] -> w1719
                        tunnel: [w1729] -> w1718
                        i -> [w1725]
                        stop <- w1726 stop-if-true
                        w1733 = T12 7 items=["PercentOutput"=0, "Position"=1, "Velocity"=2, "Current"=3, "Follower"=5, "MotionProfile"=6, "MotionMagic"=7, "MotionMagicArc"=8, "MotionProfileArc"=10, "Disabled"=15] ("Control Mode")
                        w1740 = T12 7 items=["PercentOutput"=0, "Position"=1, "Velocity"=2, "Current"=3, "Follower"=5, "MotionProfile"=6, "MotionMagic"=7, "MotionMagicArc"=8, "MotionProfileArc"=10, "Disabled"=15] ("Control Mode")
                        # "ADD INTAKE/ELEVATOR CODE HERE"
                        n498 = Increment(x=w1725) -> (x+1=w1727:i32)
                        n499 = Wait (ms)(milliseconds to wait=u32 50) -> ()  [unwired: 1 out]
                        n500 = Greater Or Equal?(x=w1727, y=20) -> (x >= y?=w1726:bool)
                        n501 = Multiply(x=309.5 ("Output"), y=217.294) -> (x*y=w1722:dbl)
                        n502 = call <vilib>:"CTRE_Phoenix_MotorControl_Set.vi"("error in (no error)"=w1731, "Output"=w1722, "Control Mode"=w1733, "PhoenixMotorControlDevRef"=w1732) -> ("error out"=w1735:errorcluster, "PhoenixMotorControlDevRef"=w1734:T2)  [unwired: 6 in]
                        n503 = call <vilib>:"CTRE_Phoenix_MotorControl_Set.vi"("error in (no error)"=w1738, "Output"=w1722, "Control Mode"=w1740, "PhoenixMotorControlDevRef"=w1739) -> ("error out"=w1742:errorcluster, "PhoenixMotorControlDevRef"=w1741:T2)  [unwired: 6 in]
                        n504 = call-poly <vilib>:"CTRE_Phoenix_MotorController_Get_Enhanced.vi"("PhoenixMotorControlDevRef"=w1734, "error in"=w1735) -> ("PhoenixMotorControlDevRef"=w1730:T2, "error out"=w1729:errorcluster)  [unwired: 8 in, 4 out]
                        n505 = call-poly <vilib>:"CTRE_Phoenix_MotorController_Get_Enhanced.vi"("PhoenixMotorControlDevRef"=w1741, "error in"=w1742) -> ("PhoenixMotorControlDevRef"=w1737:T2, "error out"=w1736:errorcluster)  [unwired: 8 in, 4 out]
                      }
                    }
                    frame #4 {
                      n506 = while {
                        tunnel: w1747 -> [w1758]
                        tunnel: w1746 -> [w1757]
                        tunnel: w1745 -> [w1755]
                        tunnel: w1744 -> [w1754]
                        i -> [w1748]
                        stop <- w1749 stop-if-true
                        w1756 = T12 0 items=["PercentOutput"=0, "Position"=1, "Velocity"=2, "Current"=3, "Follower"=5, "MotionProfile"=6, "MotionMagic"=7, "MotionMagicArc"=8, "MotionProfileArc"=10, "Disabled"=15] ("Control Mode")
                        w1759 = T12 0 items=["PercentOutput"=0, "Position"=1, "Velocity"=2, "Current"=3, "Follower"=5, "MotionProfile"=6, "MotionMagic"=7, "MotionMagicArc"=8, "MotionProfileArc"=10, "Disabled"=15] ("Control Mode")
                        n507 = Increment(x=w1748) -> (x+1=w1750:i32)
                        n508 = Greater Or Equal?(x=w1750, y=1) -> (x >= y?=w1749:bool)
                        n509 = Wait (ms)(milliseconds to wait=u32 15000) -> ()  [unwired: 1 out]
                        n510 = call <vilib>:"CTRE_Phoenix_MotorControl_Set.vi"("error in (no error)"=w1754, "Output"=0.0, "Control Mode"=w1756, "PhoenixMotorControlDevRef"=w1755) -> ()  [unwired: 6 in, 2 out]
                        n511 = call <vilib>:"CTRE_Phoenix_MotorControl_Set.vi"("error in (no error)"=w1757, "Output"=0.0, "Control Mode"=w1759, "PhoenixMotorControlDevRef"=w1758) -> ()  [unwired: 6 in, 2 out]
                      }
                    }
                  }
                }
              }
            }
            frame 5 {
              n512 = case shown="\"R\"" w1765 {
                tunnel: w1764 -> [w1769 _ w1928]
                tunnel: w1763 -> [w1768 _ w1927]
                tunnel: w1762 -> [w1767 _ w1926]
                tunnel: w1761 -> [w1766 _ w1925]
                frame "R" {
                  n513 = flat-sequence {
                    tunnel: w1769 -> [w1793]
                    tunnel: w1768 -> [w1792]
                    tunnel: [w1791] -> w1785
                    tunnel: [w1790] -> w1784
                    tunnel: w1767 -> [w1789]
                    tunnel: w1766 -> [w1788]
                    tunnel: [w1787] -> w1783
                    tunnel: [w1786] -> w1782
                    tunnel: w1785 -> [w1825]
                    tunnel: w1784 -> [w1824]
                    tunnel: [w1823] -> w1781
                    tunnel: [w1822] -> w1780
                    tunnel: [w1821] -> w1779
                    tunnel: [w1820] -> w1778
                    tunnel: w1783 -> [w1819]
                    tunnel: w1782 -> [w1818]
                    tunnel: w1781 -> [w1854]
                    tunnel: w1780 -> [w1853]
                    tunnel: w1779 -> [w1852]
                    tunnel: w1778 -> [w1851]
                    tunnel: [w1850] -> w1777
                    tunnel: [w1849] -> w1776
                    tunnel: [w1848] -> w1775
                    tunnel: [w1847] -> w1774
                    tunnel: [w1885] -> w1773
                    tunnel: [w1884] -> w1772
                    tunnel: [w1883] -> w1771
                    tunnel: [w1882] -> w1770
                    tunnel: w1777 -> [w1881]
                    tunnel: w1776 -> [w1880]
                    tunnel: w1775 -> [w1879]
                    tunnel: w1774 -> [w1878]
                    tunnel: w1773 -> [w1911]
                    tunnel: w1772 -> [w1910]
                    tunnel: w1771 -> [w1909]
                    tunnel: w1770 -> [w1908]
                    frame #0 {
                      n514 = while {
                        tunnel: w1793 -> [w1812]
                        tunnel: w1792 -> [w1811]
                        tunnel: [w1810] -> w1791
                        tunnel: [w1809] -> w1790
                        tunnel: w1789 -> [w1803]
                        tunnel: w1788 -> [w1802]
                        tunnel: [w1801] -> w1787
                        tunnel: [w1800] -> w1786
                        stop <- w1807 stop-if-true
                        w1804 = T12 7 items=["PercentOutput"=0, "Position"=1, "Velocity"=2, "Current"=3, "Follower"=5, "MotionProfile"=6, "MotionMagic"=7, "MotionMagicArc"=8, "MotionProfileArc"=10, "Disabled"=15] ("Control Mode")
                        w1813 = T12 7 items=["PercentOutput"=0, "Position"=1, "Velocity"=2, "Current"=3, "Follower"=5, "MotionProfile"=6, "MotionMagic"=7, "MotionMagicArc"=8, "MotionProfileArc"=10, "Disabled"=15] ("Control Mode")
                        n515 = global write "Robot Global Data.vi" "Elevator Bottom"(TRUE) -> ()
                        n516 = global read "Robot Global Data.vi" "Robot Travel Offset"() -> (w1808:dbl)
                        n517 = Wait (ms)(milliseconds to wait=u32 50) -> ()  [unwired: 1 out]
                        n518 = Multiply(x=303.5, y=217.294) -> (x*y=w1797:dbl)
                        n519 = Greater?(x=w1808, y=w1797) -> (0:w1807:bool)
                        n520 = Multiply(x=304.5 ("Output"), y=217.294) -> (x*y=w1794:dbl)
                        n521 = call <vilib>:"CTRE_Phoenix_MotorControl_Set.vi"("error in (no error)"=w1811, "Output"=w1794, "Control Mode"=w1813, "PhoenixMotorControlDevRef"=w1812) -> ("error out"=w1815:errorcluster, "PhoenixMotorControlDevRef"=w1814:T2)  [unwired: 6 in]
                        n522 = call <vilib>:"CTRE_Phoenix_MotorControl_Set.vi"("error in (no error)"=w1802, "Output"=w1794, "Control Mode"=w1804, "PhoenixMotorControlDevRef"=w1803) -> ("error out"=w1806:errorcluster, "PhoenixMotorControlDevRef"=w1805:T2)  [unwired: 6 in]
                        n523 = call-poly <vilib>:"CTRE_Phoenix_MotorController_Get_Enhanced.vi"("PhoenixMotorControlDevRef"=w1814, "error in"=w1815) -> ("PhoenixMotorControlDevRef"=w1810:T2, "error out"=w1809:errorcluster)  [unwired: 8 in, 4 out]
                        n524 = call-poly <vilib>:"CTRE_Phoenix_MotorController_Get_Enhanced.vi"("PhoenixMotorControlDevRef"=w1805, "error in"=w1806) -> ("PhoenixMotorControlDevRef"=w1801:T2, "error out"=w1800:errorcluster)  [unwired: 8 in, 4 out]
                      }
                    }
                    frame #1 {
                      n525 = while {
                        tunnel: w1825 -> [w1842]
                        tunnel: w1824 -> [w1841]
                        tunnel: [w1840] -> w1823
                        tunnel: [w1839] -> w1822
                        tunnel: [w1835] -> w1821
                        tunnel: [w1834] -> w1820
                        tunnel: w1819 -> [w1833]
                        tunnel: w1818 -> [w1832]
                        stop <- w1831 stop-if-true
                        w1836 = T12 7 items=["PercentOutput"=0, "Position"=1, "Velocity"=2, "Current"=3, "Follower"=5, "MotionProfile"=6, "MotionMagic"=7, "MotionMagicArc"=8, "MotionProfileArc"=10, "Disabled"=15] ("Control Mode")
                        w1843 = T12 7 items=["PercentOutput"=0, "Position"=1, "Velocity"=2, "Current"=3, "Follower"=5, "MotionProfile"=6, "MotionMagic"=7, "MotionMagicArc"=8, "MotionProfileArc"=10, "Disabled"=15] ("Control Mode")
                        n526 = global read "Robot Global Data.vi" "Robot Yaw Offset"() -> (w1829:dbl)
                        n527 = Wait (ms)(milliseconds to wait=u32 50) -> ()  [unwired: 1 out]
                        n528 = Less?(x=w1829, y=-90) -> (x < y?=w1831:bool)
                        n529 = Multiply(x=304.5 ("Output"), y=217.294) -> (x*y=w1826:dbl)
                        n530 = call <vilib>:"CTRE_Phoenix_MotorControl_Set.vi"("error in (no error)"=w1832, "Output"=w1826, "Control Mode"=w1836, "PhoenixMotorControlDevRef"=w1833) -> ("error out"=w1838:errorcluster, "PhoenixMotorControlDevRef"=w1837:T2)  [unwired: 6 in]
                        n531 = call <vilib>:"CTRE_Phoenix_MotorControl_Set.vi"("error in (no error)"=w1841, "Output"=w1826, "Control Mode"=w1843, "PhoenixMotorControlDevRef"=w1842) -> ("error out"=w1845:errorcluster, "PhoenixMotorControlDevRef"=w1844:T2)  [unwired: 6 in]
                        n532 = call-poly <vilib>:"CTRE_Phoenix_MotorController_Get_Enhanced.vi"("PhoenixMotorControlDevRef"=w1837, "error in"=w1838) -> ("PhoenixMotorControlDevRef"=w1835:T2, "error out"=w1834:errorcluster)  [unwired: 8 in, 4 out]
                        n533 = call-poly <vilib>:"CTRE_Phoenix_MotorController_Get_Enhanced.vi"("PhoenixMotorControlDevRef"=w1844, "error in"=w1845) -> ("PhoenixMotorControlDevRef"=w1840:T2, "error out"=w1839:errorcluster)  [unwired: 8 in, 4 out]
                      }
                    }
                    frame #2 {
                      n534 = while {
                        tunnel: w1854 -> [w1873]
                        tunnel: w1853 -> [w1872]
                        tunnel: [w1869] -> w1850
                        tunnel: [w1868] -> w1848
                        tunnel: [w1864] -> w1849
                        tunnel: [w1863] -> w1847
                        tunnel: w1852 -> [w1862]
                        tunnel: w1851 -> [w1861]
                        stop <- w1870 stop-if-true
                        w1865 = T12 7 items=["PercentOutput"=0, "Position"=1, "Velocity"=2, "Current"=3, "Follower"=5, "MotionProfile"=6, "MotionMagic"=7, "MotionMagicArc"=8, "MotionProfileArc"=10, "Disabled"=15] ("Control Mode")
                        w1874 = T12 7 items=["PercentOutput"=0, "Position"=1, "Velocity"=2, "Current"=3, "Follower"=5, "MotionProfile"=6, "MotionMagic"=7, "MotionMagicArc"=8, "MotionProfileArc"=10, "Disabled"=15] ("Control Mode")
                        n535 = global read "Robot Global Data.vi" "Robot Travel Offset"() -> (w1871:dbl)
                        n536 = Wait (ms)(milliseconds to wait=u32 50) -> ()  [unwired: 1 out]
                        n537 = Multiply(x=308.5, y=217.294) -> (x*y=w1855:dbl)
                        n538 = Greater?(x=w1871, y=w1855) -> (0:w1870:bool)
                        n539 = Multiply(x=309.5 ("Output"), y=217.294) -> (x*y=w1857:dbl)
                        n540 = call <vilib>:"CTRE_Phoenix_MotorControl_Set.vi"("error in (no error)"=w1861, "Output"=w1857, "Control Mode"=w1865, "PhoenixMotorControlDevRef"=w1862) -> ("error out"=w1867:errorcluster, "PhoenixMotorControlDevRef"=w1866:T2)  [unwired: 6 in]
                        n541 = call <vilib>:"CTRE_Phoenix_MotorControl_Set.vi"("error in (no error)"=w1872, "Output"=w1857, "Control Mode"=w1874, "PhoenixMotorControlDevRef"=w1873) -> ("error out"=w1876:errorcluster, "PhoenixMotorControlDevRef"=w1875:T2)  [unwired: 6 in]
                        n542 = call-poly <vilib>:"CTRE_Phoenix_MotorController_Get_Enhanced.vi"("PhoenixMotorControlDevRef"=w1866, "error in"=w1867) -> ("PhoenixMotorControlDevRef"=w1864:T2, "error out"=w1863:errorcluster)  [unwired: 8 in, 4 out]
                        n543 = call-poly <vilib>:"CTRE_Phoenix_MotorController_Get_Enhanced.vi"("PhoenixMotorControlDevRef"=w1875, "error in"=w1876) -> ("PhoenixMotorControlDevRef"=w1869:T2, "error out"=w1868:errorcluster)  [unwired: 8 in, 4 out]
                      }
                    }
                    frame #3 {
                      n544 = while {
                        tunnel: w1881 -> [w1903]
                        tunnel: w1879 -> [w1902]
                        tunnel: [w1901] -> w1885
                        tunnel: [w1900] -> w1884
                        tunnel: w1880 -> [w1896]
                        tunnel: w1878 -> [w1895]
                        tunnel: [w1894] -> w1883
                        tunnel: [w1893] -> w1882
                        i -> [w1890]
                        stop <- w1889 stop-if-true
                        w1897 = T12 7 items=["PercentOutput"=0, "Position"=1, "Velocity"=2, "Current"=3, "Follower"=5, "MotionProfile"=6, "MotionMagic"=7, "MotionMagicArc"=8, "MotionProfileArc"=10, "Disabled"=15] ("Control Mode")
                        w1904 = T12 7 items=["PercentOutput"=0, "Position"=1, "Velocity"=2, "Current"=3, "Follower"=5, "MotionProfile"=6, "MotionMagic"=7, "MotionMagicArc"=8, "MotionProfileArc"=10, "Disabled"=15] ("Control Mode")
                        # "ADD INTAKE/ELEVATOR CODE HERE"
                        n545 = Wait (ms)(milliseconds to wait=u32 50) -> ()  [unwired: 1 out]
                        n546 = Increment(x=w1890) -> (x+1=w1891:i32)
                        n547 = Greater Or Equal?(x=w1891, y=20) -> (x >= y?=w1889:bool)
                        n548 = Multiply(x=107.0 ("Output"), y=217.294) -> (x*y=w1886:dbl)
                        n549 = call <vilib>:"CTRE_Phoenix_MotorControl_Set.vi"("error in (no error)"=w1895, "Output"=w1886, "Control Mode"=w1897, "PhoenixMotorControlDevRef"=w1896) -> ("error out"=w1899:errorcluster, "PhoenixMotorControlDevRef"=w1898:T2)  [unwired: 6 in]
                        n550 = call <vilib>:"CTRE_Phoenix_MotorControl_Set.vi"("error in (no error)"=w1902, "Output"=w1886, "Control Mode"=w1904, "PhoenixMotorControlDevRef"=w1903) -> ("error out"=w1906:errorcluster, "PhoenixMotorControlDevRef"=w1905:T2)  [unwired: 6 in]
                        n551 = call-poly <vilib>:"CTRE_Phoenix_MotorController_Get_Enhanced.vi"("PhoenixMotorControlDevRef"=w1898, "error in"=w1899) -> ("PhoenixMotorControlDevRef"=w1894:T2, "error out"=w1893:errorcluster)  [unwired: 8 in, 4 out]
                        n552 = call-poly <vilib>:"CTRE_Phoenix_MotorController_Get_Enhanced.vi"("PhoenixMotorControlDevRef"=w1905, "error in"=w1906) -> ("PhoenixMotorControlDevRef"=w1901:T2, "error out"=w1900:errorcluster)  [unwired: 8 in, 4 out]
                      }
                    }
                    frame #4 {
                      n553 = while {
                        tunnel: w1911 -> [w1922]
                        tunnel: w1910 -> [w1921]
                        tunnel: w1909 -> [w1919]
                        tunnel: w1908 -> [w1918]
                        i -> [w1913]
                        stop <- w1912 stop-if-true
                        w1920 = T12 0 items=["PercentOutput"=0, "Position"=1, "Velocity"=2, "Current"=3, "Follower"=5, "MotionProfile"=6, "MotionMagic"=7, "MotionMagicArc"=8, "MotionProfileArc"=10, "Disabled"=15] ("Control Mode")
                        w1923 = T12 0 items=["PercentOutput"=0, "Position"=1, "Velocity"=2, "Current"=3, "Follower"=5, "MotionProfile"=6, "MotionMagic"=7, "MotionMagicArc"=8, "MotionProfileArc"=10, "Disabled"=15] ("Control Mode")
                        n554 = Increment(x=w1913) -> (x+1=w1914:i32)
                        n555 = Wait (ms)(milliseconds to wait=u32 15000) -> ()  [unwired: 1 out]
                        n556 = Greater Or Equal?(x=w1914, y=1) -> (x >= y?=w1912:bool)
                        n557 = call <vilib>:"CTRE_Phoenix_MotorControl_Set.vi"("error in (no error)"=w1918, "Output"=0.0, "Control Mode"=w1920, "PhoenixMotorControlDevRef"=w1919) -> ()  [unwired: 6 in, 2 out]
                        n558 = call <vilib>:"CTRE_Phoenix_MotorControl_Set.vi"("error in (no error)"=w1921, "Output"=0.0, "Control Mode"=w1923, "PhoenixMotorControlDevRef"=w1922) -> ()  [unwired: 6 in, 2 out]
                      }
                    }
                  }
                }
                frame Default {
                }
                frame "L" {
                  # "Drive straight"
                  n559 = flat-sequence {
                    tunnel: w1928 -> [w1964]
                    tunnel: w1927 -> [w1963]
                    tunnel: [w1962] -> w1956
                    tunnel: [w1961] -> w1955
                    tunnel: w1926 -> [w1960]
                    tunnel: w1925 -> [w1959]
                    tunnel: [w1958] -> w1954
                    tunnel: [w1957] -> w1953
                    tunnel: w1956 -> [w1996]
                    tunnel: w1955 -> [w1995]
                    tunnel: [w1994] -> w1952
                    tunnel: [w1993] -> w1951
                    tunnel: [w1992] -> w1950
                    tunnel: [w1991] -> w1949
                    tunnel: w1954 -> [w1990]
                    tunnel: w1953 -> [w1989]
                    tunnel: w1952 -> [w2025]
                    tunnel: w1951 -> [w2024]
                    tunnel: [w2023] -> w1948
                    tunnel: [w2022] -> w1947
                    tunnel: [w2021] -> w1946
                    tunnel: [w2020] -> w1945
                    tunnel: w1950 -> [w2019]
                    tunnel: w1949 -> [w2018]
                    tunnel: w1948 -> [w2056]
                    tunnel: w1947 -> [w2055]
                    tunnel: [w2054] -> w1944
                    tunnel: [w2053] -> w1943
                    tunnel: [w2052] -> w1942
                    tunnel: [w2051] -> w1941
                    tunnel: w1946 -> [w2050]
                    tunnel: w1945 -> [w2049]
                    tunnel: w1944 -> [w2085]
                    tunnel: w1943 -> [w2084]
                    tunnel: [w2083] -> w1940
                    tunnel: [w2082] -> w1939
                    tunnel: w1942 -> [w2081]
                    tunnel: w1941 -> [w2080]
                    tunnel: [w2079] -> w1938
                    tunnel: [w2078] -> w1937
                    tunnel: w1940 -> [w2116]
                    tunnel: w1939 -> [w2115]
                    tunnel: w1938 -> [w2114]
                    tunnel: w1937 -> [w2113]
                    tunnel: [w2112] -> w1936
                    tunnel: [w2111] -> w1935
                    tunnel: [w2110] -> w1934
                    tunnel: [w2109] -> w1933
                    tunnel: [w2145] -> w1932
                    tunnel: [w2144] -> w1931
                    tunnel: [w2143] -> w1930
                    tunnel: [w2142] -> w1929
                    tunnel: w1936 -> [w2141]
                    tunnel: w1935 -> [w2140]
                    tunnel: w1934 -> [w2139]
                    tunnel: w1933 -> [w2138]
                    tunnel: w1932 -> [w2171]
                    tunnel: w1931 -> [w2170]
                    tunnel: w1930 -> [w2169]
                    tunnel: w1929 -> [w2168]
                    frame #0 {
                      n560 = while {
                        tunnel: w1964 -> [w1983]
                        tunnel: w1963 -> [w1982]
                        tunnel: [w1981] -> w1962
                        tunnel: [w1980] -> w1961
                        tunnel: w1960 -> [w1974]
                        tunnel: w1959 -> [w1973]
                        tunnel: [w1972] -> w1958
                        tunnel: [w1971] -> w1957
                        stop <- w1978 stop-if-true
                        w1975 = T12 7 items=["PercentOutput"=0, "Position"=1, "Velocity"=2, "Current"=3, "Follower"=5, "MotionProfile"=6, "MotionMagic"=7, "MotionMagicArc"=8, "MotionProfileArc"=10, "Disabled"=15] ("Control Mode")
                        w1984 = T12 7 items=["PercentOutput"=0, "Position"=1, "Velocity"=2, "Current"=3, "Follower"=5, "MotionProfile"=6, "MotionMagic"=7, "MotionMagicArc"=8, "MotionProfileArc"=10, "Disabled"=15] ("Control Mode")
                        n561 = global write "Robot Global Data.vi" "Elevator Bottom"(TRUE) -> ()
                        n562 = global read "Robot Global Data.vi" "Robot Travel Offset"() -> (w1979:dbl)
                        n563 = Wait (ms)(milliseconds to wait=u32 50) -> ()  [unwired: 1 out]
                        n564 = Multiply(x=214.75, y=217.294) -> (x*y=w1967:dbl)
                        n565 = Greater?(x=w1979, y=w1967) -> (0:w1978:bool)
                        n566 = Multiply(x=215.75 ("Output"), y=217.294) -> (x*y=w1965:dbl)
                        n567 = call <vilib>:"CTRE_Phoenix_MotorControl_Set.vi"("error in (no error)"=w1982, "Output"=w1965, "Control Mode"=w1984, "PhoenixMotorControlDevRef"=w1983) -> ("error out"=w1986:errorcluster, "PhoenixMotorControlDevRef"=w1985:T2)  [unwired: 6 in]
                        n568 = call <vilib>:"CTRE_Phoenix_MotorControl_Set.vi"("error in (no error)"=w1973, "Output"=w1965, "Control Mode"=w1975, "PhoenixMotorControlDevRef"=w1974) -> ("error out"=w1977:errorcluster, "PhoenixMotorControlDevRef"=w1976:T2)  [unwired: 6 in]
                        n569 = call-poly <vilib>:"CTRE_Phoenix_MotorController_Get_Enhanced.vi"("PhoenixMotorControlDevRef"=w1985, "error in"=w1986) -> ("PhoenixMotorControlDevRef"=w1981:T2, "error out"=w1980:errorcluster)  [unwired: 8 in, 4 out]
                        n570 = call-poly <vilib>:"CTRE_Phoenix_MotorController_Get_Enhanced.vi"("PhoenixMotorControlDevRef"=w1976, "error in"=w1977) -> ("PhoenixMotorControlDevRef"=w1972:T2, "error out"=w1971:errorcluster)  [unwired: 8 in, 4 out]
                      }
                    }
                    frame #1 {
                      n571 = while {
                        tunnel: w1996 -> [w2013]
                        tunnel: w1995 -> [w2012]
                        tunnel: [w2011] -> w1994
                        tunnel: [w2010] -> w1993
                        tunnel: [w2006] -> w1992
                        tunnel: [w2005] -> w1991
                        tunnel: w1990 -> [w2004]
                        tunnel: w1989 -> [w2003]
                        stop <- w2002 stop-if-true
                        w2007 = T12 7 items=["PercentOutput"=0, "Position"=1, "Velocity"=2, "Current"=3, "Follower"=5, "MotionProfile"=6, "MotionMagic"=7, "MotionMagicArc"=8, "MotionProfileArc"=10, "Disabled"=15] ("Control Mode")
                        w2014 = T12 7 items=["PercentOutput"=0, "Position"=1, "Velocity"=2, "Current"=3, "Follower"=5, "MotionProfile"=6, "MotionMagic"=7, "MotionMagicArc"=8, "MotionProfileArc"=10, "Disabled"=15] ("Control Mode")
                        n572 = global read "Robot Global Data.vi" "Robot Yaw Offset"() -> (w2000:dbl)
                        n573 = Wait (ms)(milliseconds to wait=u32 50) -> ()  [unwired: 1 out]
                        n574 = Less?(x=w2000, y=-90) -> (x < y?=w2002:bool)
                        n575 = Multiply(x=215.75 ("Output"), y=217.294) -> (x*y=w1997:dbl)
                        n576 = call <vilib>:"CTRE_Phoenix_MotorControl_Set.vi"("error in (no error)"=w2003, "Output"=w1997, "Control Mode"=w2007, "PhoenixMotorControlDevRef"=w2004) -> ("error out"=w2009:errorcluster, "PhoenixMotorControlDevRef"=w2008:T2)  [unwired: 6 in]
                        n577 = call <vilib>:"CTRE_Phoenix_MotorControl_Set.vi"("error in (no error)"=w2012, "Output"=w1997, "Control Mode"=w2014, "PhoenixMotorControlDevRef"=w2013) -> ("error out"=w2016:errorcluster, "PhoenixMotorControlDevRef"=w2015:T2)  [unwired: 6 in]
                        n578 = call-poly <vilib>:"CTRE_Phoenix_MotorController_Get_Enhanced.vi"("PhoenixMotorControlDevRef"=w2008, "error in"=w2009) -> ("PhoenixMotorControlDevRef"=w2006:T2, "error out"=w2005:errorcluster)  [unwired: 8 in, 4 out]
                        n579 = call-poly <vilib>:"CTRE_Phoenix_MotorController_Get_Enhanced.vi"("PhoenixMotorControlDevRef"=w2015, "error in"=w2016) -> ("PhoenixMotorControlDevRef"=w2011:T2, "error out"=w2010:errorcluster)  [unwired: 8 in, 4 out]
                      }
                    }
                    frame #2 {
                      n580 = while {
                        tunnel: w2025 -> [w2044]
                        tunnel: w2024 -> [w2043]
                        tunnel: [w2040] -> w2023
                        tunnel: [w2039] -> w2022
                        tunnel: [w2035] -> w2021
                        tunnel: [w2034] -> w2020
                        tunnel: w2019 -> [w2033]
                        tunnel: w2018 -> [w2032]
                        stop <- w2041 stop-if-true
                        w2036 = T12 7 items=["PercentOutput"=0, "Position"=1, "Velocity"=2, "Current"=3, "Follower"=5, "MotionProfile"=6, "MotionMagic"=7, "MotionMagicArc"=8, "MotionProfileArc"=10, "Disabled"=15] ("Control Mode")
                        w2045 = T12 7 items=["PercentOutput"=0, "Position"=1, "Velocity"=2, "Current"=3, "Follower"=5, "MotionProfile"=6, "MotionMagic"=7, "MotionMagicArc"=8, "MotionProfileArc"=10, "Disabled"=15] ("Control Mode")
                        n581 = global read "Robot Global Data.vi" "Robot Travel Offset"() -> (w2042:dbl)
                        n582 = Wait (ms)(milliseconds to wait=u32 50) -> ()  [unwired: 1 out]
                        n583 = Multiply(x=440.75 ("Output"), y=217.294) -> (x*y=w2026:dbl)
                        n584 = call <vilib>:"CTRE_Phoenix_MotorControl_Set.vi"("error in (no error)"=w2032, "Output"=w2026, "Control Mode"=w2036, "PhoenixMotorControlDevRef"=w2033) -> ("error out"=w2038:errorcluster, "PhoenixMotorControlDevRef"=w2037:T2)  [unwired: 6 in]
                        n585 = call <vilib>:"CTRE_Phoenix_MotorControl_Set.vi"("error in (no error)"=w2043, "Output"=w2026, "Control Mode"=w2045, "PhoenixMotorControlDevRef"=w2044) -> ("error out"=w2047:errorcluster, "PhoenixMotorControlDevRef"=w2046:T2)  [unwired: 6 in]
                        n586 = call-poly <vilib>:"CTRE_Phoenix_MotorController_Get_Enhanced.vi"("PhoenixMotorControlDevRef"=w2037, "error in"=w2038) -> ("PhoenixMotorControlDevRef"=w2035:T2, "error out"=w2034:errorcluster)  [unwired: 8 in, 4 out]
                        n587 = call-poly <vilib>:"CTRE_Phoenix_MotorController_Get_Enhanced.vi"("PhoenixMotorControlDevRef"=w2046, "error in"=w2047) -> ("PhoenixMotorControlDevRef"=w2040:T2, "error out"=w2039:errorcluster)  [unwired: 8 in, 4 out]
                        n588 = Multiply(x=439.75, y=217.294) -> (x*y=w2029:dbl)
                        n589 = Greater?(x=w2042, y=w2029) -> (0:w2041:bool)
                      }
                    }
                    frame #3 {
                      n590 = while {
                        tunnel: w2056 -> [w2073]
                        tunnel: w2055 -> [w2072]
                        tunnel: [w2071] -> w2054
                        tunnel: [w2070] -> w2053
                        tunnel: [w2066] -> w2052
                        tunnel: [w2065] -> w2051
                        tunnel: w2050 -> [w2064]
                        tunnel: w2049 -> [w2063]
                        stop <- w2060 stop-if-true
                        w2067 = T12 7 items=["PercentOutput"=0, "Position"=1, "Velocity"=2, "Current"=3, "Follower"=5, "MotionProfile"=6, "MotionMagic"=7, "MotionMagicArc"=8, "MotionProfileArc"=10, "Disabled"=15] ("Control Mode")
                        w2074 = T12 7 items=["PercentOutput"=0, "Position"=1, "Velocity"=2, "Current"=3, "Follower"=5, "MotionProfile"=6, "MotionMagic"=7, "MotionMagicArc"=8, "MotionProfileArc"=10, "Disabled"=15] ("Control Mode")
                        n591 = global read "Robot Global Data.vi" "Robot Yaw Offset"() -> (w2061:dbl)
                        n592 = Wait (ms)(milliseconds to wait=u32 50) -> ()  [unwired: 1 out]
                        n593 = Greater?(x=w2061, y=0) -> (0:w2060:bool)
                        n594 = Multiply(x=440.75 ("Output"), y=217.294) -> (x*y=w2057:dbl)
                        n595 = call <vilib>:"CTRE_Phoenix_MotorControl_Set.vi"("error in (no error)"=w2063, "Output"=w2057, "Control Mode"=w2067, "PhoenixMotorControlDevRef"=w2064) -> ("error out"=w2069:errorcluster, "PhoenixMotorControlDevRef"=w2068:T2)  [unwired: 6 in]
                        n596 = call <vilib>:"CTRE_Phoenix_MotorControl_Set.vi"("error in (no error)"=w2072, "Output"=w2057, "Control Mode"=w2074, "PhoenixMotorControlDevRef"=w2073) -> ("error out"=w2076:errorcluster, "PhoenixMotorControlDevRef"=w2075:T2)  [unwired: 6 in]
                        n597 = call-poly <vilib>:"CTRE_Phoenix_MotorController_Get_Enhanced.vi"("PhoenixMotorControlDevRef"=w2068, "error in"=w2069) -> ("PhoenixMotorControlDevRef"=w2066:T2, "error out"=w2065:errorcluster)  [unwired: 8 in, 4 out]
                        n598 = call-poly <vilib>:"CTRE_Phoenix_MotorController_Get_Enhanced.vi"("PhoenixMotorControlDevRef"=w2075, "error in"=w2076) -> ("PhoenixMotorControlDevRef"=w2071:T2, "error out"=w2070:errorcluster)  [unwired: 8 in, 4 out]
                      }
                    }
                    frame #4 {
                      n599 = while {
                        tunnel: w2085 -> [w2104]
                        tunnel: w2084 -> [w2103]
                        tunnel: [w2100] -> w2083
                        tunnel: [w2099] -> w2082
                        tunnel: w2081 -> [w2095]
                        tunnel: w2080 -> [w2094]
                        tunnel: [w2093] -> w2079
                        tunnel: [w2092] -> w2078
                        stop <- w2101 stop-if-true
                        w2096 = T12 7 items=["PercentOutput"=0, "Position"=1, "Velocity"=2, "Current"=3, "Follower"=5, "MotionProfile"=6, "MotionMagic"=7, "MotionMagicArc"=8, "MotionProfileArc"=10, "Disabled"=15] ("Control Mode")
                        w2105 = T12 7 items=["PercentOutput"=0, "Position"=1, "Velocity"=2, "Current"=3, "Follower"=5, "MotionProfile"=6, "MotionMagic"=7, "MotionMagicArc"=8, "MotionProfileArc"=10, "Disabled"=15] ("Control Mode")
                        n600 = global read "Robot Global Data.vi" "Robot Travel Offset"() -> (w2102:dbl)
                        n601 = Wait (ms)(milliseconds to wait=u32 50) -> ()  [unwired: 1 out]
                        n602 = Multiply(x=528.5, y=217.294) -> (x*y=w2086:dbl)
                        n603 = Greater?(x=w2102, y=w2086) -> (0:w2101:bool)
                        n604 = Multiply(x=529.5 ("Output"), y=217.294) -> (x*y=w2088:dbl)
                        n605 = call <vilib>:"CTRE_Phoenix_MotorControl_Set.vi"("error in (no error)"=w2094, "Output"=w2088, "Control Mode"=w2096, "PhoenixMotorControlDevRef"=w2095) -> ("error out"=w2098:errorcluster, "PhoenixMotorControlDevRef"=w2097:T2)  [unwired: 6 in]
                        n606 = call <vilib>:"CTRE_Phoenix_MotorControl_Set.vi"("error in (no error)"=w2103, "Output"=w2088, "Control Mode"=w2105, "PhoenixMotorControlDevRef"=w2104) -> ("error out"=w2107:errorcluster, "PhoenixMotorControlDevRef"=w2106:T2)  [unwired: 6 in]
                        n607 = call-poly <vilib>:"CTRE_Phoenix_MotorController_Get_Enhanced.vi"("PhoenixMotorControlDevRef"=w2097, "error in"=w2098) -> ("PhoenixMotorControlDevRef"=w2093:T2, "error out"=w2092:errorcluster)  [unwired: 8 in, 4 out]
                        n608 = call-poly <vilib>:"CTRE_Phoenix_MotorController_Get_Enhanced.vi"("PhoenixMotorControlDevRef"=w2106, "error in"=w2107) -> ("PhoenixMotorControlDevRef"=w2100:T2, "error out"=w2099:errorcluster)  [unwired: 8 in, 4 out]
                      }
                    }
                    frame #5 {
                      n609 = while {
                        tunnel: w2116 -> [w2133]
                        tunnel: w2115 -> [w2132]
                        tunnel: [w2131] -> w2112
                        tunnel: [w2130] -> w2111
                        tunnel: [w2126] -> w2110
                        tunnel: [w2125] -> w2109
                        tunnel: w2114 -> [w2124]
                        tunnel: w2113 -> [w2123]
                        stop <- w2120 stop-if-true
                        w2127 = T12 7 items=["PercentOutput"=0, "Position"=1, "Velocity"=2, "Current"=3, "Follower"=5, "MotionProfile"=6, "MotionMagic"=7, "MotionMagicArc"=8, "MotionProfileArc"=10, "Disabled"=15] ("Control Mode")
                        w2134 = T12 7 items=["PercentOutput"=0, "Position"=1, "Velocity"=2, "Current"=3, "Follower"=5, "MotionProfile"=6, "MotionMagic"=7, "MotionMagicArc"=8, "MotionProfileArc"=10, "Disabled"=15] ("Control Mode")
                        n610 = global read "Robot Global Data.vi" "Robot Yaw Offset"() -> (w2121:dbl)
                        n611 = Wait (ms)(milliseconds to wait=u32 50) -> ()  [unwired: 1 out]
                        n612 = Greater?(x=w2121, y=90) -> (0:w2120:bool)
                        n613 = Multiply(x=529.5 ("Output"), y=217.294) -> (x*y=w2117:dbl)
                        n614 = call <vilib>:"CTRE_Phoenix_MotorControl_Set.vi"("error in (no error)"=w2123, "Output"=w2117, "Control Mode"=w2127, "PhoenixMotorControlDevRef"=w2124) -> ("error out"=w2129:errorcluster, "PhoenixMotorControlDevRef"=w2128:T2)  [unwired: 6 in]
                        n615 = call <vilib>:"CTRE_Phoenix_MotorControl_Set.vi"("error in (no error)"=w2132, "Output"=w2117, "Control Mode"=w2134, "PhoenixMotorControlDevRef"=w2133) -> ("error out"=w2136:errorcluster, "PhoenixMotorControlDevRef"=w2135:T2)  [unwired: 6 in]
                        n616 = call-poly <vilib>:"CTRE_Phoenix_MotorController_Get_Enhanced.vi"("PhoenixMotorControlDevRef"=w2128, "error in"=w2129) -> ("PhoenixMotorControlDevRef"=w2126:T2, "error out"=w2125:errorcluster)  [unwired: 8 in, 4 out]
                        n617 = call-poly <vilib>:"CTRE_Phoenix_MotorController_Get_Enhanced.vi"("PhoenixMotorControlDevRef"=w2135, "error in"=w2136) -> ("PhoenixMotorControlDevRef"=w2131:T2, "error out"=w2130:errorcluster)  [unwired: 8 in, 4 out]
                      }
                    }
                    frame #6 {
                      n618 = while {
                        tunnel: [w2163] -> w2145
                        tunnel: [w2162] -> w2144
                        tunnel: [w2158] -> w2143
                        tunnel: [w2157] -> w2142
                        tunnel: w2141 -> [w2156]
                        tunnel: w2140 -> [w2155]
                        tunnel: w2139 -> [w2154]
                        tunnel: w2138 -> [w2153]
                        i -> [w2150]
                        stop <- w2149 stop-if-true
                        w2159 = T12 7 items=["PercentOutput"=0, "Position"=1, "Velocity"=2, "Current"=3, "Follower"=5, "MotionProfile"=6, "MotionMagic"=7, "MotionMagicArc"=8, "MotionProfileArc"=10, "Disabled"=15] ("Control Mode")
                        w2164 = T12 7 items=["PercentOutput"=0, "Position"=1, "Velocity"=2, "Current"=3, "Follower"=5, "MotionProfile"=6, "MotionMagic"=7, "MotionMagicArc"=8, "MotionProfileArc"=10, "Disabled"=15] ("Control Mode")
                        # "ADD INTAKE/ELEVATOR CODE HERE"
                        n619 = Increment(x=w2150) -> (x+1=w2151:i32)
                        n620 = Wait (ms)(milliseconds to wait=u32 50) -> ()  [unwired: 1 out]
                        n621 = Greater Or Equal?(x=w2151, y=20) -> (x >= y?=w2149:bool)
                        n622 = Multiply(x=529.5 ("Output"), y=217.294) -> (x*y=w2146:dbl)
                        n623 = call <vilib>:"CTRE_Phoenix_MotorControl_Set.vi"("error in (no error)"=w2153, "Output"=w2146, "Control Mode"=w2159, "PhoenixMotorControlDevRef"=w2154) -> ("error out"=w2161:errorcluster, "PhoenixMotorControlDevRef"=w2160:T2)  [unwired: 6 in]
                        n624 = call <vilib>:"CTRE_Phoenix_MotorControl_Set.vi"("error in (no error)"=w2155, "Output"=w2146, "Control Mode"=w2164, "PhoenixMotorControlDevRef"=w2156) -> ("error out"=w2166:errorcluster, "PhoenixMotorControlDevRef"=w2165:T2)  [unwired: 6 in]
                        n625 = call-poly <vilib>:"CTRE_Phoenix_MotorController_Get_Enhanced.vi"("PhoenixMotorControlDevRef"=w2160, "error in"=w2161) -> ("PhoenixMotorControlDevRef"=w2158:T2, "error out"=w2157:errorcluster)  [unwired: 8 in, 4 out]
                        n626 = call-poly <vilib>:"CTRE_Phoenix_MotorController_Get_Enhanced.vi"("PhoenixMotorControlDevRef"=w2165, "error in"=w2166) -> ("PhoenixMotorControlDevRef"=w2163:T2, "error out"=w2162:errorcluster)  [unwired: 8 in, 4 out]
                      }
                    }
                    frame #7 {
                      n627 = while {
                        tunnel: w2171 -> [w2182]
                        tunnel: w2170 -> [w2181]
                        tunnel: w2169 -> [w2179]
                        tunnel: w2168 -> [w2178]
                        i -> [w2172]
                        stop <- w2173 stop-if-true
                        w2180 = T12 0 items=["PercentOutput"=0, "Position"=1, "Velocity"=2, "Current"=3, "Follower"=5, "MotionProfile"=6, "MotionMagic"=7, "MotionMagicArc"=8, "MotionProfileArc"=10, "Disabled"=15] ("Control Mode")
                        w2183 = T12 0 items=["PercentOutput"=0, "Position"=1, "Velocity"=2, "Current"=3, "Follower"=5, "MotionProfile"=6, "MotionMagic"=7, "MotionMagicArc"=8, "MotionProfileArc"=10, "Disabled"=15] ("Control Mode")
                        n628 = Increment(x=w2172) -> (x+1=w2174:i32)
                        n629 = Wait (ms)(milliseconds to wait=u32 15000) -> ()  [unwired: 1 out]
                        n630 = call <vilib>:"CTRE_Phoenix_MotorControl_Set.vi"("error in (no error)"=w2178, "Output"=0.0, "Control Mode"=w2180, "PhoenixMotorControlDevRef"=w2179) -> ()  [unwired: 6 in, 2 out]
                        n631 = Greater Or Equal?(x=w2174, y=1) -> (x >= y?=w2173:bool)
                        n632 = call <vilib>:"CTRE_Phoenix_MotorControl_Set.vi"("error in (no error)"=w2181, "Output"=0.0, "Control Mode"=w2183, "PhoenixMotorControlDevRef"=w2182) -> ()  [unwired: 6 in, 2 out]
                      }
                    }
                  }
                }
              }
            }
          }
        }
      }
    }
  }
